vi "rsidr_core_global.vi"() -> ()   [LabVIEW 2015, in "Rohde&Schwarz CMP LR WPAN Measurement.lvlib"]
doc: "This Global variable contains driver's:\n- Attributes\n- Range Tables\n- Repeated Capabilities"
uses:
  <instrlib>/Rohde&Schwarz CMP LR WPAN Measurement/Rohde&Schwarz CMP LR WPAN Measurement.lvlib
  <instrlib>/Rohde&Schwarz CMP LR WPAN Measurement/Private/rsidr_core.llb/type_Input_Format_Attribute.ctl
  <instrlib>/Rohde&Schwarz CMP LR WPAN Measurement/Private/rsidr_core.llb/type_Input_Format_RangeTable.ctl
  <instrlib>/Rohde&Schwarz CMP LR WPAN Measurement/Private/rsidr_core.llb/type_Input_Format_RepCap.ctl
  <instrlib>/Rohde&Schwarz CMP LR WPAN Measurement/Private/rsidr_core.llb/rsidr_core.lvlib
panel:
  in  "Repeated Capabilities":T1[](array[typedef])=[{"repCapName"="instance", "indetifiers"=["i0", "i1", "i2", "i3", "i4", "i5", "i6", "i7", "i8", "i9", "i10", "i11", "i12", "i13", "i14", "i15", "i16", "i17", "i18", "i19", "i20", "i21", "i22", "i23", "i24", "i25", "i26", "i27", "i28", "i29", "i30", "i31", "i32"], "cmdValues"=["", "1", "2", "3", "4", "5", "6", "7", "8", "9", "10", "11", "12", "13", "14", "15", "16", "17", "18", "19", "20", "21", "22", "23", "24", "25", "26", "27", "28", "29", "30", "31", "32"]}]
  in  "Range Tables":T2[](array[typedef])=[{"Type"=0, "Name"="rscmplrwm_rngExternalAttenuation", "Entries"=[{"Name"="", "Value 1"=-50.0, "Value 2"=90.0, "Command"=""}]}, {"Type"=0, "Name"="rscmplrwm_rngFrequency", "Entries"=[{"Name"="", "Value 1"=4000000000.0, "Value 2"=20000000000.0, "Command"=""}]}, {"Type"=2, "Name"="rscmplrwm_rngRepetitionMode", "Entries"=[{"Name"="Single shot measurement", "Value 1"=0.0, "Value 2"=0.0, "Command"="SING"}, {"Name"="Continuous measurement", "Value 1"=1.0, "Value 2"=0.0, "Command"="CONT"}]}, {"Type"=2, "Name"="rscmplrwm_rngMultiEvalStopCondition", "Entries"=[{"Name"="None", "Value 1"=0.0, "Value 2"=0.0, "Command"="NONE"}, {"Name"="LimitFailure", "Value 1"=1.0, "Value 2"=0.0, "Command"="SLF"}]}, {"Type"=0, "Name"="rscmplrwm_rngMultiEvalModulationStatisticCount", "Entries"=[{"Name"="", "Value 1"=1.0, "Value 2"=1000.0, "Command"=""}]}, {"Type"=0, "Name"="rscmplrwm_rngMultiEvalPowerStatisticCount", "Entries"=[{"Name"="", "Value 1"=1.0, "Value 2"=1000.0, "Command"=""}]}, {"Type"=0, "Name"="rscmplrwm_rngMultiEvalSpectrumStatisticCount", "Entries"=[{"Name"="", "Value 1"=1.0, "Value 2"=1000.0, "Command"=""}]}, {"Type"=0, "Name"="rscmplrwm_rngMultiEvalMinimumTriggerGap", "Entries"=[{"Name"="", "Value 1"=0.0, "Value 2"=0.01, "Command"=""}]}, {"Type"=0, "Name"="rscmplrwm_rngMultiEvalTriggerTimeout", "Entries"=[{"Name"="", "Value 1"=0.01, "Value 2"=167772.1, "Command"=""}]}, {"Type"=0, "Name"="rscmplrwm_rngMultiEvalTriggerThreshold", "Entries"=[{"Name"="", "Value 1"=-50.0, "Value 2"=0.0, "Command"=""}]}, {"Type"=2, "Name"="rscmplrwm_rngModulationType", "Entries"=[{"Name"="2450 MHz, OQPSK", "Value 1"=0.0, "Value 2"=0.0, "Command"="OQ24"}]}, {"Type"=2, "Name"="rscmplrwm_rngSignalPath", "Entries"=[{"Name"="Port1.IFIn", "Value 1"=1.0, "Value 2"=0.0, "Command"="\"Port1.IFIn\""}, {"Name"="Port2.IFIn", "Value 1"=2.0, "Value 2"=0.0, "Command"="\"Port2.IFIn\""}, {"Name"="Port3.IFIn", "Value 1"=3.0, "Value 2"=0.0, "Command"="\"Port3.IFIn\""}]}, {"Type"=2, "Name"="rscmplrwm_rngResultType", "Entries"=[{"Name"="Current", "Value 1"=0.0, "Value 2"=0.0, "Command"="CURR"}, {"Name"="Average", "Value 1"=1.0, "Value 2"=0.0, "Command"="AVER"}, {"Name"="Extreme", "Value 1"=2.0, "Value 2"=0.0, "Command"="EXT"}, {"Name"="Standard Deviation", "Value 1"=3.0, "Value 2"=0.0, "Command"="SDEV"}, {"Name"="Maximum", "Value 1"=4.0, "Value 2"=0.0, "Command"="MAX"}, {"Name"="Minimum", "Value 1"=5.0, "Value 2"=0.0, "Command"="MIN"}]}, {"Type"=2, "Name"="rscmplrwm_rngLimitCheckResults", "Entries"=[{"Name"="Pass", "Value 1"=0.0, "Value 2"=0.0, "Command"="OK"}, {"Name"="Failed Upper", "Value 1"=1.0, "Value 2"=0.0, "Command"="ULEU"}, {"Name"="Failed Lower", "Value 1"=2.0, "Value 2"=0.0, "Command"="ULEL"}, {"Name"="Overflow", "Value 1"=3.0, "Value 2"=0.0, "Command"="OFL"}, {"Name"="Underflow", "Value 1"=4.0, "Value 2"=0.0, "Command"="UFL"}, {"Name"="Invalid", "Value 1"=5.0, "Value 2"=0.0, "Command"="INV"}, {"Name"="Not A Value", "Value 1"=6.0, "Value 2"=0.0, "Command"="NAV"}, {"Name"="Off", "Value 1"=7.0, "Value 2"=0.0, "Command"="OFF"}, {"Name"="Not Capable", "Value 1"=8.0, "Value 2"=0.0, "Command"="NCAP"}]}, {"Type"=2, "Name"="rscmplrwm_rngSyncState", "Entries"=[{"Name"="Pending", "Value 1"=0.0, "Value 2"=0.0, "Command"="PEND"}, {"Name"="Adjusted", "Value 1"=1.0, "Value 2"=0.0, "Command"="ADJ"}, {"Name"="Invalid", "Value 1"=2.0, "Value 2"=0.0, "Command"="INV"}]}, {"Type"=2, "Name"="rscmplrwm_rngResourceState", "Entries"=[{"Name"="No Resources", "Value 1"=0.0, "Value 2"=0.0, "Command"="QUE"}, {"Name"="Active", "Value 1"=1.0, "Value 2"=0.0, "Command"="ACT"}, {"Name"="Invalid", "Value 1"=2.0, "Value 2"=0.0, "Command"="INV"}]}, {"Type"=2, "Name"="rscmplrwm_rngMainState", "Entries"=[{"Name"="Off", "Value 1"=0.0, "Value 2"=0.0, "Command"="OFF"}, {"Name"="Run", "Value 1"=1.0, "Value 2"=0.0, "Command"="RUN"}, {"Name"="Ready", "Value 1"=2.0, "Value 2"=0.0, "Command"="RDY"}]}] {"Type" items=["Range", "Coerced", "Discrete"]}
  in  "Attributes":T3[](array[typedef])=[{"Level"=1, "Class Only"=TRUE, "Identifier"="", "Descriptive Name"="Configuration", "Data Type"=0, "Command"="", "Access"=0, "Range Table"="", "Read Callback"="", "Write Callback"="", "Supported Models"="", "Instrument Options"="", "Flags"=0, "Help"="Contains attributes for configuring LR-WPAN Measurement."}, {"Level"=2, "Class Only"=FALSE, "Identifier"="RSCMPLRWM_ATTR_SIGNAL_PATH", "Descriptive Name"="Signal Path", "Data Type"=0, "Command"="ROUT:WPAN:MEAS{instance}:SPAT", "Access"=2, "Range Table"="rscmplrwm_rngSignalPath", "Read Callback"="", "Write Callback"="", "Supported Models"="", "Instrument Options"="", "Flags"=0, "Help"="Selects the signal path for the measured RF signal.\nValid Values: Port1.IFln, Port2.IFln, Port3.IFln\n\nAvailable Repeated Capabilities:\ninstance: i0, i1, i2, i3, i4, i5, i6, i7, i8, i9, i10, i11, i12, i13, i14, i15, i16, i17, i18, i19, i20, i21, i22, i23, i24, i25, i26, i27, i28, i29, i30, i31, i32\r\n\nRemote-control command(s):\nROUTe:WPAN:MEAS<i>:SPATh"}, {"Level"=2, "Class Only"=FALSE, "Identifier"="RSCMPLRWM_ATTR_SIGNAL_PATH_CATALOG", "Descriptive Name"="Signal Path Catalog", "Data Type"=2, "Command"="CAT:WPAN:MEAS{instance}:SPAT?", "Access"=0, "Range Table"="", "Read Callback"="", "Write Callback"="", "Supported Models"="", "Instrument Options"="", "Flags"=0, "Help"="Returns the names of the available signal paths.\n\nReturned values: Comma-separated list of strings, one string per signal path\n\nAvailable Repeated Capabilities:\ninstance: i0, i1, i2, i3, i4, i5, i6, i7, i8, i9, i10, i11, i12, i13, i14, i15, i16, i17, i18, i19, i20, i21, i22, i23, i24, i25, i26, i27, i28, i29, i30, i31, i32\r\n\nRemote-control command(s):\nCATalog:WPAN:MEAS<i>:SPATh<stream>?"}, {"Level"=2, "Class Only"=FALSE, "Identifier"="RSCMPLRWM_ATTR_FREQUENCY", "Descriptive Name"="Frequency", "Data Type"=1, "Command"="CONF:WPAN:MEAS{instance}:RFS:FREQ", "Access"=2, "Range Table"="rscmplrwm_rngFrequency", "Read Callback"="", "Write Callback"="", "Supported Models"="", "Instrument Options"="", "Flags"=0, "Help"="Selects the center frequency of the RF analyzer.\n\nAvailable Repeated Capabilities:\ninstance: i0, i1, i2, i3, i4, i5, i6, i7, i8, i9, i10, i11, i12, i13, i14, i15, i16, i17, i18, i19, i20, i21, i22, i23, i24, i25, i26, i27, i28, i29, i30, i31, i32\r\n\nRemote-control command(s):\nCONFigure:WPAN:MEAS<i>:RFSettings:FREQuency"}, {"Level"=2, "Class Only"=FALSE, "Identifier"="RSCMPLRWM_ATTR_EXPECTED_NOMINAL_POWER", "Descriptive Name"="Expected Nominal Power", "Data Type"=1, "Command"="CONF:WPAN:MEAS{instance}:RFS:ENP", "Access"=2, "Range Table"="", "Read Callback"="", "Write Callback"="", "Supported Models"="", "Instrument Options"="", "Flags"=0, "Help"="Sets the expected nominal power of the measured RF signal.\n\nAvailable Repeated Capabilities:\ninstance: i0, i1, i2, i3, i4, i5, i6, i7, i8, i9, i10, i11, i12, i13, i14, i15, i16, i17, i18, i19, i20, i21, i22, i23, i24, i25, i26, i27, i28, i29, i30, i31, i32\r\n\nRemote-control command(s):\nCONFigure:WPAN:MEAS<i>:RFSettings:ENPower"}, {"Level"=2, "Class Only"=FALSE, "Identifier"="RSCMPLRWM_ATTR_EXTERNAL_ATTENUATION", "Descriptive Name"="External Attenuation", "Data Type"=1, "Command"="CONF:WPAN:MEAS{instance}:RFS:EATT", "Access"=2, "Range Table"="rscmplrwm_rngExternalAttenuation", "Read Callback"="", "Write Callback"="", "Supported Models"="", "Instrument Options"="", "Flags"=0, "Help"="Defines an external attenuation (or gain, if the value is negative)  to be applied to the input connector.\n\nAvailable Repeated Capabilities:\ninstance: i0, i1, i2, i3, i4, i5, i6, i7, i8, i9, i10, i11, i12, i13, i14, i15, i16, i17, i18, i19, i20, i21, i22, i23, i24, i25, i26, i27, i28, i29, i30, i31, i32\r\n\nRemote-control command(s):\nCONFigure:WPAN:MEAS<i>:RFSettings:EATTenuation"}, {"Level"=2, "Class Only"=FALSE, "Identifier"="RSCMPLRWM_ATTR_USER_MARGIN", "Descriptive Name"="User Margin", "Data Type"=1, "Command"="CONF:WPAN:MEAS{instance}:RFS:UMAR", "Access"=2, "Range Table"="", "Read Callback"="", "Write Callback"="", "Supported Models"="", "Instrument Options"="", "Flags"=0, "Help"="Sets the margin that the measurement adds to the expected nominal power to determine the reference level. The reference level minus the external input attenuation must be within the power range of the selected input connector; refer to the data sheet.\n\nAvailable Repeated Capabilities:\ninstance: i0, i1, i2, i3, i4, i5, i6, i7, i8, i9, i10, i11, i12, i13, i14, i15, i16, i17, i18, i19, i20, i21, i22, i23, i24, i25, i26, i27, i28, i29, i30, i31, i32\r\n\nRemote-control command(s):\nCONFigure:WPAN:MEAS<i>:RFSettings:UMARgin"}, {"Level"=2, "Class Only"=FALSE, "Identifier"="RSCMPLRWM_ATTR_MODULATION_TYPE", "Descriptive Name"="Modulation Type", "Data Type"=0, "Command"="CONF:WPAN:MEAS{instance}:ISIG:MTYP", "Access"=2, "Range Table"="rscmplrwm_rngModulationType", "Read Callback"="", "Write Callback"="", "Supported Models"="", "Instrument Options"="", "Flags"=0, "Help"="Specifies the modulation of the measured packets.\n\nAvailable Repeated Capabilities:\ninstance: i0, i1, i2, i3, i4, i5, i6, i7, i8, i9, i10, i11, i12, i13, i14, i15, i16, i17, i18, i19, i20, i21, i22, i23, i24, i25, i26, i27, i28, i29, i30, i31, i32\r\n\nRemote-control command(s):\nCONFigure:WPAN:MEAS<i>:ISIGnal:MTYPe"}, {"Level"=1, "Class Only"=TRUE, "Identifier"="", "Descriptive Name"="Multi Eval Meas", "Data Type"=0, "Command"="", "Access"=0, "Range Table"="", "Read Callback"="", "Write Callback"="", "Supported Models"="", "Instrument Options"="", "Flags"=0, "Help"="The attributes for the LR-WPAN multi-evaluation measurement are divided into the groups listed below. The general measurement settings also affect the measurement."}, {"Level"=2, "Class Only"=TRUE, "Identifier"="", "Descriptive Name"="Control and States", "Data Type"=0, "Command"="", "Access"=0, "Range Table"="", "Read Callback"="", "Write Callback"="", "Supported Models"="", "Instrument Options"="", "Flags"=0, "Help"="Measurement control and states."}, {"Level"=3, "Class Only"=FALSE, "Identifier"="RSCMPLRWM_ATTR_MULTIEVAL_INIT", "Descriptive Name"="MultiEval Init", "Data Type"=4, "Command"="INIT:WPAN:MEAS{instance}:MEV", "Access"=1, "Range Table"="", "Read Callback"="", "Write Callback"="", "Supported Models"="", "Instrument Options"="", "Flags"=1, "Help"="Starts or restarts the measurement, the measurement enters the 'RUN' state.\n\nAvailable Repeated Capabilities:\ninstance: i0, i1, i2, i3, i4, i5, i6, i7, i8, i9, i10, i11, i12, i13, i14, i15, i16, i17, i18, i19, i20, i21, i22, i23, i24, i25, i26, i27, i28, i29, i30, i31, i32\r\n\nRemote-control command(s):\nINITiate:WPAN:MEAS<i>:MEValuation"}, {"Level"=3, "Class Only"=FALSE, "Identifier"="RSCMPLRWM_ATTR_MULTIEVAL_ABORT", "Descriptive Name"="MultiEval Abort", "Data Type"=4, "Command"="ABOR:WPAN:MEAS{instance}:MEV", "Access"=1, "Range Table"="", "Read Callback"="", "Write Callback"="", "Supported Models"="", "Instrument Options"="", "Flags"=0, "Help"="Causes a running measurement to stop immediately, the measurement enters the 'OFF' state. All measurement values are set to NAV. Allocated resources are released.\n\nAvailable Repeated Capabilities:\ninstance: i0, i1, i2, i3, i4, i5, i6, i7, i8, i9, i10, i11, i12, i13, i14, i15, i16, i17, i18, i19, i20, i21, i22, i23, i24, i25, i26, i27, i28, i29, i30, i31, i32\r\n\nRemote-control command(s):\nABORt:WPAN:MEAS<i>:MEValuation"}, {"Level"=3, "Class Only"=FALSE, "Identifier"="RSCMPLRWM_ATTR_MULTIEVAL_STOP", "Descriptive Name"="MultiEval Stop", "Data Type"=4, "Command"="STOP:WPAN:MEAS{instance}:MEV", "Access"=1, "Range Table"="", "Read Callback"="", "Write Callback"="", "Supported Models"="", "Instrument Options"="", "Flags"=0, "Help"="Causes a running measurement to stop immediately: the measurement enters the 'RDY' state. Measurement results are kept. The resources remain allocated to the measurement.\n\nAvailable Repeated Capabilities:\ninstance: i0, i1, i2, i3, i4, i5, i6, i7, i8, i9, i10, i11, i12, i13, i14, i15, i16, i17, i18, i19, i20, i21, i22, i23, i24, i25, i26, i27, i28, i29, i30, i31, i32\r\n\nRemote-control command(s):\nSTOP:WPAN:MEAS<i>:MEValuation"}, {"Level"=3, "Class Only"=FALSE, "Identifier"="RSCMPLRWM_ATTR_HIDDEN_MULTIEVAL_STATE", "Descriptive Name"="MultiEval State", "Data Type"=6, "Command"="FETC:WPAN:MEAS{instance}:MEV:STAT:ALL?", "Access"=0, "Range Table"="", "Read Callback"="", "Write Callback"="", "Supported Models"="", "Instrument Options"="", "Flags"=8, "Help"="Queries the main measurement state and the measurement substates. Both measurement substates are relevant for running measurements only. Use FETCh:...:STATe? to query the main measurement state only. Use INITiate..., STOP..., ABORt... to change the measurement state.\n\nAvailable Repeated Capabilities:\ninstance: i0, i1, i2, i3, i4, i5, i6, i7, i8, i9, i10, i11, i12, i13, i14, i15, i16, i17, i18, i19, i20, i21, i22, i23, i24, i25, i26, i27, i28, i29, i30, i31, i32\r\n\nRemote-control command(s):\nFETCh:WPAN:MEAS<i>:MEValuation:STATe:ALL?"}, {"Level"=2, "Class Only"=TRUE, "Identifier"="", "Descriptive Name"="Configuration", "Data Type"=0, "Command"="", "Access"=0, "Range Table"="", "Read Callback"="", "Write Callback"="", "Supported Models"="", "Instrument Options"="", "Flags"=0, "Help"="Multi Evaluation measurement configuration attributes."}, {"Level"=3, "Class Only"=FALSE, "Identifier"="RSCMPLRWM_ATTR_HIDDEN_MULTIEVAL_ALL_RESULTS_ENABLED", "Descriptive Name"="MultiEval All Results Enabled", "Data Type"=6, "Command"="CONF:WPAN:MEAS{instance}:MEV:RES", "Access"=2, "Range Table"="", "Read Callback"="", "Write Callback"="", "Supported Models"="", "Instrument Options"="", "Flags"=8, "Help"="Enables or disables the evaluation of results in the multi-evaluation measurement. Combines all other CONFigure:WPAN:MEAS<i>:MEValuation:RESult... commands.\n\nSyntax:\nCONFigure:WPAN:MEAS<i>:MEValuation:RESult[:ALL] <PvT>, <PowerScalars>, <EVMChip>, <ModScalars>, <PowSpecDensity>[, <IQConstellation>]\n\nParameters:\n<PvT>   - Power vs time\nON: evaluate results\nOFF: do not evaluate results\nDefault value: ON\n\n<PowerScalars>   - Statistical power results\nOFF | ON\nDefault value: ON\n\n<EVMChip>   - Error vector magnitude vs chip\nOFF | ON\nDefault value: ON\n\n<ModScalars>   - Statistical modulation results\nOFF | ON\nDefault value: ON\n\n<PowSpecDensity>   - Power spectral density results\nOFF | ON\nDefault value: ON\n\n<IQConstellation>   - IQ constellation results\nOFF | ON\nDefault value: ON\n\nAvailable Repeated Capabilities:\ninstance: i0, i1, i2, i3, i4, i5, i6, i7, i8, i9, i10, i11, i12, i13, i14, i15, i16, i17, i18, i19, i20, i21, i22, i23, i24, i25, i26, i27, i28, i29, i30, i31, i32\r\n\nRemote-control command(s):\nCONFigure:WPAN:MEAS<i>:MEValuation:RESult[:ALL]"}, {"Level"=3, "Class Only"=TRUE, "Identifier"="", "Descriptive Name"="Control", "Data Type"=0, "Command"="", "Access"=0, "Range Table"="", "Read Callback"="", "Write Callback"="", "Supported Models"="", "Instrument Options"="", "Flags"=0, "Help"="General measurement control settings."}, {"Level"=4, "Class Only"=FALSE, "Identifier"="RSCMPLRWM_ATTR_MULTIEVAL_REPETITION", "Descriptive Name"="MultiEval Repetition", "Data Type"=0, "Command"="CONF:WPAN:MEAS{instance}:MEV:REP", "Access"=2, "Range Table"="rscmplrwm_rngRepetitionMode", "Read Callback"="", "Write Callback"="", "Supported Models"="", "Instrument Options"="", "Flags"=0, "Help"="Specifies the repetition mode of the measurement. The repetition mode specifies whether the measurement is stopped after a single shot or repeated continuously. Use CONFigure:..:MEAS<i>:...:SCOunt to determine the number of measurement intervals per single shot.\n\nAvailable Repeated Capabilities:\ninstance: i0, i1, i2, i3, i4, i5, i6, i7, i8, i9, i10, i11, i12, i13, i14, i15, i16, i17, i18, i19, i20, i21, i22, i23, i24, i25, i26, i27, i28, i29, i30, i31, i32\r\n\nRemote-control command(s):\nCONFigure:WPAN:MEAS<i>:MEValuation:REPetition"}, {"Level"=4, "Class Only"=FALSE, "Identifier"="RSCMPLRWM_ATTR_MULTIEVAL_STOP_CONDITION", "Descriptive Name"="MultiEval Stop Condition", "Data Type"=0, "Command"="CONF:WPAN:MEAS{instance}:MEV:SCON", "Access"=2, "Range Table"="rscmplrwm_rngMultiEvalStopCondition", "Read Callback"="", "Write Callback"="", "Supported Models"="", "Instrument Options"="", "Flags"=0, "Help"="Qualifies whether the measurement is stopped after a failed limit check or continued. SLFail means that the measurement is stopped and reaches the RDY state when one of the results exceeds the limits.\n\nAvailable Repeated Capabilities:\ninstance: i0, i1, i2, i3, i4, i5, i6, i7, i8, i9, i10, i11, i12, i13, i14, i15, i16, i17, i18, i19, i20, i21, i22, i23, i24, i25, i26, i27, i28, i29, i30, i31, i32\r\n\nRemote-control command(s):\nCONFigure:WPAN:MEAS<i>:MEValuation:SCONdition"}, {"Level"=4, "Class Only"=FALSE, "Identifier"="RSCMPLRWM_ATTR_MULTIEVAL_MEASURE_ON_EXCEPTION_ENABLED", "Descriptive Name"="MultiEval Measure On Exception Enabled", "Data Type"=3, "Command"="CONF:WPAN:MEAS{instance}:MEV:MOEX", "Access"=2, "Range Table"="", "Read Callback"="", "Write Callback"="", "Supported Models"="", "Instrument Options"="", "Flags"=0, "Help"="Specifies whether measurement results that are identified as faulty or inaccurate are rejected\n\nAvailable Repeated Capabilities:\ninstance: i0, i1, i2, i3, i4, i5, i6, i7, i8, i9, i10, i11, i12, i13, i14, i15, i16, i17, i18, i19, i20, i21, i22, i23, i24, i25, i26, i27, i28, i29, i30, i31, i32\r\n\nRemote-control command(s):\nCONFigure:WPAN:MEAS<i>:MEValuation:MOEXception"}, {"Level"=4, "Class Only"=FALSE, "Identifier"="RSCMPLRWM_ATTR_MULTIEVAL_TIMEOUT", "Descriptive Name"="MultiEval Timeout", "Data Type"=1, "Command"="CONF:WPAN:MEAS{instance}:MEV:TOUT", "Access"=2, "Range Table"="", "Read Callback"="", "Write Callback"="", "Supported Models"="", "Instrument Options"="", "Flags"=0, "Help"="Defines a timeout for the measurement. The timer is started when the measurement is initiated via a READ or INIT command. It is not started if the measurement is initiated manually. When the measurement has completed the first measurement cycle (first single shot), the statistical depth is reached and the timer is reset. If the first measurement cycle has not been completed when the timer expires, the measurement is stopped. The measurement state changes to RDY. The reliability indicator is set to 1, indicating that a measurement timeout occurred. Still running READ, FETCh or CALCulate commands are completed, returning the available results. At least for some results, there are no values at all or the statistical depth has not been reached.\nA timeout of 0 s corresponds to an infinite measurement timeout.\n\nAvailable Repeated Capabilities:\ninstance: i0, i1, i2, i3, i4, i5, i6, i7, i8, i9, i10, i11, i12, i13, i14, i15, i16, i17, i18, i19, i20, i21, i22, i23, i24, i25, i26, i27, i28, i29, i30, i31, i32\r\n\nRemote-control command(s):\nCONFigure:WPAN:MEAS<i>:MEValuation:TOUT"}, {"Level"=3, "Class Only"=TRUE, "Identifier"="", "Descriptive Name"="TX Measurement", "Data Type"=0, "Command"="", "Access"=0, "Range Table"="", "Read Callback"="", "Write Callback"="", "Supported Models"="", "Instrument Options"="", "Flags"=0, "Help"="Enables or disables the evaluation of the individual measurement results."}, {"Level"=4, "Class Only"=FALSE, "Identifier"="RSCMPLRWM_ATTR_MULTIEVAL_MODULATION_SCALAR_ENABLED", "Descriptive Name"="MultiEval Modulation Scalar Enabled", "Data Type"=3, "Command"="CONF:WPAN:MEAS{instance}:MEV:RES:MSC", "Access"=2, "Range Table"="", "Read Callback"="", "Write Callback"="", "Supported Models"="", "Instrument Options"="", "Flags"=0, "Help"="Enables or disables the evaluation of Modulation Scalar results in the multi-evaluation measurement.\n\nAvailable Repeated Capabilities:\ninstance: i0, i1, i2, i3, i4, i5, i6, i7, i8, i9, i10, i11, i12, i13, i14, i15, i16, i17, i18, i19, i20, i21, i22, i23, i24, i25, i26, i27, i28, i29, i30, i31, i32\r\n\nRemote-control command(s):\nCONFigure:WPAN:MEAS<i>:MEValuation:RESult:MSCalar"}, {"Level"=4, "Class Only"=FALSE, "Identifier"="RSCMPLRWM_ATTR_MULTIEVAL_POWER_SCALAR_ENABLED", "Descriptive Name"="MultiEval Power Scalar Enabled", "Data Type"=3, "Command"="CONF:WPAN:MEAS{instance}:MEV:RES:PSC", "Access"=2, "Range Table"="", "Read Callback"="", "Write Callback"="", "Supported Models"="", "Instrument Options"="", "Flags"=0, "Help"="Enables or disables the evaluation of Power Scalar results in the multi-evaluation measurement.\n\nAvailable Repeated Capabilities:\ninstance: i0, i1, i2, i3, i4, i5, i6, i7, i8, i9, i10, i11, i12, i13, i14, i15, i16, i17, i18, i19, i20, i21, i22, i23, i24, i25, i26, i27, i28, i29, i30, i31, i32\r\n\nRemote-control command(s):\nCONFigure:WPAN:MEAS<i>:MEValuation:RESult:PSCalar"}, {"Level"=3, "Class Only"=TRUE, "Identifier"="", "Descriptive Name"="Modulation", "Data Type"=0, "Command"="", "Access"=0, "Range Table"="", "Read Callback"="", "Write Callback"="", "Supported Models"="", "Instrument Options"="", "Flags"=0, "Help"="Modulation control settings."}, {"Level"=4, "Class Only"=FALSE, "Identifier"="RSCMPLRWM_ATTR_MULTIEVAL_MODULATION_STATIC_COUNT", "Descriptive Name"="MultiEval Modulation Statistic Count", "Data Type"=0, "Command"="CONF:WPAN:MEAS{instance}:MEV:SCO:MOD", "Access"=2, "Range Table"="rscmplrwm_rngMultiEvalModulationStatisticCount", "Read Callback"="", "Write Callback"="", "Supported Models"="", "Instrument Options"="", "Flags"=0, "Help"="Specifies the statistic count of the measurement. The statistic count is equal to the number of measurement intervals per single shot.\n\nAvailable Repeated Capabilities:\ninstance: i0, i1, i2, i3, i4, i5, i6, i7, i8, i9, i10, i11, i12, i13, i14, i15, i16, i17, i18, i19, i20, i21, i22, i23, i24, i25, i26, i27, i28, i29, i30, i31, i32\r\n\nRemote-control command(s):\nCONFigure:WPAN:MEAS<i>:MEValuation:SCOunt:MODulation"}, {"Level"=4, "Class Only"=FALSE, "Identifier"="RSCMPLRWM_ATTR_MULTIEVAL_MODULATION_EVM_VS_CHIP_ENABLED", "Descriptive Name"="MultiEval Modulation EVM vs Chip Enabled", "Data Type"=3, "Command"="CONF:WPAN:MEAS{instance}:MEV:RES:EVMC", "Access"=2, "Range Table"="", "Read Callback"="", "Write Callback"="", "Supported Models"="", "Instrument Options"="", "Flags"=0, "Help"="Enables or disables the evaluation of EVM vs Chip results in the multi-evaluation measurement.\n\nAvailable Repeated Capabilities:\ninstance: i0, i1, i2, i3, i4, i5, i6, i7, i8, i9, i10, i11, i12, i13, i14, i15, i16, i17, i18, i19, i20, i21, i22, i23, i24, i25, i26, i27, i28, i29, i30, i31, i32\r\n\nRemote-control command(s):\nCONFigure:WPAN:MEAS<i>:MEValuation:RESult:EVMChip"}, {"Level"=4, "Class Only"=FALSE, "Identifier"="RSCMPLRWM_ATTR_MULTIEVAL_MODULATION_IQ_ENABLED", "Descriptive Name"="MultiEval Modulation IQ Enabled", "Data Type"=3, "Command"="CONF:WPAN:MEAS{instance}:MEV:RES:IQ", "Access"=2, "Range Table"="", "Read Callback"="", "Write Callback"="", "Supported Models"="", "Instrument Options"="", "Flags"=0, "Help"="Enables or disables the evaluation of IQ results in the multi-evaluation measurement.\n\nAvailable Repeated Capabilities:\ninstance: i0, i1, i2, i3, i4, i5, i6, i7, i8, i9, i10, i11, i12, i13, i14, i15, i16, i17, i18, i19, i20, i21, i22, i23, i24, i25, i26, i27, i28, i29, i30, i31, i32\r\n\nRemote-control command(s):\nCONFigure:WPAN:MEAS<i>:MEValuation:RESult:IQ"}, {"Level"=4, "Class Only"=FALSE, "Identifier"="RSCMPLRWM_ATTR_MULTIEVAL_MODULATION_PHASE_TRACKING", "Descriptive Name"="MultiEval Modulation Phase Tracking", "Data Type"=3, "Command"="CONF:WPAN:MEAS{instance}:MEV:MOD:PTR", "Access"=2, "Range Table"="", "Read Callback"="", "Write Callback"="", "Supported Models"="", "Instrument Options"="", "Flags"=0, "Help"="Enables or disables phase tracking for modulation results.\n\nAvailable Repeated Capabilities:\ninstance: i0, i1, i2, i3, i4, i5, i6, i7, i8, i9, i10, i11, i12, i13, i14, i15, i16, i17, i18, i19, i20, i21, i22, i23, i24, i25, i26, i27, i28, i29, i30, i31, i32\r\n\nRemote-control command(s):\nCONFigure:WPAN:MEAS<i>:MEValuation:MODulation:PTRacking"}, {"Level"=3, "Class Only"=TRUE, "Identifier"="", "Descriptive Name"="Spectrum", "Data Type"=0, "Command"="", "Access"=0, "Range Table"="", "Read Callback"="", "Write Callback"="", "Supported Models"="", "Instrument Options"="", "Flags"=0, "Help"="Spectrum Measurement Settings."}, {"Level"=4, "Class Only"=FALSE, "Identifier"="RSCMPLRWM_ATTR_MULTIEVAL_SPECTRUM_STATIC_COUNT", "Descriptive Name"="MultiEval Spectrum Statistic Count", "Data Type"=0, "Command"="CONF:WPAN:MEAS{instance}:MEV:SCO:SPEC", "Access"=2, "Range Table"="rscmplrwm_rngMultiEvalSpectrumStatisticCount", "Read Callback"="", "Write Callback"="", "Supported Models"="", "Instrument Options"="", "Flags"=0, "Help"="Specifies the statistic count of the measurement. The statistic count is equal to the number of measurement intervals per single shot.\n\nAvailable Repeated Capabilities:\ninstance: i0, i1, i2, i3, i4, i5, i6, i7, i8, i9, i10, i11, i12, i13, i14, i15, i16, i17, i18, i19, i20, i21, i22, i23, i24, i25, i26, i27, i28, i29, i30, i31, i32\r\n\nRemote-control command(s):\nCONFigure:WPAN:MEAS<i>:MEValuation:SCOunt:SPECtrum"}, {"Level"=4, "Class Only"=FALSE, "Identifier"="RSCMPLRWM_ATTR_MULTIEVAL_SPECTRUM_POWER_SPECTRAL_DENSITY_ENABLED", "Descriptive Name"="MultiEval Spectrum Power Spectral Density Enabled", "Data Type"=3, "Command"="CONF:WPAN:MEAS{instance}:MEV:RES:SPEC", "Access"=2, "Range Table"="", "Read Callback"="", "Write Callback"="", "Supported Models"="", "Instrument Options"="", "Flags"=0, "Help"="Enables or disables the evaluation of Power Spectral Density results in the multi-evaluation measurement.\n\nAvailable Repeated Capabilities:\ninstance: i0, i1, i2, i3, i4, i5, i6, i7, i8, i9, i10, i11, i12, i13, i14, i15, i16, i17, i18, i19, i20, i21, i22, i23, i24, i25, i26, i27, i28, i29, i30, i31, i32\r\n\nRemote-control command(s):\nCONFigure:WPAN:MEAS<i>:MEValuation:RESult:SPECtrum"}, {"Level"=3, "Class Only"=TRUE, "Identifier"="", "Descriptive Name"="Power", "Data Type"=0, "Command"="", "Access"=0, "Range Table"="", "Read Callback"="", "Write Callback"="", "Supported Models"="", "Instrument Options"="", "Flags"=0, "Help"="Power vs Time Measurement Setting"}, {"Level"=4, "Class Only"=FALSE, "Identifier"="RSCMPLRWM_ATTR_MULTIEVAL_PVT_STATISTIC_COUNT", "Descriptive Name"="MultiEval PVT Statistic Count", "Data Type"=0, "Command"="CONF:WPAN:MEAS{instance}:MEV:SCO:PVT", "Access"=2, "Range Table"="rscmplrwm_rngMultiEvalPowerStatisticCount", "Read Callback"="", "Write Callback"="", "Supported Models"="", "Instrument Options"="", "Flags"=0, "Help"="Specifies the statistic count of the measurement. The statistic count is equal to the number of measurement intervals per single shot.\n\nAvailable Repeated Capabilities:\ninstance: i0, i1, i2, i3, i4, i5, i6, i7, i8, i9, i10, i11, i12, i13, i14, i15, i16, i17, i18, i19, i20, i21, i22, i23, i24, i25, i26, i27, i28, i29, i30, i31, i32\r\n\nRemote-control command(s):\nCONFigure:WPAN:MEAS<i>:MEValuation:SCOunt:PVTime"}, {"Level"=4, "Class Only"=FALSE, "Identifier"="RSCMPLRWM_ATTR_MULTIEVAL_PVT_ENABLED", "Descriptive Name"="MultiEval PVT Enabled", "Data Type"=3, "Command"="CONF:WPAN:MEAS{instance}:MEV:RES:PVT", "Access"=2, "Range Table"="", "Read Callback"="", "Write Callback"="", "Supported Models"="", "Instrument Options"="", "Flags"=0, "Help"="Enables or disables the evaluation of Power vs Time results in the multi-evaluation measurement.\n\nAvailable Repeated Capabilities:\ninstance: i0, i1, i2, i3, i4, i5, i6, i7, i8, i9, i10, i11, i12, i13, i14, i15, i16, i17, i18, i19, i20, i21, i22, i23, i24, i25, i26, i27, i28, i29, i30, i31, i32\r\n\nRemote-control command(s):\nCONFigure:WPAN:MEAS<i>:MEValuation:RESult:PVTime"}, {"Level"=2, "Class Only"=TRUE, "Identifier"="", "Descriptive Name"="Trigger", "Data Type"=0, "Command"="", "Access"=0, "Range Table"="", "Read Callback"="", "Write Callback"="", "Supported Models"="", "Instrument Options"="", "Flags"=0, "Help"="Trigger settings"}, {"Level"=3, "Class Only"=FALSE, "Identifier"="RSCMPLRWM_ATTR_MULTIEVAL_TRIGGER_SOURCE", "Descriptive Name"="MultiEval Trigger Source", "Data Type"=2, "Command"="TRIG:WPAN:MEAS{instance}:MEV:SOUR", "Access"=2, "Range Table"="", "Read Callback"="", "Write Callback"="", "Supported Models"="", "Instrument Options"="", "Flags"=0, "Help"="Selects the source of the trigger events. Some values are always available. They are listed below. Depending on the installed options, additional values are available. You can query a list of all supported values via TRIGger:...:CATalog:SOURce?.\n\nAvailable Repeated Capabilities:\ninstance: i0, i1, i2, i3, i4, i5, i6, i7, i8, i9, i10, i11, i12, i13, i14, i15, i16, i17, i18, i19, i20, i21, i22, i23, i24, i25, i26, i27, i28, i29, i30, i31, i32\r\n\nRemote-control command(s):\nTRIGger:WPAN:MEAS<i>:MEValuation:SOURce"}, {"Level"=3, "Class Only"=FALSE, "Identifier"="RSCMPLRWM_ATTR_HIDDEN_MULTIEVAL_TRIGGER_SOURCE_CATALOG", "Descriptive Name"="MultiEval Trigger Source Catalog", "Data Type"=6, "Command"="TRIG:WPAN:MEAS{instance}:MEV:CAT:SOUR?", "Access"=0, "Range Table"="", "Read Callback"="", "Write Callback"="", "Supported Models"="", "Instrument Options"="", "Flags"=8, "Help"="Lists all trigger source values that can be set using TRIGger:WPAN:MEAS<i>:MEValuation:SOURce. Comma-separated list of all supported values. Each value is represented as a string.\n\nAvailable Repeated Capabilities:\ninstance: i0, i1, i2, i3, i4, i5, i6, i7, i8, i9, i10, i11, i12, i13, i14, i15, i16, i17, i18, i19, i20, i21, i22, i23, i24, i25, i26, i27, i28, i29, i30, i31, i32\r\n\nRemote-control command(s):\nTRIGger:WPAN:MEAS<i>:MEValuation:CATalog:SOURce?"}, {"Level"=3, "Class Only"=FALSE, "Identifier"="RSCMPLRWM_ATTR_MULTIEVAL_TRIGGER_THRESHOLD", "Descriptive Name"="MultiEval Trigger Threshold", "Data Type"=1, "Command"="TRIG:WPAN:MEAS{instance}:MEV:THReshold", "Access"=2, "Range Table"="rscmplrwm_rngMultiEvalTriggerThreshold", "Read Callback"="", "Write Callback"="", "Supported Models"="", "Instrument Options"="", "Flags"=0, "Help"="Defines the trigger threshold for the power trigger.\n\nAvailable Repeated Capabilities:\ninstance: i0, i1, i2, i3, i4, i5, i6, i7, i8, i9, i10, i11, i12, i13, i14, i15, i16, i17, i18, i19, i20, i21, i22, i23, i24, i25, i26, i27, i28, i29, i30, i31, i32\r\n\nRemote-control command(s):\nTRIGger:WPAN:MEAS<i>:MEValuation:THReshold"}, {"Level"=3, "Class Only"=FALSE, "Identifier"="RSCMPLRWM_ATTR_MULTIEVAL_TRIGGER_TIMEOUT_ENABLED", "Descriptive Name"="MultiEval Trigger Timeout Enabled", "Data Type"=3, "Command"="CONF:WPAN:MEAS{instance}:MEV:TRIG:TOUT", "Access"=2, "Range Table"="", "Read Callback"="", "Write Callback"="", "Supported Models"="", "Instrument Options"="", "Flags"=0, "Help"="Disables or enables timeout using the previous/default values\n\nAvailable Repeated Capabilities:\ninstance: i0, i1, i2, i3, i4, i5, i6, i7, i8, i9, i10, i11, i12, i13, i14, i15, i16, i17, i18, i19, i20, i21, i22, i23, i24, i25, i26, i27, i28, i29, i30, i31, i32\r\n\nRemote-control command(s):\nCONFigure:WPAN:MEAS<i>:MEValuation:TRIGger:TOUT"}, {"Level"=3, "Class Only"=FALSE, "Identifier"="RSCMPLRWM_ATTR_MULTIEVAL_TRIGGER_TIMEOUT", "Descriptive Name"="MultiEval Trigger Timeout", "Data Type"=1, "Command"="CONF:WPAN:MEAS{instance}:MEV:TRIG:TOUT", "Access"=2, "Range Table"="rscmplrwm_rngMultiEvalTriggerTimeout", "Read Callback"="", "Write Callback"="", "Supported Models"="", "Instrument Options"="", "Flags"=0, "Help"="Selects the maximum time that the measurement waits for a trigger event before it stops in remote control mode or indicates a trigger timeout in manual operation mode.\n\nAvailable Repeated Capabilities:\ninstance: i0, i1, i2, i3, i4, i5, i6, i7, i8, i9, i10, i11, i12, i13, i14, i15, i16, i17, i18, i19, i20, i21, i22, i23, i24, i25, i26, i27, i28, i29, i30, i31, i32\r\n\nRemote-control command(s):\nCONFigure:WPAN:MEAS<i>:MEValuation:TRIGger:TOUT"}, {"Level"=3, "Class Only"=FALSE, "Identifier"="RSCMPLRWM_ATTR_MULTIEVAL_MINIMUM_TRIGGER_GAP", "Descriptive Name"="MultiEval Minimum Trigger Gap", "Data Type"=1, "Command"="CONF:WPAN:MEAS{instance}:MEV:TRIG:MGAP", "Access"=2, "Range Table"="rscmplrwm_rngMultiEvalMinimumTriggerGap", "Read Callback"="", "Write Callback"="", "Supported Models"="", "Instrument Options"="", "Flags"=0, "Help"="Sets a minimum time during which the IF signal must be below the trigger threshold before the trigger is armed so that an IF power trigger event can be generated.\n\nAvailable Repeated Capabilities:\ninstance: i0, i1, i2, i3, i4, i5, i6, i7, i8, i9, i10, i11, i12, i13, i14, i15, i16, i17, i18, i19, i20, i21, i22, i23, i24, i25, i26, i27, i28, i29, i30, i31, i32\r\n\nRemote-control command(s):\nCONFigure:WPAN:MEAS<i>:MEValuation:TRIGger:MGAP"}, {"Level"=2, "Class Only"=TRUE, "Identifier"="", "Descriptive Name"="Limits", "Data Type"=0, "Command"="", "Access"=0, "Range Table"="", "Read Callback"="", "Write Callback"="", "Supported Models"="", "Instrument Options"="", "Flags"=0, "Help"="Multi Evaluation measurement limits attributes."}, {"Level"=3, "Class Only"=FALSE, "Identifier"="RSCMPLRWM_ATTR_HIDDEN_MULTIEVAL_EVM_ABSOLUTE_LIMIT", "Descriptive Name"="MultiEval EVM Absolute Limit", "Data Type"=6, "Command"="CONF:WPAN:MEAS{instance}:MEV:LIM:EVM:ABS", "Access"=2, "Range Table"="", "Read Callback"="", "Write Callback"="", "Supported Models"="", "Instrument Options"="", "Flags"=8, "Help"="Defines upper limits for the RMS and peak values of the absolute error vector magnitude (EVM).\n\nSyntax:\nCONFigure:WPAN:MEAS<i>:MEValuation:LIMit:EVM:ABSolute <RMS_EVM>, <PeakEVM>, <RMS_EVMEnabled>, <PeakEVM_Enabled>[, <RMS_SHRPHR>, <Peak_SHRPHR>, <RMS_Overall>, <Peak_Overall>, <RMS_SHRPHR_Enb>, <Pk_SHRPHR_Enb>, <RMSOverall_Enb>, <PkOverall_Enb>]\n\nParameters\n<1_RMS_EVM_PS>   - RMS EVM for PSDU portion\nRange: 0 - 100 %\nDefault value: 35 %\n\n<2_Peak_EVM_PS>   - Peak EVM for PSDU portion\nRange: 0 - 100 %\nDefault value: 35 %\n\n<3_RMS_PS_Enb>   - Disables | enables the RMS limit check for EVM within PSDU portion.\nOFF | ON\nDeafult value: ON\n\n<4_Peak_PS_Enb>   - Disables | enables the peak limit check for EVM within PSDU portion.\nOFF | ON\nDefault value: OFF\n\n<5_RMS_EVM_SP>   - RMS EVM for SHR + PHR portion\nRange: 0 % to 100 %\nDeaful value: 35 %\n\n<6_Peak_EVM_SP>   - Peak EVM for SHR + PHR portion\nRange: 0 % to 100 %\nDeaful value: 35 %\n\n<7_RMS_EVM_All>   - Overall RMS EVM for complete PPDU\nRange: 0 % to 100 %\nDeaful value: 35 %\n\n <8_Peak_EVM_All>   - Overall Peak EVM for complete PPDU\nRange: 0 % to 100 %\nDeaful value: 35 %\n\n<9_RMS_SP_Enb>   - Disables | enables the RMS limit check for EVM within SHR + PHR portion.\nOFF | ON\nDefault value: ON\n\n<10_Peak_SP_Enb>   - Disables | enables the peak limit check for EVM within SHR + PHR portion.\nOFF | ON\nDefault value: OFF\n\n<11_RMS_Sll_Enb>    - Disables | enables the RMS limit check for overall EVM for complete PPDU.\nOFF | ON\nDefault value: ON\n\n<12_Peak_All_Enb>   - Disables | enables the peak limit check for overall EVM for complete PPDU.\nOFF | ON\nDefault value: OFF\n\nAvailable Repeated Capabilities:\ninstance: i0, i1, i2, i3, i4, i5, i6, i7, i8, i9, i10, i11, i12, i13, i14, i15, i16, i17, i18, i19, i20, i21, i22, i23, i24, i25, i26, i27, i28, i29, i30, i31, i32\r\n\nRemote-control command(s):\nCONFigure:WPAN:MEAS<i>:MEValuation:LIMit:EVM:ABSolute"}, {"Level"=3, "Class Only"=FALSE, "Identifier"="RSCMPLRWM_ATTR_HIDDEN_MULTIEVAL_EVM_OFFSET_LIMIT", "Descriptive Name"="MultiEval EVM Offset Limit", "Data Type"=6, "Command"="CONF:WPAN:MEAS{instance}:MEV:LIM:EVM", "Access"=2, "Range Table"="", "Read Callback"="", "Write Callback"="", "Supported Models"="", "Instrument Options"="", "Flags"=8, "Help"="Defines upper limits for the RMS and peak values of the offset error vector magnitude (EVM).\n\nSyntax:\nCONFigure:WPAN:MEAS<i>:MEValuation:LIMit:EVM[:OFFSet] <RMS_EVM>, <PeakEVM>, <RMS_EVMEnabled>, <PeakEVM_Enabled>[, <RMS_SHRPHR>, <Peak_SHRPHR>, <RMS_Overall>, <Peak_Overall>, <RMS_SHRPHR_Enb>, <Pk_SHRPHR_Enb>, <RMSOverall_Enb>, <PkOverall_Enb>]\n\nParameters\n<1_RMS_EVM_PS>   - RMS offset EVM for PSDU portion\nRange: 0 - 100 %\nDefault value: 35 %\n\n<2_Peak_EVM_PS>   - Peak offset EVM for PSDU portion\nRange: 0 - 100 %\nDefault value: 35 %\n\n<3_RMS_PS_Enb>   - Disables | enables the limit check for RMS offset EVM within PSDU portion.\nOFF | ON\nDeafult value: ON\n\n<4_Peak_PS_Enb>   - Disables | enables the limit check for peak offset EVM within PSDU portion.\nOFF | ON\nDefault value: OFF\n\n<5_RMS_EVM_SP>   - RMS offset EVM for SHR + PHR portion\nRange: 0 % to 100 %\nDeaful value: 35 %\n\n<6_Peak_EVM_SP>   - Peak offset EVM for SHR + PHR portion\nRange: 0 % to 100 %\nDeaful value: 35 %\n\n<7_RMS_EVM_All>   - Overall RMS offset EVM for complete PPDU\nRange: 0 % to 100 %\nDeaful value: 35 %\n\n <8_Peak_EVM_All>   - Overall Peak offset EVM for complete PPDU\nRange: 0 % to 100 %\nDeaful value: 35 %\n\n<9_RMS_SP_Enb>   - Disables | enables the RMS limit check for offset EVM within SHR + PHR portion.\nOFF | ON\nDefault value: ON\n\n<10_Peak_SP_Enb>   - Disables | enables the peak limit check for offset EVM within SHR + PHR portion.\nOFF | ON\nDefault value: OFF\n\n<11_RMS_Sll_Enb>    - Disables | enables the RMS limit check for overall offset EVM for complete PPDU.\nOFF | ON\nDefault value: ON\n\n<12_Peak_All_Enb>   - Disables | enables the peak limit check for overall offset EVM for complete PPDU.\nOFF | ON\nDefault value: OFF\n\nAvailable Repeated Capabilities:\ninstance: i0, i1, i2, i3, i4, i5, i6, i7, i8, i9, i10, i11, i12, i13, i14, i15, i16, i17, i18, i19, i20, i21, i22, i23, i24, i25, i26, i27, i28, i29, i30, i31, i32\r\n\nRemote-control command(s):\nCONFigure:WPAN:MEAS<i>:MEValuation:LIMit:EVM[:OFFSet]"}, {"Level"=3, "Class Only"=FALSE, "Identifier"="RSCMPLRWM_ATTR_HIDDEN_MULTIEVAL_LO_LEAKAGE_LIMIT", "Descriptive Name"="MultiEval LO Leakage Limit", "Data Type"=6, "Command"="CONF:WPAN:MEAS{instance}:MEV:LIM:LLE", "Access"=2, "Range Table"="", "Read Callback"="", "Write Callback"="", "Supported Models"="", "Instrument Options"="", "Flags"=8, "Help"="Defines upper limit for the LO leakage value.\n\nSyntax:\nCONFigure:WPAN:MEAS<i>:MEValuation:LIMit:LLEakage <LO_Leakage>, <LO_Leakage_Enb>\n\nParameters:\n<LO_Leakage>\nRange: -90 - 0\nDefault value: -40\n\n<LO_Leakage_Enb>   - Disables | enables the limit check for LO leakage.\nOFF | ON\nDefault value: ON\n\nAvailable Repeated Capabilities:\ninstance: i0, i1, i2, i3, i4, i5, i6, i7, i8, i9, i10, i11, i12, i13, i14, i15, i16, i17, i18, i19, i20, i21, i22, i23, i24, i25, i26, i27, i28, i29, i30, i31, i32\r\n\nRemote-control command(s):\nCONFigure:WPAN:MEAS<i>:MEValuation:LIMit:LLEakage"}, {"Level"=3, "Class Only"=FALSE, "Identifier"="RSCMPLRWM_ATTR_HIDDEN_MULTIEVAL_FREQUENCY_ACCURACY_LIMIT", "Descriptive Name"="MultiEval Frequency Accuracy Limit", "Data Type"=6, "Command"="CONF:WPAN:MEAS{instance}:MEV:LIM:FACC", "Access"=2, "Range Table"="", "Read Callback"="", "Write Callback"="", "Supported Models"="", "Instrument Options"="", "Flags"=8, "Help"="Defines the upper limit for the frequency accuracy.\n\nSyntax:\nCONFigure:WPAN:MEAS<i>:MEValuation:LIMit:FACCuracy <FreqAccuracyppm>, <FreqAccuracykHz>, <FreqAccppmEnble>, <FreqAcckHzEnble>\n\nParameters:\n<FreqAccuracyppm>\nRange: 0 - 80\nDefault value: 40\n\n<FreqAccuracykHz>\nRange: 0 - 200\nDefault value: 98\n\n<FreqAccppmEnble>   - Disable or enable limit check for frequency accuracy defined in ppm.\nOFF | ON\nDefault value: ON\n\n<FreqAcckHzEnble>   - Disable or enable limit check for frequency accuracy defined in kHz.\nOFF | ON\nDefault value: ON\n\nAvailable Repeated Capabilities:\ninstance: i0, i1, i2, i3, i4, i5, i6, i7, i8, i9, i10, i11, i12, i13, i14, i15, i16, i17, i18, i19, i20, i21, i22, i23, i24, i25, i26, i27, i28, i29, i30, i31, i32\r\n\nRemote-control command(s):\nCONFigure:WPAN:MEAS<i>:MEValuation:LIMit:FACCuracy"}, {"Level"=3, "Class Only"=FALSE, "Identifier"="RSCMPLRWM_ATTR_HIDDEN_MULTIEVAL_POWER_VS_TIME_LIMIT", "Descriptive Name"="MultiEval Power Vs Time Limit", "Data Type"=6, "Command"="CONF:WPAN:MEAS{instance}:MEV:LIM:PVT", "Access"=2, "Range Table"="", "Read Callback"="", "Write Callback"="", "Supported Models"="", "Instrument Options"="", "Flags"=8, "Help"="Sets and enables or disables a lower limit for PVT measurements.\n\nSyntax:\nCONFigure:WPAN:MEAS<i>:MEValuation:LIMit:PVTime <AveragePower>, <AvgPowEnabled>\n\nParameters:\n<AveragePower>\nRange: -50 - 55\nDefault value: -3\n\n<AvgPowEnabled>\nOFF | ON\nDefault value:ON\n\nAvailable Repeated Capabilities:\ninstance: i0, i1, i2, i3, i4, i5, i6, i7, i8, i9, i10, i11, i12, i13, i14, i15, i16, i17, i18, i19, i20, i21, i22, i23, i24, i25, i26, i27, i28, i29, i30, i31, i32\r\n\nRemote-control command(s):\nCONFigure:WPAN:MEAS<i>:MEValuation:LIMit:PVTime"}, {"Level"=3, "Class Only"=FALSE, "Identifier"="RSCMPLRWM_ATTR_HIDDEN_MULTIEVAL_POWER_SPECTRUM_DENSITY_LIMIT", "Descriptive Name"="MultiEval Power Spectrum Density Limit", "Data Type"=6, "Command"="CONF:WPAN:MEAS{instance}:MEV:LIM:SPEC", "Access"=2, "Range Table"="", "Read Callback"="", "Write Callback"="", "Supported Models"="", "Instrument Options"="", "Flags"=8, "Help"="Defines upper limits of power spectrum density for the absolute power and for the power relative to the reference power.\n\nSyntax:\nCONFigure:WPAN:MEAS<i>:MEValuation:LIMit:SPECtrum <PSDAbsolute>, <PSDRelative>, <PSDEnabled>\n\nParameters:\n<PSDAbsolute>\nRange: -80 -  5\nDefault value: -30\n\n<PSDRelative>\nRange: -80 - 0\nDefault value: -20\n\n<PSDEnabled>   - Disable or enable limit check.\nOFF | ON\nDefault value: ON\n\nAvailable Repeated Capabilities:\ninstance: i0, i1, i2, i3, i4, i5, i6, i7, i8, i9, i10, i11, i12, i13, i14, i15, i16, i17, i18, i19, i20, i21, i22, i23, i24, i25, i26, i27, i28, i29, i30, i31, i32\r\n\nRemote-control command(s):\nCONFigure:WPAN:MEAS<i>:MEValuation:LIMit:SPECtrum"}, {"Level"=3, "Class Only"=FALSE, "Identifier"="RSCMPLRWM_ATTR_HIDDEN_MULTIEVAL_SYMBOL_RATE_ERROR_LIMIT", "Descriptive Name"="MultiEval Symbol Rate Error Limit", "Data Type"=6, "Command"="CONF:WPAN:MEAS{instance}:MEV:LIM:SRAT", "Access"=2, "Range Table"="", "Read Callback"="", "Write Callback"="", "Supported Models"="", "Instrument Options"="", "Flags"=8, "Help"="Defines upper limit for symbol rate error.\n\nSyntax:\nCONFigure:WPAN:MEAS<i>:MEValuation:LIMit:SRATe <SymbolRate>, <SymbolRateEnble>\n\nParameters:\n<SymbolRate>\nRange: 0 - 80\nDefault: 40\n\n<SymbolRateEnble>   - Disables | enables the limit check for symbol rate error.\nOFF | ON\nDefault: ON\n\nAvailable Repeated Capabilities:\ninstance: i0, i1, i2, i3, i4, i5, i6, i7, i8, i9, i10, i11, i12, i13, i14, i15, i16, i17, i18, i19, i20, i21, i22, i23, i24, i25, i26, i27, i28, i29, i30, i31, i32\r\n\nRemote-control command(s):\nCONFigure:WPAN:MEAS<i>:MEValuation:LIMit:SRATe"}, {"Level"=2, "Class Only"=TRUE, "Identifier"="", "Descriptive Name"="Results", "Data Type"=0, "Command"="", "Access"=0, "Range Table"="", "Read Callback"="", "Write Callback"="", "Supported Models"="", "Instrument Options"="", "Flags"=0, "Help"="The attributes in this class retrieve results for multi-evaluation measurements."}, {"Level"=3, "Class Only"=TRUE, "Identifier"="", "Descriptive Name"="Modulation", "Data Type"=0, "Command"="", "Access"=0, "Range Table"="", "Read Callback"="", "Write Callback"="", "Supported Models"="", "Instrument Options"="", "Flags"=0, "Help"="The following attributes return the modulation results."}, {"Level"=4, "Class Only"=FALSE, "Identifier"="RSCMPLRWM_ATTR_HIDDEN_QUERY_MULTIEVAL_MODULATION_CURRENT_LIMIT_CHECK_RESULTS", "Descriptive Name"="Query MultiEval Modulation Current Limit Check Results", "Data Type"=6, "Command"="CALC:WPAN:MEAS{instance}:MEV:MOD:CURR?", "Access"=0, "Range Table"="", "Read Callback"="", "Write Callback"="", "Supported Models"="", "Instrument Options"="", "Flags"=8, "Help"="Returns the current limit check single value results.\n\nReturn values:\n<1_Reliability>   - Reliability indicator\nfloat\n\n<2_OutOfTol>   -  Out of tolerance result\nfloat\nRange: 0 - 100\n\n<3_AveragePower>   - Average burst power\nfloat\nRange: -99.99 - 99.99\n\n<4_SymbolRateErr>   - Symbol rate error\nfloat\nRange: -1000 - 1000\n\n<5_FreqTolerance>   -  Frequency accuracy\nfloat\nRange: -1000 - 1000\n\n<6_FreqAccuracy>   -  Frequency accuracy\nfloat\nRange: -0.99999E+6 - 0.99999E+6\n\n<7_RMS_EVM_PS>   -  Offset error vector magnitude within PSDU portion, RMS value\nfloat\nRange: 0 -100\n\n<8_Peak_EVM_PS>   -  Offset error vector magnitude within PSDU portion,  peak value\nfloat\nRange: 0 - 100\n\n<9_RMS_EVM_SP>   -  Offset error vector magnitude within SHR + PHR portion, RMS value\nfloat\nRange: 0 - 999.99\n\n<10_Peak_EVM_SP>   -  Offset error vector magnitude within SHR + PHR portion, peak value\nfloat\nRange: 0 - 999.99\n\n<11_RMS_EVM_All>   -  Overall offset error vector magnitude for complete PPDU, RMS value\nfloat\nRange: 0 - 999.99\n\n<12_Peak_EVM_All>   -  Overall offset error vector magnitude for complete PPDU, peak value\nfloat\nRange: 0 - 999.99\n\n<13_LoLeakage>   -  Local oscillator leakage\nfloat\nRange: -99.99 - 99.99\n\nAvailable Repeated Capabilities:\ninstance: i0, i1, i2, i3, i4, i5, i6, i7, i8, i9, i10, i11, i12, i13, i14, i15, i16, i17, i18, i19, i20, i21, i22, i23, i24, i25, i26, i27, i28, i29, i30, i31, i32\r\n\nRemote-control command(s):\nCALCulate:WPAN:MEAS<i>:MEValuation:MODulation[:OFFSet]:CURRent?"}, {"Level"=4, "Class Only"=FALSE, "Identifier"="RSCMPLRWM_ATTR_HIDDEN_QUERY_MULTIEVAL_MODULATION_AVERAGE_LIMIT_CHECK_RESULTS", "Descriptive Name"="Query MultiEval Modulation Average Limit Check Results", "Data Type"=6, "Command"="CALC:WPAN:MEAS{instance}:MEV:MOD:AVER?", "Access"=0, "Range Table"="", "Read Callback"="", "Write Callback"="", "Supported Models"="", "Instrument Options"="", "Flags"=8, "Help"="Returns the average limit check single value results.\n\nReturn values:\n<1_Reliability>   - Reliability indicator\nfloat\n\n<2_OutOfTol>   -  Out of tolerance result\nfloat\nRange: 0 - 100\n\n<3_AveragePower>   - Average burst power\nfloat\nRange: -99.99 - 99.99\n\n<4_SymbolRateErr>   - Symbol rate error\nfloat\nRange: -1000 - 1000\n\n<5_FreqTolerance>   -  Frequency accuracy\nfloat\nRange: -1000 - 1000\n\n<6_FreqAccuracy>   -  Frequency accuracy\nfloat\nRange: -0.99999E+6 - 0.99999E+6\n\n<7_RMS_EVM_PS>   -  Offset error vector magnitude within PSDU portion, RMS value\nfloat\nRange: 0 -100\n\n<8_Peak_EVM_PS>   -  Offset error vector magnitude within PSDU portion,  peak value\nfloat\nRange: 0 - 100\n\n<9_RMS_EVM_SP>   -  Offset error vector magnitude within SHR + PHR portion, RMS value\nfloat\nRange: 0 - 999.99\n\n<10_Peak_EVM_SP>   -  Offset error vector magnitude within SHR + PHR portion, peak value\nfloat\nRange: 0 - 999.99\n\n<11_RMS_EVM_All>   -  Overall offset error vector magnitude for complete PPDU, RMS value\nfloat\nRange: 0 - 999.99\n\n<12_Peak_EVM_All>   -  Overall offset error vector magnitude for complete PPDU, peak value\nfloat\nRange: 0 - 999.99\n\n<13_LoLeakage>   -  Local oscillator leakage\nfloat\nRange: -99.99 - 99.99\n\nAvailable Repeated Capabilities:\ninstance: i0, i1, i2, i3, i4, i5, i6, i7, i8, i9, i10, i11, i12, i13, i14, i15, i16, i17, i18, i19, i20, i21, i22, i23, i24, i25, i26, i27, i28, i29, i30, i31, i32\r\n\nRemote-control command(s):\nCALCulate:WPAN:MEAS<i>:MEValuation:MODulation[:OFFSet]:AVERage?"}, {"Level"=4, "Class Only"=FALSE, "Identifier"="RSCMPLRWM_ATTR_HIDDEN_QUERY_MULTIEVAL_MODULATION_MAXIMUM_LIMIT_CHECK_RESULTS", "Descriptive Name"="Query MultiEval Modulation Maximum Limit Check Results", "Data Type"=6, "Command"="CALC:WPAN:MEAS{instance}:MEV:MOD:MAX?", "Access"=0, "Range Table"="", "Read Callback"="", "Write Callback"="", "Supported Models"="", "Instrument Options"="", "Flags"=8, "Help"="Returns the maximum limit check single value results.\n\nReturn values:\n<1_Reliability>   - Reliability indicator\nfloat\n\n<2_OutOfTol>   -  Out of tolerance result\nfloat\nRange: 0 - 100\n\n<3_AveragePower>   - Average burst power\nfloat\nRange: -99.99 - 99.99\n\n<4_SymbolRateErr>   - Symbol rate error\nfloat\nRange: -1000 - 1000\n\n<5_FreqTolerance>   -  Frequency accuracy\nfloat\nRange: -1000 - 1000\n\n<6_FreqAccuracy>   -  Frequency accuracy\nfloat\nRange: -0.99999E+6 - 0.99999E+6\n\n<7_RMS_EVM_PS>   -  Offset error vector magnitude within PSDU portion, RMS value\nfloat\nRange: 0 -100\n\n<8_Peak_EVM_PS>   -  Offset error vector magnitude within PSDU portion,  peak value\nfloat\nRange: 0 - 100\n\n<9_RMS_EVM_SP>   -  Offset error vector magnitude within SHR + PHR portion, RMS value\nfloat\nRange: 0 - 999.99\n\n<10_Peak_EVM_SP>   -  Offset error vector magnitude within SHR + PHR portion, peak value\nfloat\nRange: 0 - 999.99\n\n<11_RMS_EVM_All>   -  Overall offset error vector magnitude for complete PPDU, RMS value\nfloat\nRange: 0 - 999.99\n\n<12_Peak_EVM_All>   -  Overall offset error vector magnitude for complete PPDU, peak value\nfloat\nRange: 0 - 999.99\n\n<13_LoLeakage>   -  Local oscillator leakage\nfloat\nRange: -99.99 - 99.99\n\nAvailable Repeated Capabilities:\ninstance: i0, i1, i2, i3, i4, i5, i6, i7, i8, i9, i10, i11, i12, i13, i14, i15, i16, i17, i18, i19, i20, i21, i22, i23, i24, i25, i26, i27, i28, i29, i30, i31, i32\r\n\nRemote-control command(s):\nCALCulate:WPAN:MEAS<i>:MEValuation:MODulation[:OFFSet]:MAXimum?"}, {"Level"=4, "Class Only"=FALSE, "Identifier"="RSCMPLRWM_ATTR_HIDDEN_QUERY_MULTIEVAL_MODULATION_STANDARD_DEVIATION_LIMIT_CHECK_RESULTS", "Descriptive Name"="Query MultiEval Modulation Standard Deviation Limit Check Results", "Data Type"=6, "Command"="CALC:WPAN:MEAS{instance}:MEV:MOD:SDEV?", "Access"=0, "Range Table"="", "Read Callback"="", "Write Callback"="", "Supported Models"="", "Instrument Options"="", "Flags"=8, "Help"="Returns the standard deviation limit check single value results.\n\nReturn values:\n<1_Reliability>   - Reliability indicator\nfloat\n\n<2_OutOfTol>   -  Out of tolerance result\nfloat\nRange: 0 - 100\n\n<3_AveragePower>   - Average burst power\nfloat\nRange: -99.99 - 99.99\n\n<4_SymbolRateErr>   - Symbol rate error\nfloat\nRange: -1000 - 1000\n\n<5_FreqTolerance>   -  Frequency accuracy\nfloat\nRange: -1000 - 1000\n\n<6_FreqAccuracy>   -  Frequency accuracy\nfloat\nRange: -0.99999E+6 - 0.99999E+6\n\n<7_RMS_EVM_PS>   -  Offset error vector magnitude within PSDU portion, RMS value\nfloat\nRange: 0 -100\n\n<8_Peak_EVM_PS>   -  Offset error vector magnitude within PSDU portion,  peak value\nfloat\nRange: 0 - 100\n\n<9_RMS_EVM_SP>   -  Offset error vector magnitude within SHR + PHR portion, RMS value\nfloat\nRange: 0 - 999.99\n\n<10_Peak_EVM_SP>   -  Offset error vector magnitude within SHR + PHR portion, peak value\nfloat\nRange: 0 - 999.99\n\n<11_RMS_EVM_All>   -  Overall offset error vector magnitude for complete PPDU, RMS value\nfloat\nRange: 0 - 999.99\n\n<12_Peak_EVM_All>   -  Overall offset error vector magnitude for complete PPDU, peak value\nfloat\nRange: 0 - 999.99\n\n<13_LoLeakage>   -  Local oscillator leakage\nfloat\nRange: -99.99 - 99.99\n\nAvailable Repeated Capabilities:\ninstance: i0, i1, i2, i3, i4, i5, i6, i7, i8, i9, i10, i11, i12, i13, i14, i15, i16, i17, i18, i19, i20, i21, i22, i23, i24, i25, i26, i27, i28, i29, i30, i31, i32\r\n\nRemote-control command(s):\nCALCulate:WPAN:MEAS<i>:MEValuation:MODulation[:OFFSet]:SDEViation?"}, {"Level"=4, "Class Only"=FALSE, "Identifier"="RSCMPLRWM_ATTR_HIDDEN_FETCH_MULTIEVAL_MODULATION_CURRENT_RESULTS", "Descriptive Name"="Fetch MultiEval Modulation Current Results", "Data Type"=6, "Command"="FETC:WPAN:MEAS{instance}:MEV:MOD:CURR?", "Access"=0, "Range Table"="", "Read Callback"="", "Write Callback"="", "Supported Models"="", "Instrument Options"="", "Flags"=8, "Help"="Returns the current single value results.\n\nReturn values:\n<1_Reliability>   - Reliability indicator\nfloat\n\n<2_OutOfTol>   -  Out of tolerance result\nfloat\nRange: 0 - 100\n\n<3_AveragePower>   - Average burst power\nfloat\nRange: -99.99 - 99.99\n\n<4_SymbolRateErr>   - Symbol rate error\nfloat\nRange: -1000 - 1000\n\n<5_FreqTolerance>   -  Frequency accuracy\nfloat\nRange: -1000 - 1000\n\n<6_FreqAccuracy>   -  Frequency accuracy\nfloat\nRange: -0.99999E+6 - 0.99999E+6\n\n<7_RMS_EVM_PS>   -  Offset error vector magnitude within PSDU portion, RMS value\nfloat\nRange: 0 -100\n\n<8_Peak_EVM_PS>   -  Offset error vector magnitude within PSDU portion,  peak value\nfloat\nRange: 0 - 100\n\n<9_RMS_EVM_SP>   -  Offset error vector magnitude within SHR + PHR portion, RMS value\nfloat\nRange: 0 - 999.99\n\n<10_Peak_EVM_SP>   -  Offset error vector magnitude within SHR + PHR portion, peak value\nfloat\nRange: 0 - 999.99\n\n<11_RMS_EVM_All>   -  Overall offset error vector magnitude for complete PPDU, RMS value\nfloat\nRange: 0 - 999.99\n\n<12_Peak_EVM_All>   -  Overall offset error vector magnitude for complete PPDU, peak value\nfloat\nRange: 0 - 999.99\n\n<13_LoLeakage>   -  Local oscillator leakage\nfloat\nRange: -99.99 - 99.99\n\nAvailable Repeated Capabilities:\ninstance: i0, i1, i2, i3, i4, i5, i6, i7, i8, i9, i10, i11, i12, i13, i14, i15, i16, i17, i18, i19, i20, i21, i22, i23, i24, i25, i26, i27, i28, i29, i30, i31, i32\r\n\nRemote-control command(s):\nFETCh:WPAN:MEAS<i>:MEValuation:MODulation[:OFFSet]:CURRent?"}, {"Level"=4, "Class Only"=FALSE, "Identifier"="RSCMPLRWM_ATTR_HIDDEN_FETCH_MULTIEVAL_MODULATION_AVERAGE_RESULTS", "Descriptive Name"="Fetch MultiEval Modulation Average Results", "Data Type"=6, "Command"="FETC:WPAN:MEAS{instance}:MEV:MOD:AVER?", "Access"=0, "Range Table"="", "Read Callback"="", "Write Callback"="", "Supported Models"="", "Instrument Options"="", "Flags"=8, "Help"="Returns the average single value results.\n\nReturn values:\n<1_Reliability>   - Reliability indicator\nfloat\n\n<2_OutOfTol>   -  Out of tolerance result\nfloat\nRange: 0 - 100\n\n<3_AveragePower>   - Average burst power\nfloat\nRange: -99.99 - 99.99\n\n<4_SymbolRateErr>   - Symbol rate error\nfloat\nRange: -1000 - 1000\n\n<5_FreqTolerance>   -  Frequency accuracy\nfloat\nRange: -1000 - 1000\n\n<6_FreqAccuracy>   -  Frequency accuracy\nfloat\nRange: -0.99999E+6 - 0.99999E+6\n\n<7_RMS_EVM_PS>   -  Offset error vector magnitude within PSDU portion, RMS value\nfloat\nRange: 0 -100\n\n<8_Peak_EVM_PS>   -  Offset error vector magnitude within PSDU portion,  peak value\nfloat\nRange: 0 - 100\n\n<9_RMS_EVM_SP>   -  Offset error vector magnitude within SHR + PHR portion, RMS value\nfloat\nRange: 0 - 999.99\n\n<10_Peak_EVM_SP>   -  Offset error vector magnitude within SHR + PHR portion, peak value\nfloat\nRange: 0 - 999.99\n\n<11_RMS_EVM_All>   -  Overall offset error vector magnitude for complete PPDU, RMS value\nfloat\nRange: 0 - 999.99\n\n<12_Peak_EVM_All>   -  Overall offset error vector magnitude for complete PPDU, peak value\nfloat\nRange: 0 - 999.99\n\n<13_LoLeakage>   -  Local oscillator leakage\nfloat\nRange: -99.99 - 99.99\n\nAvailable Repeated Capabilities:\ninstance: i0, i1, i2, i3, i4, i5, i6, i7, i8, i9, i10, i11, i12, i13, i14, i15, i16, i17, i18, i19, i20, i21, i22, i23, i24, i25, i26, i27, i28, i29, i30, i31, i32\r\n\nRemote-control command(s):\nFETCh:WPAN:MEAS<i>:MEValuation:MODulation[:OFFSet]:AVERage?"}, {"Level"=4, "Class Only"=FALSE, "Identifier"="RSCMPLRWM_ATTR_HIDDEN_FETCH_MULTIEVAL_MODULATION_MAXIMUM_RESULTS", "Descriptive Name"="Fetch MultiEval Modulation Maximum Results", "Data Type"=6, "Command"="FETC:WPAN:MEAS{instance}:MEV:MOD:MAX?", "Access"=0, "Range Table"="", "Read Callback"="", "Write Callback"="", "Supported Models"="", "Instrument Options"="", "Flags"=8, "Help"="Returns the maximum single value results.\n\nReturn values:\n<1_Reliability>   - Reliability indicator\nfloat\n\n<2_OutOfTol>   -  Out of tolerance result\nfloat\nRange: 0 - 100\n\n<3_AveragePower>   - Average burst power\nfloat\nRange: -99.99 - 99.99\n\n<4_SymbolRateErr>   - Symbol rate error\nfloat\nRange: -1000 - 1000\n\n<5_FreqTolerance>   -  Frequency accuracy\nfloat\nRange: -1000 - 1000\n\n<6_FreqAccuracy>   -  Frequency accuracy\nfloat\nRange: -0.99999E+6 - 0.99999E+6\n\n<7_RMS_EVM_PS>   -  Offset error vector magnitude within PSDU portion, RMS value\nfloat\nRange: 0 -100\n\n<8_Peak_EVM_PS>   -  Offset error vector magnitude within PSDU portion,  peak value\nfloat\nRange: 0 - 100\n\n<9_RMS_EVM_SP>   -  Offset error vector magnitude within SHR + PHR portion, RMS value\nfloat\nRange: 0 - 999.99\n\n<10_Peak_EVM_SP>   -  Offset error vector magnitude within SHR + PHR portion, peak value\nfloat\nRange: 0 - 999.99\n\n<11_RMS_EVM_All>   -  Overall offset error vector magnitude for complete PPDU, RMS value\nfloat\nRange: 0 - 999.99\n\n<12_Peak_EVM_All>   -  Overall offset error vector magnitude for complete PPDU, peak value\nfloat\nRange: 0 - 999.99\n\n<13_LoLeakage>   -  Local oscillator leakage\nfloat\nRange: -99.99 - 99.99\n\nAvailable Repeated Capabilities:\ninstance: i0, i1, i2, i3, i4, i5, i6, i7, i8, i9, i10, i11, i12, i13, i14, i15, i16, i17, i18, i19, i20, i21, i22, i23, i24, i25, i26, i27, i28, i29, i30, i31, i32\r\n\nRemote-control command(s):\nFETCh:WPAN:MEAS<i>:MEValuation:MODulation[:OFFSet]:MAXimum?"}, {"Level"=4, "Class Only"=FALSE, "Identifier"="RSCMPLRWM_ATTR_HIDDEN_FETCH_MULTIEVAL_MODULATION_STANDARD_DEVIATION_RESULTS", "Descriptive Name"="Fetch MultiEval Modulation Standard Deviation Results", "Data Type"=6, "Command"="FETC:WPAN:MEAS{instance}:MEV:MOD:SDEV?", "Access"=0, "Range Table"="", "Read Callback"="", "Write Callback"="", "Supported Models"="", "Instrument Options"="", "Flags"=8, "Help"="Returns the standard deviation single value results.\n\nReturn values:\n<1_Reliability>   - Reliability indicator\nfloat\n\n<2_OutOfTol>   -  Out of tolerance result\nfloat\nRange: 0 - 100\n\n<3_AveragePower>   - Average burst power\nfloat\nRange: -99.99 - 99.99\n\n<4_SymbolRateErr>   - Symbol rate error\nfloat\nRange: -1000 - 1000\n\n<5_FreqTolerance>   -  Frequency accuracy\nfloat\nRange: -1000 - 1000\n\n<6_FreqAccuracy>   -  Frequency accuracy\nfloat\nRange: -0.99999E+6 - 0.99999E+6\n\n<7_RMS_EVM_PS>   -  Offset error vector magnitude within PSDU portion, RMS value\nfloat\nRange: 0 -100\n\n<8_Peak_EVM_PS>   -  Offset error vector magnitude within PSDU portion,  peak value\nfloat\nRange: 0 - 100\n\n<9_RMS_EVM_SP>   -  Offset error vector magnitude within SHR + PHR portion, RMS value\nfloat\nRange: 0 - 999.99\n\n<10_Peak_EVM_SP>   -  Offset error vector magnitude within SHR + PHR portion, peak value\nfloat\nRange: 0 - 999.99\n\n<11_RMS_EVM_All>   -  Overall offset error vector magnitude for complete PPDU, RMS value\nfloat\nRange: 0 - 999.99\n\n<12_Peak_EVM_All>   -  Overall offset error vector magnitude for complete PPDU, peak value\nfloat\nRange: 0 - 999.99\n\n<13_LoLeakage>   -  Local oscillator leakage\nfloat\nRange: -99.99 - 99.99\n\nAvailable Repeated Capabilities:\ninstance: i0, i1, i2, i3, i4, i5, i6, i7, i8, i9, i10, i11, i12, i13, i14, i15, i16, i17, i18, i19, i20, i21, i22, i23, i24, i25, i26, i27, i28, i29, i30, i31, i32\r\n\nRemote-control command(s):\nFETCh:WPAN:MEAS<i>:MEValuation:MODulation[:OFFSet]:SDEViation?"}, {"Level"=4, "Class Only"=FALSE, "Identifier"="RSCMPLRWM_ATTR_HIDDEN_READ_MULTIEVAL_MODULATION_CURRENT_RESULTS", "Descriptive Name"="Read MultiEval Modulation Current Results", "Data Type"=6, "Command"="READ:WPAN:MEAS{instance}:MEV:MOD:CURR?", "Access"=0, "Range Table"="", "Read Callback"="", "Write Callback"="", "Supported Models"="", "Instrument Options"="", "Flags"=8, "Help"="Starts a new single shot measurement and returns the current single value results.\n\nReturn values:\n<1_Reliability>   - Reliability indicator\nfloat\n\n<2_OutOfTol>   -  Out of tolerance result\nfloat\nRange: 0 - 100\n\n<3_AveragePower>   - Average burst power\nfloat\nRange: -99.99 - 99.99\n\n<4_SymbolRateErr>   - Symbol rate error\nfloat\nRange: -1000 - 1000\n\n<5_FreqTolerance>   -  Frequency accuracy\nfloat\nRange: -1000 - 1000\n\n<6_FreqAccuracy>   -  Frequency accuracy\nfloat\nRange: -0.99999E+6 - 0.99999E+6\n\n<7_RMS_EVM_PS>   -  Offset error vector magnitude within PSDU portion, RMS value\nfloat\nRange: 0 -100\n\n<8_Peak_EVM_PS>   -  Offset error vector magnitude within PSDU portion,  peak value\nfloat\nRange: 0 - 100\n\n<9_RMS_EVM_SP>   -  Offset error vector magnitude within SHR + PHR portion, RMS value\nfloat\nRange: 0 - 999.99\n\n<10_Peak_EVM_SP>   -  Offset error vector magnitude within SHR + PHR portion, peak value\nfloat\nRange: 0 - 999.99\n\n<11_RMS_EVM_All>   -  Overall offset error vector magnitude for complete PPDU, RMS value\nfloat\nRange: 0 - 999.99\n\n<12_Peak_EVM_All>   -  Overall offset error vector magnitude for complete PPDU, peak value\nfloat\nRange: 0 - 999.99\n\n<13_LoLeakage>   -  Local oscillator leakage\nfloat\nRange: -99.99 - 99.99\n\nAvailable Repeated Capabilities:\ninstance: i0, i1, i2, i3, i4, i5, i6, i7, i8, i9, i10, i11, i12, i13, i14, i15, i16, i17, i18, i19, i20, i21, i22, i23, i24, i25, i26, i27, i28, i29, i30, i31, i32\r\n\nRemote-control command(s):\nREAD:WPAN:MEAS<i>:MEValuation:MODulation[:OFFSet]:CURRent?"}, {"Level"=4, "Class Only"=FALSE, "Identifier"="RSCMPLRWM_ATTR_HIDDEN_READ_MULTIEVAL_MODULATION_AVERAGE_RESULTS", "Descriptive Name"="Read MultiEval Modulation Average Results", "Data Type"=6, "Command"="READ:WPAN:MEAS{instance}:MEV:MOD:AVER?", "Access"=0, "Range Table"="", "Read Callback"="", "Write Callback"="", "Supported Models"="", "Instrument Options"="", "Flags"=8, "Help"="Starts a new single shot measurement and returns the average single value results.\n\nReturn values:\n<1_Reliability>   - Reliability indicator\nfloat\n\n<2_OutOfTol>   -  Out of tolerance result\nfloat\nRange: 0 - 100\n\n<3_AveragePower>   - Average burst power\nfloat\nRange: -99.99 - 99.99\n\n<4_SymbolRateErr>   - Symbol rate error\nfloat\nRange: -1000 - 1000\n\n<5_FreqTolerance>   - Frequency accuracy\nfloat\nRange: -1000 - 1000\n\n<6_FreqAccuracy>   -  Frequency accuracy\nfloat\nRange: -0.99999E+6 - 0.99999E+6\n\n<7_RMS_EVM_PS>   -  Offset error vector magnitude within PSDU portion, RMS value\nfloat\nRange: 0 -100\n\n<8_Peak_EVM_PS>   -  Offset error vector magnitude within PSDU portion,  peak value\nfloat\nRange: 0 - 100\n\n<9_RMS_EVM_SP>   -  Offset error vector magnitude within SHR + PHR portion, RMS value\nfloat\nRange: 0 - 999.99\n\n<10_Peak_EVM_SP>   -  Offset error vector magnitude within SHR + PHR portion, peak value\nfloat\nRange: 0 - 999.99\n\n<11_RMS_EVM_All>   -  Overall offset error vector magnitude for complete PPDU, RMS value\nfloat\nRange: 0 - 999.99\n\n<12_Peak_EVM_All>   -  Overall offset error vector magnitude for complete PPDU, peak value\nfloat\nRange: 0 - 999.99\n\n<13_LoLeakage>   -  Local oscillator leakage\nfloat\nRange: -99.99 - 99.99\n\nAvailable Repeated Capabilities:\ninstance: i0, i1, i2, i3, i4, i5, i6, i7, i8, i9, i10, i11, i12, i13, i14, i15, i16, i17, i18, i19, i20, i21, i22, i23, i24, i25, i26, i27, i28, i29, i30, i31, i32\r\n\nRemote-control command(s):\nREAD:WPAN:MEAS<i>:MEValuation:MODulation[:OFFSet]:AVERage?"}, {"Level"=4, "Class Only"=FALSE, "Identifier"="RSCMPLRWM_ATTR_HIDDEN_READ_MULTIEVAL_MODULATION_MAXIMUM_RESULTS", "Descriptive Name"="Read MultiEval Modulation Maximum Results", "Data Type"=6, "Command"="READ:WPAN:MEAS{instance}:MEV:MOD:MAX?", "Access"=0, "Range Table"="", "Read Callback"="", "Write Callback"="", "Supported Models"="", "Instrument Options"="", "Flags"=8, "Help"="Starts a new single shot measurement and returns the maximum single value results.\n\nReturn values:\n<1_Reliability>   - Reliability indicator\nfloat\n\n<2_OutOfTol>   -  Out of tolerance result\nfloat\nRange: 0 - 100\n\n<3_AveragePower>   - Average burst power\nfloat\nRange: -99.99 - 99.99\n\n<4_SymbolRateErr>   - Symbol rate error\nfloat\nRange: -1000 - 1000\n\n<5_FreqTolerance>   -  Frequency accuracy\nfloat\nRange: -1000 - 1000\n\n<6_FreqAccuracy>   -  Frequency accuracy\nfloat\nRange: -0.99999E+6 - 0.99999E+6\n\n<7_RMS_EVM_PS>   -  Offset error vector magnitude within PSDU portion, RMS value\nfloat\nRange: 0 -100\n\n<8_Peak_EVM_PS>   -  Offset error vector magnitude within PSDU portion,  peak value\nfloat\nRange: 0 - 100\n\n<9_RMS_EVM_SP>   -  Offset error vector magnitude within SHR + PHR portion, RMS value\nfloat\nRange: 0 - 999.99\n\n<10_Peak_EVM_SP>   -  Offset error vector magnitude within SHR + PHR portion, peak value\nfloat\nRange: 0 - 999.99\n\n<11_RMS_EVM_All>   -  Overall offset error vector magnitude for complete PPDU, RMS value\nfloat\nRange: 0 - 999.99\n\n<12_Peak_EVM_All>   -  Overall offset error vector magnitude for complete PPDU, peak value\nfloat\nRange: 0 - 999.99\n\n<13_LoLeakage>   -  Local oscillator leakage\nfloat\nRange: -99.99 - 99.99\n\nAvailable Repeated Capabilities:\ninstance: i0, i1, i2, i3, i4, i5, i6, i7, i8, i9, i10, i11, i12, i13, i14, i15, i16, i17, i18, i19, i20, i21, i22, i23, i24, i25, i26, i27, i28, i29, i30, i31, i32\r\n\nRemote-control command(s):\nREAD:WPAN:MEAS<i>:MEValuation:MODulation[:OFFSet]:MAXimum?"}, {"Level"=4, "Class Only"=FALSE, "Identifier"="RSCMPLRWM_ATTR_HIDDEN_READ_MULTIEVAL_MODULATION_STANDARD_DEVIATION_RESULTS", "Descriptive Name"="Read MultiEval Modulation Standard Deviation Results", "Data Type"=6, "Command"="READ:WPAN:MEAS{instance}:MEV:MOD:SDEV?", "Access"=0, "Range Table"="", "Read Callback"="", "Write Callback"="", "Supported Models"="", "Instrument Options"="", "Flags"=8, "Help"="Starts a new single shot measurement and returns the standard deviation single value results.\n\nReturn values:\n<1_Reliability>   - Reliability indicator\nfloat\n\n<2_OutOfTol>   -  Out of tolerance result\nfloat\nRange: 0 - 100\n\n<3_AveragePower>   - Average burst power\nfloat\nRange: -99.99 - 99.99\n\n<4_SymbolRateErr>   - Symbol rate error\nfloat\nRange: -1000 - 1000\n\n<5_FreqTolerance>   -  Frequency accuracy\nfloat\nRange: -1000 - 1000\n\n<6_FreqAccuracy>   -  Frequency accuracy\nfloat\nRange: -0.99999E+6 - 0.99999E+6\n\n<7_RMS_EVM_PS>   -  Offset error vector magnitude within PSDU portion, RMS value\nfloat\nRange: 0 -100\n\n<8_Peak_EVM_PS>   -  Offset error vector magnitude within PSDU portion,  peak value\nfloat\nRange: 0 - 100\n\n<9_RMS_EVM_SP>   -  Offset error vector magnitude within SHR + PHR portion, RMS value\nfloat\nRange: 0 - 999.99\n\n<10_Peak_EVM_SP>   -  Offset error vector magnitude within SHR + PHR portion, peak value\nfloat\nRange: 0 - 999.99\n\n<11_RMS_EVM_All>   -  Overall offset error vector magnitude for complete PPDU, RMS value\nfloat\nRange: 0 - 999.99\n\n<12_Peak_EVM_All>   -  Overall offset error vector magnitude for complete PPDU, peak value\nfloat\nRange: 0 - 999.99\n\n<13_LoLeakage>   -  Local oscillator leakage\nfloat\nRange: -99.99 - 99.99\n\nAvailable Repeated Capabilities:\ninstance: i0, i1, i2, i3, i4, i5, i6, i7, i8, i9, i10, i11, i12, i13, i14, i15, i16, i17, i18, i19, i20, i21, i22, i23, i24, i25, i26, i27, i28, i29, i30, i31, i32\r\n\nRemote-control command(s):\nREAD:WPAN:MEAS<i>:MEValuation:MODulation[:OFFSet]:SDEViation?"}, {"Level"=4, "Class Only"=FALSE, "Identifier"="RSCMPLRWM_ATTR_HIDDEN_QUERY_MULTIEVAL_MODULATION_ABSOLUTE_CURRENT_LIMIT_CHECK_RESULTS", "Descriptive Name"="Query MultiEval Modulation Absolute Current Limit Check Results", "Data Type"=6, "Command"="CALC:WPAN:MEAS{instance}:MEV:MOD:ABS:CURR?", "Access"=0, "Range Table"="", "Read Callback"="", "Write Callback"="", "Supported Models"="", "Instrument Options"="", "Flags"=8, "Help"="Returns the absolute current limit check single value results.\n\nReturn values:\n<1_Reliability>   - Reliability indicator\nfloat\n\n<2_OutOfTol>   -  Out of tolerance result\nfloat\nRange: 0 - 100\n\n<3_AveragePower>   - Average burst power\nfloat\nRange: -99.99 - 99.99\n\n<4_SymbolRateErr>   - Symbol rate error\nfloat\nRange: -1000 - 1000\n\n<5_FreqTolerance>   -  Frequency accuracy\nfloat\nRange: -1000 - 1000\n\n<6_FreqAccuracy>   -  Frequency accuracy\nfloat\nRange: -0.99999E+6 - 0.99999E+6\n\n<7_RMS_EVM_PS>   -  Offset error vector magnitude within PSDU portion, RMS value\nfloat\nRange: 0 -100\n\n<8_Peak_EVM_PS>   -  Offset error vector magnitude within PSDU portion,  peak value\nfloat\nRange: 0 - 100\n\n<9_RMS_EVM_SP>   -  Offset error vector magnitude within SHR + PHR portion, RMS value\nfloat\nRange: 0 - 999.99\n\n<10_Peak_EVM_SP>   -  Offset error vector magnitude within SHR + PHR portion, peak value\nfloat\nRange: 0 - 999.99\n\n<11_RMS_EVM_All>   -  Overall offset error vector magnitude for complete PPDU, RMS value\nfloat\nRange: 0 - 999.99\n\n<12_Peak_EVM_All>   -  Overall offset error vector magnitude for complete PPDU, peak value\nfloat\nRange: 0 - 999.99\n\n<13_LoLeakage>   -  Local oscillator leakage\nfloat\nRange: -99.99 - 99.99\n\nAvailable Repeated Capabilities:\ninstance: i0, i1, i2, i3, i4, i5, i6, i7, i8, i9, i10, i11, i12, i13, i14, i15, i16, i17, i18, i19, i20, i21, i22, i23, i24, i25, i26, i27, i28, i29, i30, i31, i32\r\n\nRemote-control command(s):\nCALCulate:WPAN:MEAS<i>:MEValuation:MODulation:ABSolute:CURRent?"}, {"Level"=4, "Class Only"=FALSE, "Identifier"="RSCMPLRWM_ATTR_HIDDEN_QUERY_MULTIEVAL_MODULATION_ABSOLUTE_AVERAGE_LIMIT_CHECK_RESULTS", "Descriptive Name"="Query MultiEval Modulation Absolute Average Limit Check Results", "Data Type"=6, "Command"="CALC:WPAN:MEAS{instance}:MEV:MOD:ABS:AVER?", "Access"=0, "Range Table"="", "Read Callback"="", "Write Callback"="", "Supported Models"="", "Instrument Options"="", "Flags"=8, "Help"="Returns the absolute average limit check single value results.\n\nReturn values:\n<1_Reliability>   - Reliability indicator\nfloat\n\n<2_OutOfTol>   -  Out of tolerance result\nfloat\nRange: 0 - 100\n\n<3_AveragePower>   - Average burst power\nfloat\nRange: -99.99 - 99.99\n\n<4_SymbolRateErr>   - Symbol rate error\nfloat\nRange: -1000 - 1000\n\n<5_FreqTolerance>   -  Frequency accuracy\nfloat\nRange: -1000 - 1000\n\n<6_FreqAccuracy>   -  Frequency accuracy\nfloat\nRange: -0.99999E+6 - 0.99999E+6\n\n<7_RMS_EVM_PS>   -  Offset error vector magnitude within PSDU portion, RMS value\nfloat\nRange: 0 -100\n\n<8_Peak_EVM_PS>   -  Offset error vector magnitude within PSDU portion,  peak value\nfloat\nRange: 0 - 100\n\n<9_RMS_EVM_SP>   -  Offset error vector magnitude within SHR + PHR portion, RMS value\nfloat\nRange: 0 - 999.99\n\n<10_Peak_EVM_SP>   -  Offset error vector magnitude within SHR + PHR portion, peak value\nfloat\nRange: 0 - 999.99\n\n<11_RMS_EVM_All>   -  Overall offset error vector magnitude for complete PPDU, RMS value\nfloat\nRange: 0 - 999.99\n\n<12_Peak_EVM_All>   -  Overall offset error vector magnitude for complete PPDU, peak value\nfloat\nRange: 0 - 999.99\n\n<13_LoLeakage>   -  Local oscillator leakage\nfloat\nRange: -99.99 - 99.99\n\nAvailable Repeated Capabilities:\ninstance: i0, i1, i2, i3, i4, i5, i6, i7, i8, i9, i10, i11, i12, i13, i14, i15, i16, i17, i18, i19, i20, i21, i22, i23, i24, i25, i26, i27, i28, i29, i30, i31, i32\r\n\nRemote-control command(s):\nCALCulate:WPAN:MEAS<i>:MEValuation:MODulation:ABSolute:AVERage?"}, {"Level"=4, "Class Only"=FALSE, "Identifier"="RSCMPLRWM_ATTR_HIDDEN_QUERY_MULTIEVAL_MODULATION_ABSOLUTE_MAXIMUM_LIMIT_CHECK_RESULTS", "Descriptive Name"="Query MultiEval Modulation Absolute Maximum Limit Check Results", "Data Type"=6, "Command"="CALC:WPAN:MEAS{instance}:MEV:MOD:ABS:MAX?", "Access"=0, "Range Table"="", "Read Callback"="", "Write Callback"="", "Supported Models"="", "Instrument Options"="", "Flags"=8, "Help"="Returns the absolute maximum limit check single value results.\n\nReturn values:\n<1_Reliability>   - Reliability indicator\nfloat\n\n<2_OutOfTol>   -  Out of tolerance result\nfloat\nRange: 0 - 100\n\n<3_AveragePower>   - Average burst power\nfloat\nRange: -99.99 - 99.99\n\n<4_SymbolRateErr>   - Symbol rate error\nfloat\nRange: -1000 - 1000\n\n<5_FreqTolerance>   -  Frequency accuracy\nfloat\nRange: -1000 - 1000\n\n<6_FreqAccuracy>   -  Frequency accuracy\nfloat\nRange: -0.99999E+6 - 0.99999E+6\n\n<7_RMS_EVM_PS>   -  Offset error vector magnitude within PSDU portion, RMS value\nfloat\nRange: 0 -100\n\n<8_Peak_EVM_PS>   -  Offset error vector magnitude within PSDU portion,  peak value\nfloat\nRange: 0 - 100\n\n<9_RMS_EVM_SP>   -  Offset error vector magnitude within SHR + PHR portion, RMS value\nfloat\nRange: 0 - 999.99\n\n<10_Peak_EVM_SP>   -  Offset error vector magnitude within SHR + PHR portion, peak value\nfloat\nRange: 0 - 999.99\n\n<11_RMS_EVM_All>   -  Overall offset error vector magnitude for complete PPDU, RMS value\nfloat\nRange: 0 - 999.99\n\n<12_Peak_EVM_All>   -  Overall offset error vector magnitude for complete PPDU, peak value\nfloat\nRange: 0 - 999.99\n\n<13_LoLeakage>   -  Local oscillator leakage\nfloat\nRange: -99.99 - 99.99\n\nAvailable Repeated Capabilities:\ninstance: i0, i1, i2, i3, i4, i5, i6, i7, i8, i9, i10, i11, i12, i13, i14, i15, i16, i17, i18, i19, i20, i21, i22, i23, i24, i25, i26, i27, i28, i29, i30, i31, i32\r\n\nRemote-control command(s):\nCALCulate:WPAN:MEAS<i>:MEValuation:MODulation:ABSolute:MAXimum?"}, {"Level"=4, "Class Only"=FALSE, "Identifier"="RSCMPLRWM_ATTR_HIDDEN_QUERY_MULTIEVAL_MODULATION_ABSOLUTE_STANDARD_DEVIATION_LIMIT_CHECK_RESULTS", "Descriptive Name"="Query MultiEval Modulation Absolute Standard Deviation Limit Check Results", "Data Type"=6, "Command"="CALC:WPAN:MEAS{instance}:MEV:MOD:ABS:SDEV?", "Access"=0, "Range Table"="", "Read Callback"="", "Write Callback"="", "Supported Models"="", "Instrument Options"="", "Flags"=8, "Help"="Returns the absolute standard deviation limit check single value results.\n\nReturn values:\n<1_Reliability>   - Reliability indicator\nfloat\n\n<2_OutOfTol>   -  Out of tolerance results\nfloat\nRange: 0 - 100\n\n<3_AveragePower>   - Average burst power\nfloat\nRange: -99.99 - 99.99\n\n<4_SymbolRateErr>   - Symbol rate error\nfloat\nRange: -1000 - 1000\n\n<5_FreqTolerance>   -  Frequency accuracy\nfloat\nRange: -1000 - 1000\n\n<6_FreqAccuracy>   -  Frequency accuracy\nfloat\nRange: -0.99999E+6 - 0.99999E+6\n\n<7_RMS_EVM_PS>   -  Offset error vector magnitude within PSDU portion, RMS value\nfloat\nRange: 0 -100\n\n<8_Peak_EVM_PS>   -  Offset error vector magnitude within PSDU portion,  peak value\nfloat\nRange: 0 - 100\n\n<9_RMS_EVM_SP>   -  Offset error vector magnitude within SHR + PHR portion, RMS value\nfloat\nRange: 0 - 999.99\n\n<10_Peak_EVM_SP>   -  Offset error vector magnitude within SHR + PHR portion, peak value\nfloat\nRange: 0 - 999.99\n\n<11_RMS_EVM_All>   -  Overall offset error vector magnitude for complete PPDU, RMS value\nfloat\nRange: 0 - 999.99\n\n<12_Peak_EVM_All>   -  Overall offset error vector magnitude for complete PPDU, peak value\nfloat\nRange: 0 - 999.99\n\n<13_LoLeakage>   -  Local oscillator leakage\nfloat\nRange: -99.99 - 99.99\n\nAvailable Repeated Capabilities:\ninstance: i0, i1, i2, i3, i4, i5, i6, i7, i8, i9, i10, i11, i12, i13, i14, i15, i16, i17, i18, i19, i20, i21, i22, i23, i24, i25, i26, i27, i28, i29, i30, i31, i32\r\n\nRemote-control command(s):\nCALCulate:WPAN:MEAS<i>:MEValuation:MODulation:ABSolute:SDEViation?"}, {"Level"=4, "Class Only"=FALSE, "Identifier"="RSCMPLRWM_ATTR_HIDDEN_FETCH_MULTIEVAL_MODULATION_ABSOLUTE_CURRENT_RESULTS", "Descriptive Name"="Fetch MultiEval Modulation Absolute Current Results", "Data Type"=6, "Command"="FETC:WPAN:MEAS{instance}:MEV:MOD:ABS:CURR?", "Access"=0, "Range Table"="", "Read Callback"="", "Write Callback"="", "Supported Models"="", "Instrument Options"="", "Flags"=8, "Help"="Returns the absolute current single value results.\n\nReturn values:\n<1_Reliability>   - Reliability indicator\nfloat\n\n<2_OutOfTol>   -  Out of tolerance result\nfloat\nRange: 0 - 100\n\n<3_AveragePower>   - Average burst power\nfloat\nRange: -99.99 - 99.99\n\n<4_SymbolRateErr>   - Symbol rate error\nfloat\nRange: -1000 - 1000\n\n<5_FreqTolerance>   -  Frequency accuracy\nfloat\nRange: -1000 - 1000\n\n<6_FreqAccuracy>   -  Frequency accuracy\nfloat\nRange: -0.99999E+6 - 0.99999E+6\n\n<7_RMS_EVM_PS>   -  Offset error vector magnitude within PSDU portion, RMS value\nfloat\nRange: 0 -100\n\n<8_Peak_EVM_PS>   -  Offset error vector magnitude within PSDU portion,  peak value\nfloat\nRange: 0 - 100\n\n<9_RMS_EVM_SP>   -  Offset error vector magnitude within SHR + PHR portion, RMS value\nfloat\nRange: 0 - 999.99\n\n<10_Peak_EVM_SP>   -  Offset error vector magnitude within SHR + PHR portion, peak value\nfloat\nRange: 0 - 999.99\n\n<11_RMS_EVM_All>   -  Overall offset error vector magnitude for complete PPDU, RMS value\nfloat\nRange: 0 - 999.99\n\n<12_Peak_EVM_All>   -  Overall offset error vector magnitude for complete PPDU, peak value\nfloat\nRange: 0 - 999.99\n\n<13_LoLeakage>   -  Local oscillator leakage\nfloat\nRange: -99.99 - 99.99\n\nAvailable Repeated Capabilities:\ninstance: i0, i1, i2, i3, i4, i5, i6, i7, i8, i9, i10, i11, i12, i13, i14, i15, i16, i17, i18, i19, i20, i21, i22, i23, i24, i25, i26, i27, i28, i29, i30, i31, i32\r\n\nRemote-control command(s):\nFETCh:WPAN:MEAS<i>:MEValuation:MODulation:ABSolute:CURRent?"}, {"Level"=4, "Class Only"=FALSE, "Identifier"="RSCMPLRWM_ATTR_HIDDEN_FETCH_MULTIEVAL_MODULATION_ABSOLUTE_AVERAGE_RESULTS", "Descriptive Name"="Fetch MultiEval Modulation Absolute Average Results", "Data Type"=6, "Command"="FETC:WPAN:MEAS{instance}:MEV:MOD:ABS:AVER?", "Access"=0, "Range Table"="", "Read Callback"="", "Write Callback"="", "Supported Models"="", "Instrument Options"="", "Flags"=8, "Help"="Returns the absolute average single value results.\n\nReturn values:\n<1_Reliability>   - Reliability indicator\nfloat\n\n<2_OutOfTol>   -  Out of tolerance result\nfloat\nRange: 0 - 100\n\n<3_AveragePower>   - Average burst power\nfloat\nRange: -99.99 - 99.99\n\n<4_SymbolRateErr>   - Symbol rate error\nfloat\nRange: -1000 - 1000\n\n<5_FreqTolerance>   -  Frequency accuracy\nfloat\nRange: -1000 - 1000\n\n<6_FreqAccuracy>   -  Frequency accuracy\nfloat\nRange: -0.99999E+6 - 0.99999E+6\n\n<7_RMS_EVM_PS>   -  Offset error vector magnitude within PSDU portion, RMS value\nfloat\nRange: 0 -100\n\n<8_Peak_EVM_PS>   -  Offset error vector magnitude within PSDU portion,  peak value\nfloat\nRange: 0 - 100\n\n<9_RMS_EVM_SP>   -  Offset error vector magnitude within SHR + PHR portion, RMS value\nfloat\nRange: 0 - 999.99\n\n<10_Peak_EVM_SP>   -  Offset error vector magnitude within SHR + PHR portion, peak value\nfloat\nRange: 0 - 999.99\n\n<11_RMS_EVM_All>   -  Overall offset error vector magnitude for complete PPDU, RMS value\nfloat\nRange: 0 - 999.99\n\n<12_Peak_EVM_All>   -  Overall offset error vector magnitude for complete PPDU, peak value\nfloat\nRange: 0 - 999.99\n\n<13_LoLeakage>   -  Local oscillator leakage\nfloat\nRange: -99.99 - 99.99\n\nAvailable Repeated Capabilities:\ninstance: i0, i1, i2, i3, i4, i5, i6, i7, i8, i9, i10, i11, i12, i13, i14, i15, i16, i17, i18, i19, i20, i21, i22, i23, i24, i25, i26, i27, i28, i29, i30, i31, i32\r\n\nRemote-control command(s):\nFETCh:WPAN:MEAS<i>:MEValuation:MODulation:ABSolute:AVERage?"}, {"Level"=4, "Class Only"=FALSE, "Identifier"="RSCMPLRWM_ATTR_HIDDEN_FETCH_MULTIEVAL_MODULATION_ABSOLUTE_MAXIMUM_RESULTS", "Descriptive Name"="Fetch MultiEval Modulation Absolute Maximum Results", "Data Type"=6, "Command"="FETC:WPAN:MEAS{instance}:MEV:MOD:ABS:MAX?", "Access"=0, "Range Table"="", "Read Callback"="", "Write Callback"="", "Supported Models"="", "Instrument Options"="", "Flags"=8, "Help"="Returns the absolute maximum single value results.\n\nReturn values:\n<1_Reliability>   - Reliability indicator\nfloat\n\n<2_OutOfTol>   -  Out of tolerance result\nfloat\nRange: 0 - 100\n\n<3_AveragePower>   - Average burst power\nfloat\nRange: -99.99 - 99.99\n\n<4_SymbolRateErr>   - Symbol rate error\nfloat\nRange: -1000 - 1000\n\n<5_FreqTolerance>   -  Frequency accuracy\nfloat\nRange: -1000 - 1000\n\n<6_FreqAccuracy>   -  Frequency accuracy\nfloat\nRange: -0.99999E+6 - 0.99999E+6\n\n<7_RMS_EVM_PS>   -  Offset error vector magnitude within PSDU portion, RMS value\nfloat\nRange: 0 -100\n\n<8_Peak_EVM_PS>   -  Offset error vector magnitude within PSDU portion,  peak value\nfloat\nRange: 0 - 100\n\n<9_RMS_EVM_SP>   -  Offset error vector magnitude within SHR + PHR portion, RMS value\nfloat\nRange: 0 - 999.99\n\n<10_Peak_EVM_SP>   -  Offset error vector magnitude within SHR + PHR portion, peak value\nfloat\nRange: 0 - 999.99\n\n<11_RMS_EVM_All>   -  Overall offset error vector magnitude for complete PPDU, RMS value\nfloat\nRange: 0 - 999.99\n\n<12_Peak_EVM_All>   -  Overall offset error vector magnitude for complete PPDU, peak value\nfloat\nRange: 0 - 999.99\n\n<13_LoLeakage>   -  Local oscillator leakage\nfloat\nRange: -99.99 - 99.99\n\nAvailable Repeated Capabilities:\ninstance: i0, i1, i2, i3, i4, i5, i6, i7, i8, i9, i10, i11, i12, i13, i14, i15, i16, i17, i18, i19, i20, i21, i22, i23, i24, i25, i26, i27, i28, i29, i30, i31, i32\r\n\nRemote-control command(s):\nFETCh:WPAN:MEAS<i>:MEValuation:MODulation:ABSolute:MAXimum?"}, {"Level"=4, "Class Only"=FALSE, "Identifier"="RSCMPLRWM_ATTR_HIDDEN_FETCH_MULTIEVAL_MODULATION_ABSOLUTE_STANDARD_DEVIATION_RESULTS", "Descriptive Name"="Fetch MultiEval Modulation Absolute Standard Deviation Results", "Data Type"=6, "Command"="FETC:WPAN:MEAS{instance}:MEV:MOD:ABS:SDEV?", "Access"=0, "Range Table"="", "Read Callback"="", "Write Callback"="", "Supported Models"="", "Instrument Options"="", "Flags"=8, "Help"="Returns the absolute standard deviation single value results.\n\nReturn values:\n<1_Reliability>   - Reliability indicator\nfloat\n\n<2_OutOfTol>   -  Out of tolerance result\nfloat\nRange: 0 - 100\n\n<3_AveragePower>   - Average burst power\nfloat\nRange: -99.99 - 99.99\n\n<4_SymbolRateErr>   - Symbol rate error\nfloat\nRange: -1000 - 1000\n\n<5_FreqTolerance>   -  Frequency accuracy\nfloat\nRange: -1000 - 1000\n\n<6_FreqAccuracy>   -  Frequency accuracy\nfloat\nRange: -0.99999E+6 - 0.99999E+6\n\n<7_RMS_EVM_PS>   -  Offset error vector magnitude within PSDU portion, RMS value\nfloat\nRange: 0 -100\n\n<8_Peak_EVM_PS>   -  Offset error vector magnitude within PSDU portion,  peak value\nfloat\nRange: 0 - 100\n\n<9_RMS_EVM_SP>   -  Offset error vector magnitude within SHR + PHR portion, RMS value\nfloat\nRange: 0 - 999.99\n\n<10_Peak_EVM_SP>   -  Offset error vector magnitude within SHR + PHR portion, peak value\nfloat\nRange: 0 - 999.99\n\n<11_RMS_EVM_All>   -  Overall offset error vector magnitude for complete PPDU, RMS value\nfloat\nRange: 0 - 999.99\n\n<12_Peak_EVM_All>   -  Overall offset error vector magnitude for complete PPDU, peak value\nfloat\nRange: 0 - 999.99\n\n<13_LoLeakage>   -  Local oscillator leakage\nfloat\nRange: -99.99 - 99.99\n\nAvailable Repeated Capabilities:\ninstance: i0, i1, i2, i3, i4, i5, i6, i7, i8, i9, i10, i11, i12, i13, i14, i15, i16, i17, i18, i19, i20, i21, i22, i23, i24, i25, i26, i27, i28, i29, i30, i31, i32\r\n\nRemote-control command(s):\nFETCh:WPAN:MEAS<i>:MEValuation:MODulation:ABSolute:SDEViation?"}, {"Level"=4, "Class Only"=FALSE, "Identifier"="RSCMPLRWM_ATTR_HIDDEN_READ_MULTIEVAL_MODULATION_ABSOLUTE_CURRENT_RESULTS", "Descriptive Name"="Read MultiEval Modulation Absolute Current Results", "Data Type"=6, "Command"="READ:WPAN:MEAS{instance}:MEV:MOD:ABS:CURR?", "Access"=0, "Range Table"="", "Read Callback"="", "Write Callback"="", "Supported Models"="", "Instrument Options"="", "Flags"=8, "Help"="Starts a new single shot measurement and returns the absolute current single value results.\n\nReturn values:\n<1_Reliability>   - Reliability indicator\nfloat\n\n<2_OutOfTol>   -  Out of tolerance result\nfloat\nRange: 0 - 100\n\n<3_AveragePower>   - Average burst power\nfloat\nRange: -99.99 - 99.99\n\n<4_SymbolRateErr>   - Symbol rate error\nfloat\nRange: -1000 - 1000\n\n<5_FreqTolerance>   -  Frequency accuracy\nfloat\nRange: -1000 - 1000\n\n<6_FreqAccuracy>   -  Frequency accuracy\nfloat\nRange: -0.99999E+6 - 0.99999E+6\n\n<7_RMS_EVM_PS>   -  Offset error vector magnitude within PSDU portion, RMS value\nfloat\nRange: 0 -100\n\n<8_Peak_EVM_PS>   -  Offset error vector magnitude within PSDU portion,  peak value\nfloat\nRange: 0 - 100\n\n<9_RMS_EVM_SP>   -  Offset error vector magnitude within SHR + PHR portion, RMS value\nfloat\nRange: 0 - 999.99\n\n<10_Peak_EVM_SP>   -  Offset error vector magnitude within SHR + PHR portion, peak value\nfloat\nRange: 0 - 999.99\n\n<11_RMS_EVM_All>   -  Overall offset error vector magnitude for complete PPDU, RMS value\nfloat\nRange: 0 - 999.99\n\n<12_Peak_EVM_All>   -  Overall offset error vector magnitude for complete PPDU, peak value\nfloat\nRange: 0 - 999.99\n\n<13_LoLeakage>   -  Local oscillator leakage\nfloat\nRange: -99.99 - 99.99\n\nAvailable Repeated Capabilities:\ninstance: i0, i1, i2, i3, i4, i5, i6, i7, i8, i9, i10, i11, i12, i13, i14, i15, i16, i17, i18, i19, i20, i21, i22, i23, i24, i25, i26, i27, i28, i29, i30, i31, i32\r\n\nRemote-control command(s):\nREAD:WPAN:MEAS<i>:MEValuation:MODulation:ABSolute:CURRent?"}, {"Level"=4, "Class Only"=FALSE, "Identifier"="RSCMPLRWM_ATTR_HIDDEN_READ_MULTIEVAL_MODULATION_ABSOLUTE_AVERAGE_RESULTS", "Descriptive Name"="Read MultiEval Modulation Absolute Average Results", "Data Type"=6, "Command"="READ:WPAN:MEAS{instance}:MEV:MOD:ABS:AVER?", "Access"=0, "Range Table"="", "Read Callback"="", "Write Callback"="", "Supported Models"="", "Instrument Options"="", "Flags"=8, "Help"="Starts a new single shot measurement and returns the absolute average single value results.\n\nReturn values:\n<1_Reliability>   - Reliability indicator\nfloat\n\n<2_OutOfTol>   -  Out of tolerance result\nfloat\nRange: 0 - 100\n\n<3_AveragePower>   - Average burst power\nfloat\nRange: -99.99 - 99.99\n\n<4_SymbolRateErr>   - Symbol rate error\nfloat\nRange: -1000 - 1000\n\n<5_FreqTolerance>   -  Frequency accuracy\nfloat\nRange: -1000 - 1000\n\n<6_FreqAccuracy>   -  Frequency accuracy\nfloat\nRange: -0.99999E+6 - 0.99999E+6\n\n<7_RMS_EVM_PS>   -  Offset error vector magnitude within PSDU portion, RMS value\nfloat\nRange: 0 -100\n\n<8_Peak_EVM_PS>   -  Offset error vector magnitude within PSDU portion,  peak value\nfloat\nRange: 0 - 100\n\n<9_RMS_EVM_SP>   -  Offset error vector magnitude within SHR + PHR portion, RMS value\nfloat\nRange: 0 - 999.99\n\n<10_Peak_EVM_SP>   -  Offset error vector magnitude within SHR + PHR portion, peak value\nfloat\nRange: 0 - 999.99\n\n<11_RMS_EVM_All>   -  Overall offset error vector magnitude for complete PPDU, RMS value\nfloat\nRange: 0 - 999.99\n\n<12_Peak_EVM_All>   -  Overall offset error vector magnitude for complete PPDU, peak value\nfloat\nRange: 0 - 999.99\n\n<13_LoLeakage>   -  Local oscillator leakage\nfloat\nRange: -99.99 - 99.99\n\nAvailable Repeated Capabilities:\ninstance: i0, i1, i2, i3, i4, i5, i6, i7, i8, i9, i10, i11, i12, i13, i14, i15, i16, i17, i18, i19, i20, i21, i22, i23, i24, i25, i26, i27, i28, i29, i30, i31, i32\r\n\nRemote-control command(s):\nREAD:WPAN:MEAS<i>:MEValuation:MODulation:ABSolute:AVERage?"}, {"Level"=4, "Class Only"=FALSE, "Identifier"="RSCMPLRWM_ATTR_HIDDEN_READ_MULTIEVAL_MODULATION_ABSOLUTE_MAXIMUM_RESULTS", "Descriptive Name"="Read MultiEval Modulation Absolute Maximum Results", "Data Type"=6, "Command"="READ:WPAN:MEAS{instance}:MEV:MOD:ABS:MAX?", "Access"=0, "Range Table"="", "Read Callback"="", "Write Callback"="", "Supported Models"="", "Instrument Options"="", "Flags"=8, "Help"="Starts a new single shot measurement and returns the absolute maximum single value results.\n\nReturn values:\n<1_Reliability>   - Reliability indicator\nfloat\n\n<2_OutOfTol>   -  Out of tolerance result\nfloat\nRange: 0 - 100\n\n<3_AveragePower>   - Average burst power\nfloat\nRange: -99.99 - 99.99\n\n<4_SymbolRateErr>   - Symbol rate error\nfloat\nRange: -1000 - 1000\n\n<5_FreqTolerance>   -  Frequency accuracy\nfloat\nRange: -1000 - 1000\n\n<6_FreqAccuracy>   -  Frequency accuracy\nfloat\nRange: -0.99999E+6 - 0.99999E+6\n\n<7_RMS_EVM_PS>   -  Offset error vector magnitude within PSDU portion, RMS value\nfloat\nRange: 0 -100\n\n<8_Peak_EVM_PS>   -  Offset error vector magnitude within PSDU portion,  peak value\nfloat\nRange: 0 - 100\n\n<9_RMS_EVM_SP>   -  Offset error vector magnitude within SHR + PHR portion, RMS value\nfloat\nRange: 0 - 999.99\n\n<10_Peak_EVM_SP>   -  Offset error vector magnitude within SHR + PHR portion, peak value\nfloat\nRange: 0 - 999.99\n\n<11_RMS_EVM_All>   -  Overall offset error vector magnitude for complete PPDU, RMS value\nfloat\nRange: 0 - 999.99\n\n<12_Peak_EVM_All>   -  Overall offset error vector magnitude for complete PPDU, peak value\nfloat\nRange: 0 - 999.99\n\n<13_LoLeakage>   -  Local oscillator leakage\nfloat\nRange: -99.99 - 99.99\n\nAvailable Repeated Capabilities:\ninstance: i0, i1, i2, i3, i4, i5, i6, i7, i8, i9, i10, i11, i12, i13, i14, i15, i16, i17, i18, i19, i20, i21, i22, i23, i24, i25, i26, i27, i28, i29, i30, i31, i32\r\n\nRemote-control command(s):\nREAD:WPAN:MEAS<i>:MEValuation:MODulation:ABSolute:MAXimum?"}, {"Level"=4, "Class Only"=FALSE, "Identifier"="RSCMPLRWM_ATTR_HIDDEN_READ_MULTIEVAL_MODULATION_ABSOLUTE_STANDARD_DEVIATION_RESULTS", "Descriptive Name"="Read MultiEval Modulation Absolute Standard Deviation Results", "Data Type"=6, "Command"="READ:WPAN:MEAS{instance}:MEV:MOD:ABS:SDEV?", "Access"=0, "Range Table"="", "Read Callback"="", "Write Callback"="", "Supported Models"="", "Instrument Options"="", "Flags"=8, "Help"="Starts a new single shot measurement and returns the absolute standard deviation single value results.\n\nReturn values:\n<1_Reliability>   - Reliability indicator\nfloat\n\n<2_OutOfTol>   -  Out of tolerance result\nfloat\nRange: 0 - 100s\n\n<3_AveragePower>   - Average burst power\nfloat\nRange: -99.99 - 99.99\n\n<4_SymbolRateErr>   - Symbol rate error\nfloat\nRange: -1000 - 1000\n\n<5_FreqTolerance>   -  Frequency accuracy\nfloat\nRange: -1000 - 1000\n\n<6_FreqAccuracy>   -  Frequency accuracy\nfloat\nRange: -0.99999E+6 - 0.99999E+6\n\n<7_RMS_EVM_PS>   -  Offset error vector magnitude within PSDU portion, RMS value\nfloat\nRange: 0 -100\n\n<8_Peak_EVM_PS>   -  Offset error vector magnitude within PSDU portion,  peak value\nfloat\nRange: 0 - 100\n\n<9_RMS_EVM_SP>   -  Offset error vector magnitude within SHR + PHR portion, RMS value\nfloat\nRange: 0 - 999.99\n\n<10_Peak_EVM_SP>   -  Offset error vector magnitude within SHR + PHR portion, peak value\nfloat\nRange: 0 - 999.99\n\n<11_RMS_EVM_All>   -  Overall offset error vector magnitude for complete PPDU, RMS value\nfloat\nRange: 0 - 999.99\n\n<12_Peak_EVM_All>   -  Overall offset error vector magnitude for complete PPDU, peak value\nfloat\nRange: 0 - 999.99\n\n<13_LoLeakage>   -  Local oscillator leakage\nfloat\nRange: -99.99 - 99.99\n\nAvailable Repeated Capabilities:\ninstance: i0, i1, i2, i3, i4, i5, i6, i7, i8, i9, i10, i11, i12, i13, i14, i15, i16, i17, i18, i19, i20, i21, i22, i23, i24, i25, i26, i27, i28, i29, i30, i31, i32\r\n\nRemote-control command(s):\nREAD:WPAN:MEAS<i>:MEValuation:MODulation:ABSolute:SDEViation?"}, {"Level"=3, "Class Only"=TRUE, "Identifier"="", "Descriptive Name"="Power", "Data Type"=0, "Command"="", "Access"=0, "Range Table"="", "Read Callback"="", "Write Callback"="", "Supported Models"="", "Instrument Options"="", "Flags"=0, "Help"="The following attributes return the power vs time results."}, {"Level"=4, "Class Only"=FALSE, "Identifier"="RSCMPLRWM_ATTR_HIDDEN_QUERY_MULTIEVAL_PVT_CURRENT_LIMIT_CHECK_RESULTS", "Descriptive Name"="Query MultiEval PVT Current Limit Check Results", "Data Type"=6, "Command"="CALC:WPAN:MEAS{instance}:MEV:PVT:CURR?", "Access"=0, "Range Table"="", "Read Callback"="", "Write Callback"="", "Supported Models"="", "Instrument Options"="", "Flags"=8, "Help"="Returns the limit check for current power vs time results.\n\nReturned values:\n<Reliability>   - Reliability indicator\ndecimal\n\n<BurstOutOfTol>   - Out of tolerance result,\nfloat | ON | OFF\nRange: 0 - 100\n\n<AveragePower>   - Average transmit power of the DUT\nfloat\nRange: -128 - 30\n\n<TrigToPpduStart>   - Trigger to packet start timing\nfloat\nRange: -5 - 5\n\nAvailable Repeated Capabilities:\ninstance: i0, i1, i2, i3, i4, i5, i6, i7, i8, i9, i10, i11, i12, i13, i14, i15, i16, i17, i18, i19, i20, i21, i22, i23, i24, i25, i26, i27, i28, i29, i30, i31, i32\r\n\nRemote-control command(s):\nCALCulate:WPAN:MEAS<i>:MEValuation:PVTime:CURRent?"}, {"Level"=4, "Class Only"=FALSE, "Identifier"="RSCMPLRWM_ATTR_HIDDEN_QUERY_MULTIEVAL_PVT_AVERAGE_LIMIT_CHECK_RESULTS", "Descriptive Name"="Query MultiEval PVT Average Limit Check Results", "Data Type"=6, "Command"="CALC:WPAN:MEAS{instance}:MEV:PVT:AVER?", "Access"=0, "Range Table"="", "Read Callback"="", "Write Callback"="", "Supported Models"="", "Instrument Options"="", "Flags"=8, "Help"="Returns the limit check for average power vs time results.\n\nReturned values:\n<Reliability>   - Reliability indicator\ndecimal\n\n<BurstOutOfTol>   - Out of tolerance result,\nfloat | ON | OFF\nRange: 0 - 100\n\n<AveragePower>   - Average transmit power of the DUT\nfloat\nRange: -128 - 30\n\n<TrigToPpduStart>   - Trigger to packet start timing\nfloat\nRange: -5 - 5\n\nAvailable Repeated Capabilities:\ninstance: i0, i1, i2, i3, i4, i5, i6, i7, i8, i9, i10, i11, i12, i13, i14, i15, i16, i17, i18, i19, i20, i21, i22, i23, i24, i25, i26, i27, i28, i29, i30, i31, i32\r\n\nRemote-control command(s):\nCALCulate:WPAN:MEAS<i>:MEValuation:PVTime:AVERage?"}, {"Level"=4, "Class Only"=FALSE, "Identifier"="RSCMPLRWM_ATTR_HIDDEN_QUERY_MULTIEVAL_PVT_MAXIMUM_LIMIT_CHECK_RESULTS", "Descriptive Name"="Query MultiEval PVT Maximum Limit Check Results", "Data Type"=6, "Command"="CALC:WPAN:MEAS{instance}:MEV:PVT:MAX?", "Access"=0, "Range Table"="", "Read Callback"="", "Write Callback"="", "Supported Models"="", "Instrument Options"="", "Flags"=8, "Help"="Returns the limit check for maximum power vs time results.\n\nReturned values:\n<Reliability>   - Reliability indicator\ndecimal\n\n<BurstOutOfTol>   - Out of tolerance result,\nfloat | ON | OFF\nRange: 0 - 100\n\n<AveragePower>   - Average transmit power of the DUT\nfloat\nRange: -128 - 30\n\n<TrigToPpduStart>   - Trigger to packet start timing\nfloat\nRange: -5 - 5\n\nAvailable Repeated Capabilities:\ninstance: i0, i1, i2, i3, i4, i5, i6, i7, i8, i9, i10, i11, i12, i13, i14, i15, i16, i17, i18, i19, i20, i21, i22, i23, i24, i25, i26, i27, i28, i29, i30, i31, i32\r\n\nRemote-control command(s):\nCALCulate:WPAN:MEAS<i>:MEValuation:PVTime:MAXimum?"}, {"Level"=4, "Class Only"=FALSE, "Identifier"="RSCMPLRWM_ATTR_HIDDEN_QUERY_MULTIEVAL_PVT_MINIMUM_LIMIT_CHECK_RESULTS", "Descriptive Name"="Query MultiEval PVT Minimum Limit Check Results", "Data Type"=6, "Command"="CALC:WPAN:MEAS{instance}:MEV:PVT:MIN?", "Access"=0, "Range Table"="", "Read Callback"="", "Write Callback"="", "Supported Models"="", "Instrument Options"="", "Flags"=8, "Help"="Returns the limit check for minimum power vs time results.\n\nReturned values:\n<Reliability>   - Reliability indicator\ndecimal\n\n<BurstOutOfTol>   - Out of tolerance result,\nfloat | ON | OFF\nRange: 0 - 100\n\n<AveragePower>   - Average transmit power of the DUT\nfloat\nRange: -128 - 30\n\n<TrigToPpduStart>   - Trigger to packet start timing\nfloat\nRange: -5 - 5\n\nAvailable Repeated Capabilities:\ninstance: i0, i1, i2, i3, i4, i5, i6, i7, i8, i9, i10, i11, i12, i13, i14, i15, i16, i17, i18, i19, i20, i21, i22, i23, i24, i25, i26, i27, i28, i29, i30, i31, i32\r\n\nRemote-control command(s):\nCALCulate:WPAN:MEAS<i>:MEValuation:PVTime:MINimum?"}, {"Level"=4, "Class Only"=FALSE, "Identifier"="RSCMPLRWM_ATTR_HIDDEN_FETCH_MULTIEVAL_PVT_CURRENT_RESULTS", "Descriptive Name"="Fetch MultiEval PVT Current Results", "Data Type"=6, "Command"="FETC:WPAN:MEAS{instance}:MEV:PVT:CURR?", "Access"=0, "Range Table"="", "Read Callback"="", "Write Callback"="", "Supported Models"="", "Instrument Options"="", "Flags"=8, "Help"="Returns the current power vs time results.\n\nReturned values:\n<Reliability>   - Reliability indicator\ndecimal\n\n<BurstOutOfTol>   - Out of tolerance result,\nfloat | ON | OFF\nRange: 0 - 100\n\n<AveragePower>   - Average transmit power of the DUT\nfloat\nRange: -128 - 30\n\n<TrigToPpduStart>   - Trigger to packet start timing\nfloat\nRange: -5 - 5\n\nAvailable Repeated Capabilities:\ninstance: i0, i1, i2, i3, i4, i5, i6, i7, i8, i9, i10, i11, i12, i13, i14, i15, i16, i17, i18, i19, i20, i21, i22, i23, i24, i25, i26, i27, i28, i29, i30, i31, i32\r\n\nRemote-control command(s):\nFETCh:WPAN:MEAS<i>:MEValuation:PVTime:CURRent?"}, {"Level"=4, "Class Only"=FALSE, "Identifier"="RSCMPLRWM_ATTR_HIDDEN_FETCH_MULTIEVAL_PVT_AVERAGE_RESULTS", "Descriptive Name"="Fetch MultiEval PVT Average Results", "Data Type"=6, "Command"="FETC:WPAN:MEAS{instance}:MEV:PVT:AVER?", "Access"=0, "Range Table"="", "Read Callback"="", "Write Callback"="", "Supported Models"="", "Instrument Options"="", "Flags"=8, "Help"="Returns the average power vs time results.\n\nReturned values:\n<Reliability>   - Reliability indicator\ndecimal\n\n<BurstOutOfTol>   - Out of tolerance result,\nfloat | ON | OFF\nRange: 0 - 100\n\n<AveragePower>   - Average transmit power of the DUT\nfloat\nRange: -128 - 30\n\n<TrigToPpduStart>   - Trigger to packet start timing\nfloat\nRange: -5 - 5\n\nAvailable Repeated Capabilities:\ninstance: i0, i1, i2, i3, i4, i5, i6, i7, i8, i9, i10, i11, i12, i13, i14, i15, i16, i17, i18, i19, i20, i21, i22, i23, i24, i25, i26, i27, i28, i29, i30, i31, i32\r\n\nRemote-control command(s):\nFETCh:WPAN:MEAS<i>:MEValuation:PVTime:AVERage?"}, {"Level"=4, "Class Only"=FALSE, "Identifier"="RSCMPLRWM_ATTR_HIDDEN_FETCH_MULTIEVAL_PVT_MAXIMUM_RESULTS", "Descriptive Name"="Fetch MultiEval PVT Maximum Results", "Data Type"=6, "Command"="FETC:WPAN:MEAS{instance}:MEV:PVT:MAX?", "Access"=0, "Range Table"="", "Read Callback"="", "Write Callback"="", "Supported Models"="", "Instrument Options"="", "Flags"=8, "Help"="Returns the maximum power vs time results.\n\nReturned values:\n<Reliability>   - Reliability indicator\ndecimal\n\n<BurstOutOfTol>   - Out of tolerance result,\nfloat | ON | OFF\nRange: 0 - 100\n\n<AveragePower>   - Average transmit power of the DUT\nfloat\nRange: -128 - 30\n\n<TrigToPpduStart>   - Trigger to packet start timing\nfloat\nRange: -5 - 5\n\nAvailable Repeated Capabilities:\ninstance: i0, i1, i2, i3, i4, i5, i6, i7, i8, i9, i10, i11, i12, i13, i14, i15, i16, i17, i18, i19, i20, i21, i22, i23, i24, i25, i26, i27, i28, i29, i30, i31, i32\r\n\nRemote-control command(s):\nFETCh:WPAN:MEAS<i>:MEValuation:PVTime:MAXimum?"}, {"Level"=4, "Class Only"=FALSE, "Identifier"="RSCMPLRWM_ATTR_HIDDEN_FETCH_MULTIEVAL_PVT_MINIMUM_RESULTS", "Descriptive Name"="Fetch MultiEval PVT Minimum Results", "Data Type"=6, "Command"="FETC:WPAN:MEAS{instance}:MEV:PVT:MIN?", "Access"=0, "Range Table"="", "Read Callback"="", "Write Callback"="", "Supported Models"="", "Instrument Options"="", "Flags"=8, "Help"="Returns the minimum power vs time results.\n\nReturned values:\n<Reliability>   - Reliability indicator\ndecimal\n\n<BurstOutOfTol>   - Out of tolerance result,\nfloat | ON | OFF\nRange: 0 - 100\n\n<AveragePower>   - Average transmit power of the DUT\nfloat\nRange: -128 - 30\n\n<TrigToPpduStart>   - Trigger to packet start timing\nfloat\nRange: -5 - 5\n\nAvailable Repeated Capabilities:\ninstance: i0, i1, i2, i3, i4, i5, i6, i7, i8, i9, i10, i11, i12, i13, i14, i15, i16, i17, i18, i19, i20, i21, i22, i23, i24, i25, i26, i27, i28, i29, i30, i31, i32\r\n\nRemote-control command(s):\nFETCh:WPAN:MEAS<i>:MEValuation:PVTime:MINimum?"}, {"Level"=4, "Class Only"=FALSE, "Identifier"="RSCMPLRWM_ATTR_HIDDEN_READ_MULTIEVAL_PVT_CURRENT_RESULTS", "Descriptive Name"="Read MultiEval PVT Current Results", "Data Type"=6, "Command"="READ:WPAN:MEAS{instance}:MEV:PVT:CURR?", "Access"=0, "Range Table"="", "Read Callback"="", "Write Callback"="", "Supported Models"="", "Instrument Options"="", "Flags"=8, "Help"="Starts a new single shot measurement and returns the current power vs time results.\n\nReturned values:\n<Reliability>   - Reliability indicator\ndecimal\n\n<BurstOutOfTol>   - Out of tolerance result,\nfloat | ON | OFF\nRange: 0 - 100\n\n<AveragePower>   - Average transmit power of the DUT\nfloat\nRange: -128 - 30\n\n<TrigToPpduStart>   - Trigger to packet start timing\nfloat\nRange: -5 - 5\n\nAvailable Repeated Capabilities:\ninstance: i0, i1, i2, i3, i4, i5, i6, i7, i8, i9, i10, i11, i12, i13, i14, i15, i16, i17, i18, i19, i20, i21, i22, i23, i24, i25, i26, i27, i28, i29, i30, i31, i32\r\n\nRemote-control command(s):\nREAD:WPAN:MEAS<i>:MEValuation:PVTime:CURRent?"}, {"Level"=4, "Class Only"=FALSE, "Identifier"="RSCMPLRWM_ATTR_HIDDEN_READ_MULTIEVAL_PVT_AVERAGE_RESULTS", "Descriptive Name"="Read MultiEval PVT Average Results", "Data Type"=6, "Command"="READ:WPAN:MEAS{instance}:MEV:PVT:AVER?", "Access"=0, "Range Table"="", "Read Callback"="", "Write Callback"="", "Supported Models"="", "Instrument Options"="", "Flags"=8, "Help"="Starts a new single shot measurement and returns the average power vs time results.\n\nReturned values:\n<Reliability>   - Reliability indicator\ndecimal\n\n<BurstOutOfTol>   - Out of tolerance result,\nfloat | ON | OFF\nRange: 0 - 100\n\n<AveragePower>   - Average transmit power of the DUT\nfloat\nRange: -128 - 30\n\n<TrigToPpduStart>   - Trigger to packet start timing\nfloat\nRange: -5 - 5\n\nAvailable Repeated Capabilities:\ninstance: i0, i1, i2, i3, i4, i5, i6, i7, i8, i9, i10, i11, i12, i13, i14, i15, i16, i17, i18, i19, i20, i21, i22, i23, i24, i25, i26, i27, i28, i29, i30, i31, i32\r\n\nRemote-control command(s):\nREAD:WPAN:MEAS<i>:MEValuation:PVTime:AVERage?"}, {"Level"=4, "Class Only"=FALSE, "Identifier"="RSCMPLRWM_ATTR_HIDDEN_READ_MULTIEVAL_PVT_MAXIMUM_RESULTS", "Descriptive Name"="Read MultiEval PVT Maximum Results", "Data Type"=6, "Command"="READ:WPAN:MEAS{instance}:MEV:PVT:MAX?", "Access"=0, "Range Table"="", "Read Callback"="", "Write Callback"="", "Supported Models"="", "Instrument Options"="", "Flags"=8, "Help"="Starts a new single shot measurement and returns the maximum power vs time results.\n\nReturned values:\n<Reliability>   - Reliability indicator\ndecimal\n\n<BurstOutOfTol>   - Out of tolerance result,\nfloat | ON | OFF\nRange: 0 - 100\n\n<AveragePower>   - Average transmit power of the DUT\nfloat\nRange: -128 - 30\n\n<TrigToPpduStart>   - Trigger to packet start timing\nfloat\nRange: -5 - 5\n\nAvailable Repeated Capabilities:\ninstance: i0, i1, i2, i3, i4, i5, i6, i7, i8, i9, i10, i11, i12, i13, i14, i15, i16, i17, i18, i19, i20, i21, i22, i23, i24, i25, i26, i27, i28, i29, i30, i31, i32\r\n\nRemote-control command(s):\nREAD:WPAN:MEAS<i>:MEValuation:PVTime:MAXimum?"}, {"Level"=4, "Class Only"=FALSE, "Identifier"="RSCMPLRWM_ATTR_HIDDEN_READ_MULTIEVAL_PVT_MINIMUM_RESULTS", "Descriptive Name"="Read MultiEval PVT Minimum Results", "Data Type"=6, "Command"="READ:WPAN:MEAS{instance}:MEV:PVT:MIN?", "Access"=0, "Range Table"="", "Read Callback"="", "Write Callback"="", "Supported Models"="", "Instrument Options"="", "Flags"=8, "Help"="Starts a new single shot measurement and returns the minimum power vs time results.\n\nReturned values:\n<Reliability>   - Reliability indicator\ndecimal\n\n<BurstOutOfTol>   - Out of tolerance result,\nfloat | ON | OFF\nRange: 0 - 100\n\n<AveragePower>   - Average transmit power of the DUT\nfloat\nRange: -128 - 30\n\n<TrigToPpduStart>   - Trigger to packet start timing\nfloat\nRange: -5 - 5\n\nAvailable Repeated Capabilities:\ninstance: i0, i1, i2, i3, i4, i5, i6, i7, i8, i9, i10, i11, i12, i13, i14, i15, i16, i17, i18, i19, i20, i21, i22, i23, i24, i25, i26, i27, i28, i29, i30, i31, i32\r\n\nRemote-control command(s):\nREAD:WPAN:MEAS<i>:MEValuation:PVTime:MINimum?"}, {"Level"=4, "Class Only"=FALSE, "Identifier"="RSCMPLRWM_ATTR_HIDDEN_FETCH_MULTIEVAL_PVT_CURRENT_TRACE_RESULTS", "Descriptive Name"="Fetch MultiEval PVT Current Trace Results", "Data Type"=6, "Command"="FETC:WPAN:MEAS{instance}:MEV:TRAC:PVT:CURR?", "Access"=0, "Range Table"="", "Read Callback"="", "Write Callback"="", "Supported Models"="", "Instrument Options"="", "Flags"=8, "Help"="Returns the power vs time traces. Eight values per chip are returned, starting from 500 st chip before the first chip to 500 st chip after the last chip in the burst.\n\nReturn values:\n<Reliability>   - Reliability indicator\ndecimal\n\n<PvT>   - Transmit power of the DUT\nfloat\nRange: -128 - 30\n\nAvailable Repeated Capabilities:\ninstance: i0, i1, i2, i3, i4, i5, i6, i7, i8, i9, i10, i11, i12, i13, i14, i15, i16, i17, i18, i19, i20, i21, i22, i23, i24, i25, i26, i27, i28, i29, i30, i31, i32\r\n\nRemote-control command(s):\nFETCh:WPAN:MEAS<i>:MEValuation:TRACe:PVTime:CURRent?"}, {"Level"=4, "Class Only"=FALSE, "Identifier"="RSCMPLRWM_ATTR_HIDDEN_FETCH_MULTIEVAL_PVT_AVERAGE_TRACE_RESULTS", "Descriptive Name"="Fetch MultiEval PVT Average Trace Results", "Data Type"=6, "Command"="FETC:WPAN:MEAS{instance}:MEV:TRAC:PVT:AVER?", "Access"=0, "Range Table"="", "Read Callback"="", "Write Callback"="", "Supported Models"="", "Instrument Options"="", "Flags"=8, "Help"="Returns the average power vs time traces. Eight values per chip are returned, starting from 500 st chip before the first chip to 500 st chip after the last chip in the burst.\n\nReturn values:\n<Reliability>   - Reliability indicator\ndecimal\n\n<PvT>   - Transmit power of the DUT\nfloat\nRange: -128 - 30\n\nAvailable Repeated Capabilities:\ninstance: i0, i1, i2, i3, i4, i5, i6, i7, i8, i9, i10, i11, i12, i13, i14, i15, i16, i17, i18, i19, i20, i21, i22, i23, i24, i25, i26, i27, i28, i29, i30, i31, i32\r\n\nRemote-control command(s):\nFETCh:WPAN:MEAS<i>:MEValuation:TRACe:PVTime:AVERage?"}, {"Level"=4, "Class Only"=FALSE, "Identifier"="RSCMPLRWM_ATTR_HIDDEN_FETCH_MULTIEVAL_PVT_MAXIMUM_TRACE_RESULTS", "Descriptive Name"="Fetch MultiEval PVT Maximum Trace Results", "Data Type"=6, "Command"="FETC:WPAN:MEAS{instance}:MEV:TRAC:PVT:MAX?", "Access"=0, "Range Table"="", "Read Callback"="", "Write Callback"="", "Supported Models"="", "Instrument Options"="", "Flags"=8, "Help"="Returns the maximum power vs time traces. Eight values per chip are returned, starting from 500 st chip before the first chip to 500 st chip after the last chip in the burst.\n\nReturn values:\n<Reliability>   - Reliability indicator\ndecimal\n\n<PvT>   - Transmit power of the DUT\nfloat\nRange: -128 - 30\n\nAvailable Repeated Capabilities:\ninstance: i0, i1, i2, i3, i4, i5, i6, i7, i8, i9, i10, i11, i12, i13, i14, i15, i16, i17, i18, i19, i20, i21, i22, i23, i24, i25, i26, i27, i28, i29, i30, i31, i32\r\n\nRemote-control command(s):\nFETCh:WPAN:MEAS<i>:MEValuation:TRACe:PVTime:MAXimum?"}, {"Level"=4, "Class Only"=FALSE, "Identifier"="RSCMPLRWM_ATTR_HIDDEN_FETCH_MULTIEVAL_PVT_MINIMUM_TRACE_RESULTS", "Descriptive Name"="Fetch MultiEval PVT Minimum Trace Results", "Data Type"=6, "Command"="FETC:WPAN:MEAS{instance}:MEV:TRAC:PVT:MIN?", "Access"=0, "Range Table"="", "Read Callback"="", "Write Callback"="", "Supported Models"="", "Instrument Options"="", "Flags"=8, "Help"="Returns the minimum power vs time traces. Eight values per chip are returned, starting from 500 st chip before the first chip to 500 st chip after the last chip in the burst.\n\nReturn values:\n<Reliability>   - Reliability indicator\ndecimal\n\n<PvT>   - Transmit power of the DUT\nfloat\nRange: -128 - 30\n\nAvailable Repeated Capabilities:\ninstance: i0, i1, i2, i3, i4, i5, i6, i7, i8, i9, i10, i11, i12, i13, i14, i15, i16, i17, i18, i19, i20, i21, i22, i23, i24, i25, i26, i27, i28, i29, i30, i31, i32\r\n\nRemote-control command(s):\nFETCh:WPAN:MEAS<i>:MEValuation:TRACe:PVTime:MINimum?"}, {"Level"=4, "Class Only"=FALSE, "Identifier"="RSCMPLRWM_ATTR_HIDDEN_READ_MULTIEVAL_PVT_CURRENT_TRACE_RESULTS", "Descriptive Name"="Read MultiEval PVT Current Trace Results", "Data Type"=6, "Command"="READ:WPAN:MEAS{instance}:MEV:TRAC:PVT:CURR?", "Access"=0, "Range Table"="", "Read Callback"="", "Write Callback"="", "Supported Models"="", "Instrument Options"="", "Flags"=8, "Help"="Starts a new single shot measurement and returns  the current power vs time traces. Eight values per chip are returned, starting from 500 st chip before the first chip to 500 st chip after the last chip in the burst.\n\nReturn values:\n<Reliability>   - Reliability indicator\ndecimal\n\n<PvT>   - Transmit power of the DUT\nfloat\nRange: -128 - 30\n\nAvailable Repeated Capabilities:\ninstance: i0, i1, i2, i3, i4, i5, i6, i7, i8, i9, i10, i11, i12, i13, i14, i15, i16, i17, i18, i19, i20, i21, i22, i23, i24, i25, i26, i27, i28, i29, i30, i31, i32\r\n\nRemote-control command(s):\nREAD:WPAN:MEAS<i>:MEValuation:TRACe:PVTime:CURRent?"}, {"Level"=4, "Class Only"=FALSE, "Identifier"="RSCMPLRWM_ATTR_HIDDEN_READ_MULTIEVAL_PVT_AVERAGE_TRACE_RESULTS", "Descriptive Name"="Read MultiEval PVT Average Trace Results", "Data Type"=6, "Command"="READ:WPAN:MEAS{instance}:MEV:TRAC:PVT:AVER?", "Access"=0, "Range Table"="", "Read Callback"="", "Write Callback"="", "Supported Models"="", "Instrument Options"="", "Flags"=8, "Help"="Starts a new single shot measurement and returns  the average power vs time traces. Eight values per chip are returned, starting from 500 st chip before the first chip to 500 st chip after the last chip in the burst.\n\nReturn values:\n<Reliability>   - Reliability indicator\ndecimal\n\n<PvT>   - Transmit power of the DUT\nfloat\nRange: -128 - 30\n\nAvailable Repeated Capabilities:\ninstance: i0, i1, i2, i3, i4, i5, i6, i7, i8, i9, i10, i11, i12, i13, i14, i15, i16, i17, i18, i19, i20, i21, i22, i23, i24, i25, i26, i27, i28, i29, i30, i31, i32\r\n\nRemote-control command(s):\nREAD:WPAN:MEAS<i>:MEValuation:TRACe:PVTime:AVERage?"}, {"Level"=4, "Class Only"=FALSE, "Identifier"="RSCMPLRWM_ATTR_HIDDEN_READ_MULTIEVAL_PVT_MAXIMUM_TRACE_RESULTS", "Descriptive Name"="Read MultiEval PVT Maximum Trace Results", "Data Type"=6, "Command"="READ:WPAN:MEAS{instance}:MEV:TRAC:PVT:MAX?", "Access"=0, "Range Table"="", "Read Callback"="", "Write Callback"="", "Supported Models"="", "Instrument Options"="", "Flags"=8, "Help"="Starts a new single shot measurement and returns  the maximum power vs time traces. Eight values per chip are returned, starting from 500 st chip before the first chip to 500 st chip after the last chip in the burst.\n\nReturn values:\n<Reliability>   - Reliability indicator\ndecimal\n\n<PvT>   - Transmit power of the DUT\nfloat\nRange: -128 - 30\n\nAvailable Repeated Capabilities:\ninstance: i0, i1, i2, i3, i4, i5, i6, i7, i8, i9, i10, i11, i12, i13, i14, i15, i16, i17, i18, i19, i20, i21, i22, i23, i24, i25, i26, i27, i28, i29, i30, i31, i32\r\n\nRemote-control command(s):\nREAD:WPAN:MEAS<i>:MEValuation:TRACe:PVTime:MAXimum?"}, {"Level"=4, "Class Only"=FALSE, "Identifier"="RSCMPLRWM_ATTR_HIDDEN_READ_MULTIEVAL_PVT_MINIMUM_TRACE_RESULTS", "Descriptive Name"="Read MultiEval PVT Minimum Trace Results", "Data Type"=6, "Command"="READ:WPAN:MEAS{instance}:MEV:TRAC:PVT:MIN?", "Access"=0, "Range Table"="", "Read Callback"="", "Write Callback"="", "Supported Models"="", "Instrument Options"="", "Flags"=8, "Help"="Starts a new single shot measurement and returns  the minimum power vs time traces. Eight values per chip are returned, starting from 500 st chip before the first chip to 500 st chip after the last chip in the burst.\n\nReturn values:\n<Reliability>   - Reliability indicator\ndecimal\n\n<PvT>   - Transmit power of the DUT\nfloats\nRange: -128 - 30\n\nAvailable Repeated Capabilities:\ninstance: i0, i1, i2, i3, i4, i5, i6, i7, i8, i9, i10, i11, i12, i13, i14, i15, i16, i17, i18, i19, i20, i21, i22, i23, i24, i25, i26, i27, i28, i29, i30, i31, i32\r\n\nRemote-control command(s):\nREAD:WPAN:MEAS<i>:MEValuation:TRACe:PVTime:MINimum?"}, {"Level"=3, "Class Only"=TRUE, "Identifier"="", "Descriptive Name"="Spectrum", "Data Type"=0, "Command"="", "Access"=0, "Range Table"="", "Read Callback"="", "Write Callback"="", "Supported Models"="", "Instrument Options"="", "Flags"=0, "Help"="The following attributes return spectrum results."}, {"Level"=4, "Class Only"=FALSE, "Identifier"="RSCMPLRWM_ATTR_HIDDEN_QUERY_MULTIEVAL_SPECTRUM_AVERAGE_LIMIT_CHECK_RESULTS", "Descriptive Name"="Query MultiEval Spectrum Average Limit Check Results", "Data Type"=6, "Command"="CALC:WPAN:MEAS{instance}:MEV:SPEC:AVER?", "Access"=0, "Range Table"="", "Read Callback"="", "Write Callback"="", "Supported Models"="", "Instrument Options"="", "Flags"=8, "Help"="Returns the average limit check results. Returns string of 22 single values.\n\nReturned values:\n<1_Reliability>   - Reliability indicator\ndecimal\n\n<2_BurstOutOfTol>   - Out of tolerance result\nfloat | ON | OFF\nRange: 0 - 100\n\n<3_AveragePower>  - Average burst power\nfloat\nRange: -99.99 - 99.99\n\n<5_Margin1> ... <7_Margin3>\nfloat\nRange: -99.99 - 99.99\nThree margins (three worst values) between power spectral density trace and spectrum limit line for relative frequencies f < 0 (lesser than the frequency of central channel). A negative result indicates that the trace is located above the limit line, i.e. the limit is exceeded.\n\n\n<8_Margin4> ... <10_Margin6>\nfloat\nRange: -99.99 - 99.99\nThree margins (three worst values) between power spectral density trace and spectrum limit line for relative frequencies f > 0 (greater than the frequency of central channel). A negative result indicates that the trace is located above the limit line, i.e. the limit is exceeded.\n\n<11_Signal_Level1> ... <16_Signal_Level6>\nfloat\nRange: -99.99 - 99.99\nLevel of received signal measured in margin points 1 to 6.\n\n<17_Frequency1> ... <22_Frequency6>\nfloat\nRange: -9999 - 9999\nFrequency offsets between the margin points 1 to 6 and the channel center frequency.\n\nAvailable Repeated Capabilities:\ninstance: i0, i1, i2, i3, i4, i5, i6, i7, i8, i9, i10, i11, i12, i13, i14, i15, i16, i17, i18, i19, i20, i21, i22, i23, i24, i25, i26, i27, i28, i29, i30, i31, i32\r\n\nRemote-control command(s):\nCALCulate:WPAN:MEAS<i>:MEValuation:SPECtrum:AVERage?"}, {"Level"=4, "Class Only"=FALSE, "Identifier"="RSCMPLRWM_ATTR_HIDDEN_FETCH_MULTIEVAL_SPECTRUM_AVERAGE_RESULTS", "Descriptive Name"="Fetch MultiEval Spectrum Average Results", "Data Type"=6, "Command"="FETC:WPAN:MEAS{instance}:MEV:SPEC:AVER?", "Access"=0, "Range Table"="", "Read Callback"="", "Write Callback"="", "Supported Models"="", "Instrument Options"="", "Flags"=8, "Help"="Returns the average spectrum results. Returns string of 22 single values.\n\nReturned values:\n<1_Reliability>   - Reliability indicator\ndecimal\n\n<2_BurstOutOfTol>   - Out of tolerance result\nfloat | ON | OFF\nRange: 0 - 100\n\n<3_AveragePower>  - Average burst power\nfloat\nRange: -99.99 - 99.99\n\n<5_Margin1> ... <7_Margin3>\nfloat\nRange: -99.99 - 99.99\nThree margins (three worst values) between power spectral density trace and spectrum limit line for relative frequencies f < 0 (lesser than the frequency of central channel). A negative result indicates that the trace is located above the limit line, i.e. the limit is exceeded.\n\n\n<8_Margin4> ... <10_Margin6>\nfloat\nRange: -99.99 - 99.99\nThree margins (three worst values) between power spectral density trace and spectrum limit line for relative frequencies f > 0 (greater than the frequency of central channel). A negative result indicates that the trace is located above the limit line, i.e. the limit is exceeded.\n\n<11_Signal_Level1> ... <16_Signal_Level6>\nfloat\nRange: -99.99 - 99.99\nLevel of received signal measured in margin points 1 to 6.\n\n<17_Frequency1> ... <22_Frequency6>\nfloat\nRange: -9999 - 9999\nFrequency offsets between the margin points 1 to 6 and the channel center frequency.\n\nAvailable Repeated Capabilities:\ninstance: i0, i1, i2, i3, i4, i5, i6, i7, i8, i9, i10, i11, i12, i13, i14, i15, i16, i17, i18, i19, i20, i21, i22, i23, i24, i25, i26, i27, i28, i29, i30, i31, i32\r\n\nRemote-control command(s):\nFETCh:WPAN:MEAS<i>:MEValuation:SPECtrum:AVERage?"}, {"Level"=4, "Class Only"=FALSE, "Identifier"="RSCMPLRWM_ATTR_HIDDEN_READ_MULTIEVAL_SPECTRUM_AVERAGE_RESULTS", "Descriptive Name"="Read MultiEval Spectrum Average Results", "Data Type"=6, "Command"="READ:WPAN:MEAS{instance}:MEV:SPEC:AVER?", "Access"=0, "Range Table"="", "Read Callback"="", "Write Callback"="", "Supported Models"="", "Instrument Options"="", "Flags"=8, "Help"="Starts a new single shot measurement and returns the average spectrum results. Returns string of 22 single values.\n\nReturned values:\n<1_Reliability>   - Reliability indicator\ndecimal\n\n<2_BurstOutOfTol>   - Out of tolerance result\nfloat | ON | OFF\nRange: 0 - 100\n\n<3_AveragePower>  - Average burst power\nfloat\nRange: -99.99 - 99.99\n\n<5_Margin1> ... <7_Margin3>\nfloat\nRange: -99.99 - 99.99\nThree margins (three worst values) between power spectral density trace and spectrum limit line for relative frequencies f < 0 (lesser than the frequency of central channel). A negative result indicates that the trace is located above the limit line, i.e. the limit is exceeded.\n\n\n<8_Margin4> ... <10_Margin6>\nfloat\nRange: -99.99 - 99.99\nThree margins (three worst values) between power spectral density trace and spectrum limit line for relative frequencies f > 0 (greater than the frequency of central channel). A negative result indicates that the trace is located above the limit line, i.e. the limit is exceeded.\n\n<11_Signal_Level1> ... <16_Signal_Level6>\nfloat\nRange: -99.99 - 99.99\nLevel of received signal measured in margin points 1 to 6.\n\n<17_Frequency1> ... <22_Frequency6>\nfloat\nRange: -9999 - 9999\nFrequency offsets between the margin points 1 to 6 and the channel center frequency.\n\nAvailable Repeated Capabilities:\ninstance: i0, i1, i2, i3, i4, i5, i6, i7, i8, i9, i10, i11, i12, i13, i14, i15, i16, i17, i18, i19, i20, i21, i22, i23, i24, i25, i26, i27, i28, i29, i30, i31, i32\r\n\nRemote-control command(s):\nREAD:WPAN:MEAS<i>:MEValuation:SPECtrum:AVERage?"}, {"Level"=4, "Class Only"=FALSE, "Identifier"="RSCMPLRWM_ATTR_HIDDEN_QUERY_MULTIEVAL_SPECTRUM_CURRENT_LIMIT_CHECK_RESULTS", "Descriptive Name"="Query MultiEval Spectrum Current Limit Check Results", "Data Type"=6, "Command"="CALC:WPAN:MEAS{instance}:MEV:SPEC:CURR?", "Access"=0, "Range Table"="", "Read Callback"="", "Write Callback"="", "Supported Models"="", "Instrument Options"="", "Flags"=8, "Help"="Returns the current spectrum limit check single results.\n\nReturned values:\n<Reliability>   - Reliability indicator\ndecimal\n\n<BurstOutOfTol>   - Out of tolerance result\nfloat | ON | OFF\nRange : 0 - 100\n\n<AveragePower>   - Average burst power\nfloat\nRange: -99.99 - 99.99\n\nAvailable Repeated Capabilities:\ninstance: i0, i1, i2, i3, i4, i5, i6, i7, i8, i9, i10, i11, i12, i13, i14, i15, i16, i17, i18, i19, i20, i21, i22, i23, i24, i25, i26, i27, i28, i29, i30, i31, i32\r\n\nRemote-control command(s):\nCALCulate:WPAN:MEAS<i>:MEValuation:SPECtrum:CURRent?"}, {"Level"=4, "Class Only"=FALSE, "Identifier"="RSCMPLRWM_ATTR_HIDDEN_QUERY_MULTIEVAL_SPECTRUM_MAXIMUM_LIMIT_CHECK_RESULTS", "Descriptive Name"="Query MultiEval Spectrum Maximum Limit Check Results", "Data Type"=6, "Command"="CALC:WPAN:MEAS{instance}:MEV:SPEC:MAX?", "Access"=0, "Range Table"="", "Read Callback"="", "Write Callback"="", "Supported Models"="", "Instrument Options"="", "Flags"=8, "Help"="Returns the maximum spectrum limit check single results.\n\nReturned values:\n<Reliability>   - Reliability indicator\ndecimal\n\n<BurstOutOfTol>   - Out of tolerance result\nfloat | ON | OFF\nRange : 0 - 100\n\n<AveragePower>   - Average burst power\nfloat\nRange: -99.99 - 99.99\n\nAvailable Repeated Capabilities:\ninstance: i0, i1, i2, i3, i4, i5, i6, i7, i8, i9, i10, i11, i12, i13, i14, i15, i16, i17, i18, i19, i20, i21, i22, i23, i24, i25, i26, i27, i28, i29, i30, i31, i32\r\n\nRemote-control command(s):\nCALCulate:WPAN:MEAS<i>:MEValuation:SPECtrum:MAXimum?"}, {"Level"=4, "Class Only"=FALSE, "Identifier"="RSCMPLRWM_ATTR_HIDDEN_FETCH_MULTIEVAL_SPECTRUM_CURRENT_RESULTS", "Descriptive Name"="Fetch MultiEval Spectrum Current Results", "Data Type"=6, "Command"="FETC:WPAN:MEAS{instance}:MEV:SPEC:CURR?", "Access"=0, "Range Table"="", "Read Callback"="", "Write Callback"="", "Supported Models"="", "Instrument Options"="", "Flags"=8, "Help"="Returns the current spectrum single results.\n\nReturned values:\n<Reliability>   - Reliability indicator\ndecimal\n\n<BurstOutOfTol>   - Out of tolerance result\nfloat | ON | OFF\nRange : 0 - 100\n\n<AveragePower>   - Average burst power\nfloat\nRange: -99.99 - 99.99\n\nAvailable Repeated Capabilities:\ninstance: i0, i1, i2, i3, i4, i5, i6, i7, i8, i9, i10, i11, i12, i13, i14, i15, i16, i17, i18, i19, i20, i21, i22, i23, i24, i25, i26, i27, i28, i29, i30, i31, i32\r\n\nRemote-control command(s):\nFETCh:WPAN:MEAS<i>:MEValuation:SPECtrum:CURRent?"}, {"Level"=4, "Class Only"=FALSE, "Identifier"="RSCMPLRWM_ATTR_HIDDEN_FETCH_MULTIEVAL_SPECTRUM_MAXIMUM_RESULTS", "Descriptive Name"="Fetch MultiEval Spectrum Maximum Results", "Data Type"=6, "Command"="FETC:WPAN:MEAS{instance}:MEV:SPEC:MAX?", "Access"=0, "Range Table"="", "Read Callback"="", "Write Callback"="", "Supported Models"="", "Instrument Options"="", "Flags"=8, "Help"="Returns the maximum spectrum single results.\n\nReturned values:\n<Reliability>   - Reliability indicator\ndecimal\n\n<BurstOutOfTol>   - Out of tolerance result\nfloat | ON | OFF\nRange : 0 - 100\n\n<AveragePower>   - Average burst power\nfloat\nRange: -99.99 - 99.99\n\nAvailable Repeated Capabilities:\ninstance: i0, i1, i2, i3, i4, i5, i6, i7, i8, i9, i10, i11, i12, i13, i14, i15, i16, i17, i18, i19, i20, i21, i22, i23, i24, i25, i26, i27, i28, i29, i30, i31, i32\r\n\nRemote-control command(s):\nFETCh:WPAN:MEAS<i>:MEValuation:SPECtrum:MAXimum?"}, {"Level"=4, "Class Only"=FALSE, "Identifier"="RSCMPLRWM_ATTR_HIDDEN_READ_MULTIEVAL_SPECTRUM_CURRENT_RESULTS", "Descriptive Name"="Read MultiEval Spectrum Current Results", "Data Type"=6, "Command"="READ:WPAN:MEAS{instance}:MEV:SPEC:CURR?", "Access"=0, "Range Table"="", "Read Callback"="", "Write Callback"="", "Supported Models"="", "Instrument Options"="", "Flags"=8, "Help"="Starts a new single shot measurement and returns the current spectrum results.\n\nReturned values:\n<Reliability>   - Reliability indicator\ndecimal\n\n<BurstOutOfTol>   - Out of tolerance result\nfloat | ON | OFF\nRange : 0 - 100\n\n<AveragePower>   - Average burst power\nfloat\nRange: -99.99 - 99.99\n\nAvailable Repeated Capabilities:\ninstance: i0, i1, i2, i3, i4, i5, i6, i7, i8, i9, i10, i11, i12, i13, i14, i15, i16, i17, i18, i19, i20, i21, i22, i23, i24, i25, i26, i27, i28, i29, i30, i31, i32\r\n\nRemote-control command(s):\nREAD:WPAN:MEAS<i>:MEValuation:SPECtrum:CURRent?"}, {"Level"=4, "Class Only"=FALSE, "Identifier"="RSCMPLRWM_ATTR_HIDDEN_READ_MULTIEVAL_SPECTRUM_MAXIMUM_RESULTS", "Descriptive Name"="Read MultiEval Spectrum Maximum Results", "Data Type"=6, "Command"="READ:WPAN:MEAS{instance}:MEV:SPEC:MAX?", "Access"=0, "Range Table"="", "Read Callback"="", "Write Callback"="", "Supported Models"="", "Instrument Options"="", "Flags"=8, "Help"="Starts a new single shot measurement and returns the maximum spectrum results.\n\nReturned values:\n<Reliability>   - Reliability indicator\ndecimal\n\n<BurstOutOfTol>   - Out of tolerance result\nfloat | ON | OFF\nRange : 0 - 100\n\n<AveragePower>   - Average burst power\nfloat\nRange: -99.99 - 99.99\n\nAvailable Repeated Capabilities:\ninstance: i0, i1, i2, i3, i4, i5, i6, i7, i8, i9, i10, i11, i12, i13, i14, i15, i16, i17, i18, i19, i20, i21, i22, i23, i24, i25, i26, i27, i28, i29, i30, i31, i32\r\n\nRemote-control command(s):\nREAD:WPAN:MEAS<i>:MEValuation:SPECtrum:MAXimum?"}, {"Level"=3, "Class Only"=TRUE, "Identifier"="", "Descriptive Name"="EVM vs Chip Trace Results", "Data Type"=0, "Command"="", "Access"=0, "Range Table"="", "Read Callback"="", "Write Callback"="", "Supported Models"="", "Instrument Options"="", "Flags"=0, "Help"="The commands in this class return the contents of the EVM vs chip result diagrams."}, {"Level"=4, "Class Only"=FALSE, "Identifier"="RSCMPLRWM_ATTR_HIDDEN_FETCH_MULTIEVAL_EVM_VS_CHIP_CURRENT_TRACE_RESULTS", "Descriptive Name"="Fetch MultiEval EVM vs Chip Current Trace Results", "Data Type"=6, "Command"="FETC:WPAN:MEAS{instance}:MEV:TRAC:EVMC:CURR?", "Access"=0, "Range Table"="", "Read Callback"="", "Write Callback"="", "Supported Models"="", "Instrument Options"="", "Flags"=8, "Help"="Returns the current offset EVM vs chip traces. One value per two chips within the PSDU is returned.\n\nReturn values:\n<Reliability>   - Reliability indicator\ndecimal\n\n<EVM>   - Offset error vector magnitude\nfloat\n\nAvailable Repeated Capabilities:\ninstance: i0, i1, i2, i3, i4, i5, i6, i7, i8, i9, i10, i11, i12, i13, i14, i15, i16, i17, i18, i19, i20, i21, i22, i23, i24, i25, i26, i27, i28, i29, i30, i31, i32\r\n\nRemote-control command(s):\nFETCh:WPAN:MEAS<i>:MEValuation:TRACe:EVMChip[:OFFSet]:CURRent?"}, {"Level"=4, "Class Only"=FALSE, "Identifier"="RSCMPLRWM_ATTR_HIDDEN_FETCH_MULTIEVAL_EVM_VS_CHIP_AVERAGE_TRACE_RESULTS", "Descriptive Name"="Fetch MultiEval EVM vs Chip Average Trace Results", "Data Type"=6, "Command"="FETC:WPAN:MEAS{instance}:MEV:TRAC:EVMC:AVER?", "Access"=0, "Range Table"="", "Read Callback"="", "Write Callback"="", "Supported Models"="", "Instrument Options"="", "Flags"=8, "Help"="Returns theverage offset EVM vs chip traces. One value per two chips within the PSDU is returned.\n\nReturn values:\n<Reliability>   - Reliability indicator\ndecimal\n\n<EVM>   - Offset error vector magnitude\nfloat\n\nAvailable Repeated Capabilities:\ninstance: i0, i1, i2, i3, i4, i5, i6, i7, i8, i9, i10, i11, i12, i13, i14, i15, i16, i17, i18, i19, i20, i21, i22, i23, i24, i25, i26, i27, i28, i29, i30, i31, i32\r\n\nRemote-control command(s):\nFETCh:WPAN:MEAS<i>:MEValuation:TRACe:EVMChip[:OFFSet]:AVERage?"}, {"Level"=4, "Class Only"=FALSE, "Identifier"="RSCMPLRWM_ATTR_HIDDEN_FETCH_MULTIEVAL_EVM_VS_CHIP_MAXIMUM_TRACE_RESULTS", "Descriptive Name"="Fetch MultiEval EVM vs Chip Maximum Trace Results", "Data Type"=6, "Command"="FETC:WPAN:MEAS{instance}:MEV:TRAC:EVMC:MAX?", "Access"=0, "Range Table"="", "Read Callback"="", "Write Callback"="", "Supported Models"="", "Instrument Options"="", "Flags"=8, "Help"="Returns the maximum offset EVM vs chip traces. One value per two chips within the PSDU is returned.\n\nReturn values:\n<Reliability>   - Reliability indicator\ndecimal\n\n<EVM>   - Offset error vector magnitudes\nfloat\n\nAvailable Repeated Capabilities:\ninstance: i0, i1, i2, i3, i4, i5, i6, i7, i8, i9, i10, i11, i12, i13, i14, i15, i16, i17, i18, i19, i20, i21, i22, i23, i24, i25, i26, i27, i28, i29, i30, i31, i32\r\n\nRemote-control command(s):\nFETCh:WPAN:MEAS<i>:MEValuation:TRACe:EVMChip[:OFFSet]:MAXimum?"}, {"Level"=4, "Class Only"=FALSE, "Identifier"="RSCMPLRWM_ATTR_HIDDEN_READ_MULTIEVAL_EVM_VS_CHIP_CURRENT_TRACE_RESULTS", "Descriptive Name"="Read MultiEval EVM vs Chip Current Trace Results", "Data Type"=6, "Command"="READ:WPAN:MEAS{instance}:MEV:TRAC:EVMC:CURR?", "Access"=0, "Range Table"="", "Read Callback"="", "Write Callback"="", "Supported Models"="", "Instrument Options"="", "Flags"=8, "Help"="Starts a single-shot measurement and returns the current offset EVM vs chip traces. One value per two chips within the PSDU is returned.\n\nReturn values:\n<Reliability>   - Reliability indicator\ndecimal\n\n<EVM>   - Offset error vector magnitude\nfloat\n\nAvailable Repeated Capabilities:\ninstance: i0, i1, i2, i3, i4, i5, i6, i7, i8, i9, i10, i11, i12, i13, i14, i15, i16, i17, i18, i19, i20, i21, i22, i23, i24, i25, i26, i27, i28, i29, i30, i31, i32\r\n\nRemote-control command(s):\nREAD:WPAN:MEAS<i>:MEValuation:TRACe:EVMChip[:OFFSet]:CURRent?"}, {"Level"=4, "Class Only"=FALSE, "Identifier"="RSCMPLRWM_ATTR_HIDDEN_READ_MULTIEVAL_EVM_VS_CHIP_AVERAGE_TRACE_RESULTS", "Descriptive Name"="Read MultiEval EVM vs Chip Average Trace Results", "Data Type"=6, "Command"="READ:WPAN:MEAS{instance}:MEV:TRAC:EVMC:AVER?", "Access"=0, "Range Table"="", "Read Callback"="", "Write Callback"="", "Supported Models"="", "Instrument Options"="", "Flags"=8, "Help"="Starts a single-shot measurement and returns the average offset EVM vs chip traces. One value per two chips within the PSDU is returned.\n\nReturn values:\n<Reliability>   - Reliability indicator\ndecimal\n\n<EVM>   - Offset error vector magnitude\nfloat\n\nAvailable Repeated Capabilities:\ninstance: i0, i1, i2, i3, i4, i5, i6, i7, i8, i9, i10, i11, i12, i13, i14, i15, i16, i17, i18, i19, i20, i21, i22, i23, i24, i25, i26, i27, i28, i29, i30, i31, i32\r\n\nRemote-control command(s):\nREAD:WPAN:MEAS<i>:MEValuation:TRACe:EVMChip[:OFFSet]:AVERage?"}, {"Level"=4, "Class Only"=FALSE, "Identifier"="RSCMPLRWM_ATTR_HIDDEN_READ_MULTIEVAL_EVM_VS_CHIP_MAXIMUM_TRACE_RESULTS", "Descriptive Name"="Read MultiEval EVM vs Chip Maximum Trace Results", "Data Type"=6, "Command"="READ:WPAN:MEAS{instance}:MEV:TRAC:EVMC:MAX?", "Access"=0, "Range Table"="", "Read Callback"="", "Write Callback"="", "Supported Models"="", "Instrument Options"="", "Flags"=8, "Help"="Starts a single-shot measurement and returns the maximum offset EVM vs chip traces. One value per two chips within the PSDU is returned.\n\nReturn values:\n<Reliability>   - Reliability indicator\ndecimal\n\n<EVM>   - Offset error vector magnitude\nfloat\n\nAvailable Repeated Capabilities:\ninstance: i0, i1, i2, i3, i4, i5, i6, i7, i8, i9, i10, i11, i12, i13, i14, i15, i16, i17, i18, i19, i20, i21, i22, i23, i24, i25, i26, i27, i28, i29, i30, i31, i32\r\n\nRemote-control command(s):\nREAD:WPAN:MEAS<i>:MEValuation:TRACe:EVMChip[:OFFSet]:MAXimum?"}, {"Level"=4, "Class Only"=FALSE, "Identifier"="RSCMPLRWM_ATTR_HIDDEN_FETCH_MULTIEVAL_EVM_VS_CHIP_CURRENT_ABSOLUTE_TRACE_RESULTS", "Descriptive Name"="Fetch MultiEval EVM vs Chip Current Absolute Trace Results", "Data Type"=6, "Command"="FETC:WPAN:MEAS{instance}:MEV:TRAC:EVMC:ABS:CURR?", "Access"=0, "Range Table"="", "Read Callback"="", "Write Callback"="", "Supported Models"="", "Instrument Options"="", "Flags"=8, "Help"="Returns the absolute current offset EVM vs chip traces. One value per two chips within the PSDU is returned.\n\nReturn values:\n<Reliability>   - Reliability indicator\ndecimal\n\n<EVM>   - Absolute error vector magnitude\nfloat\n\nAvailable Repeated Capabilities:\ninstance: i0, i1, i2, i3, i4, i5, i6, i7, i8, i9, i10, i11, i12, i13, i14, i15, i16, i17, i18, i19, i20, i21, i22, i23, i24, i25, i26, i27, i28, i29, i30, i31, i32\r\n\nRemote-control command(s):\nFETCh:WPAN:MEAS<i>:MEValuation:TRACe:EVMChip:ABSolute:CURRent?"}, {"Level"=4, "Class Only"=FALSE, "Identifier"="RSCMPLRWM_ATTR_HIDDEN_FETCH_MULTIEVAL_EVM_VS_CHIP_AVERAGE_ABSOLUTE_TRACE_RESULTS", "Descriptive Name"="Fetch MultiEval EVM vs Chip Average Absolute Trace Results", "Data Type"=6, "Command"="FETC:WPAN:MEAS{instance}:MEV:TRAC:EVMC:ABS:AVER?", "Access"=0, "Range Table"="", "Read Callback"="", "Write Callback"="", "Supported Models"="", "Instrument Options"="", "Flags"=8, "Help"="Returns the absolute average offset EVM vs chip traces. One value per two chips within the PSDU is returned.\n\nReturn values:\n<Reliability>   - Reliability indicator\ndecimal\n\n<EVM>   - Absolute error vector magnitude\nfloat\n\nAvailable Repeated Capabilities:\ninstance: i0, i1, i2, i3, i4, i5, i6, i7, i8, i9, i10, i11, i12, i13, i14, i15, i16, i17, i18, i19, i20, i21, i22, i23, i24, i25, i26, i27, i28, i29, i30, i31, i32\r\n\nRemote-control command(s):\nFETCh:WPAN:MEAS<i>:MEValuation:TRACe:EVMChip:ABSolute:AVERage?"}, {"Level"=4, "Class Only"=FALSE, "Identifier"="RSCMPLRWM_ATTR_HIDDEN_FETCH_MULTIEVAL_EVM_VS_CHIP_MAXIMUM_ABSOLUTE_TRACE_RESULTS", "Descriptive Name"="Fetch MultiEval EVM vs Chip Maximum Absolute Trace Results", "Data Type"=6, "Command"="FETC:WPAN:MEAS{instance}:MEV:TRAC:EVMC:ABS:MAX?", "Access"=0, "Range Table"="", "Read Callback"="", "Write Callback"="", "Supported Models"="", "Instrument Options"="", "Flags"=8, "Help"="Returns the absolute maximumt offset EVM vs chip traces. One value per two chips within the PSDU is returned.\n\nReturn values:\n<Reliability>   - Reliability indicator\ndecimal\n\n<EVM>   - Absolute error vector magnitude\nfloat\n\nAvailable Repeated Capabilities:\ninstance: i0, i1, i2, i3, i4, i5, i6, i7, i8, i9, i10, i11, i12, i13, i14, i15, i16, i17, i18, i19, i20, i21, i22, i23, i24, i25, i26, i27, i28, i29, i30, i31, i32\r\n\nRemote-control command(s):\nFETCh:WPAN:MEAS<i>:MEValuation:TRACe:EVMChip:ABSolute:MAXimum?"}, {"Level"=4, "Class Only"=FALSE, "Identifier"="RSCMPLRWM_ATTR_HIDDEN_READ_MULTIEVAL_EVM_VS_CHIP_CURRENT_ABSOLUTE_TRACE_RESULTS", "Descriptive Name"="Read MultiEval EVM vs Chip Current Absolute Trace Results", "Data Type"=6, "Command"="READ:WPAN:MEAS{instance}:MEV:TRAC:EVMC:ABS:CURR?", "Access"=0, "Range Table"="", "Read Callback"="", "Write Callback"="", "Supported Models"="", "Instrument Options"="", "Flags"=8, "Help"="Starts a single-shot measurement and returns the absolute current EVM vs chip traces. One value per two chips within the PSDU is returned.\n\nReturn values:\n<Reliability>   - Reliability indicator\ndecimal\n\n<EVM>   - Absolute error vector magnitude\nfloats\n\nAvailable Repeated Capabilities:\ninstance: i0, i1, i2, i3, i4, i5, i6, i7, i8, i9, i10, i11, i12, i13, i14, i15, i16, i17, i18, i19, i20, i21, i22, i23, i24, i25, i26, i27, i28, i29, i30, i31, i32\r\n\nRemote-control command(s):\nREAD:WPAN:MEAS<i>:MEValuation:TRACe:EVMChip:ABSolute:CURRent?"}, {"Level"=4, "Class Only"=FALSE, "Identifier"="RSCMPLRWM_ATTR_HIDDEN_READ_MULTIEVAL_EVM_VS_CHIP_AVERAGE_ABSOLUTE_TRACE_RESULTS", "Descriptive Name"="Read MultiEval EVM vs Chip Average  Absolute Trace Results", "Data Type"=6, "Command"="READ:WPAN:MEAS{instance}:MEV:TRAC:EVMC:ABS:AVER?", "Access"=0, "Range Table"="", "Read Callback"="", "Write Callback"="", "Supported Models"="", "Instrument Options"="", "Flags"=8, "Help"="Starts a single-shot measurement and returns the absolute average EVM vs chip traces. One value per two chips within the PSDU is returned.\n\nReturn values:\n<Reliability>   - Reliability indicator\ndecimal\n\n<EVM>   - Absolute error vector magnitude\nfloats\n\nAvailable Repeated Capabilities:\ninstance: i0, i1, i2, i3, i4, i5, i6, i7, i8, i9, i10, i11, i12, i13, i14, i15, i16, i17, i18, i19, i20, i21, i22, i23, i24, i25, i26, i27, i28, i29, i30, i31, i32\r\n\nRemote-control command(s):\nREAD:WPAN:MEAS<i>:MEValuation:TRACe:EVMChip:ABSolute:AVERage?"}, {"Level"=4, "Class Only"=FALSE, "Identifier"="RSCMPLRWM_ATTR_HIDDEN_READ_MULTIEVAL_EVM_VS_CHIP_MAXIMUM_ABSOLUTE_TRACE_RESULTS", "Descriptive Name"="Read MultiEval EVM vs Chip Maximum Absolute Trace Results", "Data Type"=6, "Command"="READ:WPAN:MEAS{instance}:MEV:TRAC:EVMC:ABS:MAX?", "Access"=0, "Range Table"="", "Read Callback"="", "Write Callback"="", "Supported Models"="", "Instrument Options"="", "Flags"=8, "Help"="Starts a single-shot measurement and returns the absolute maximum EVM vs chip traces. One value per two chips within the PSDU is returned.\n\nReturn values:\n<Reliability>   - Reliability indicators\ndecimal\n\n<EVM>   - Absolute error vector magnitude\nfloats\n\nAvailable Repeated Capabilities:\ninstance: i0, i1, i2, i3, i4, i5, i6, i7, i8, i9, i10, i11, i12, i13, i14, i15, i16, i17, i18, i19, i20, i21, i22, i23, i24, i25, i26, i27, i28, i29, i30, i31, i32\r\n\nRemote-control command(s):\nREAD:WPAN:MEAS<i>:MEValuation:TRACe:EVMChip:ABSolute:MAXimum?"}, {"Level"=3, "Class Only"=TRUE, "Identifier"="", "Descriptive Name"="IQ Constellation", "Data Type"=0, "Command"="", "Access"=0, "Range Table"="", "Read Callback"="", "Write Callback"="", "Supported Models"="", "Instrument Options"="", "Flags"=0, "Help"="This class contains commands that return the contents of the IQ constellation diagram."}, {"Level"=4, "Class Only"=FALSE, "Identifier"="RSCMPLRWM_ATTR_HIDDEN_FETCH_MULTIEVAL_IQ_ABSOLUTE_TRACE_RESULTS", "Descriptive Name"="Fetch MultiEval IQ Absolute Trace Results", "Data Type"=6, "Command"="FETC:WPAN:MEAS{instance}:MEV:TRAC:IQAB?", "Access"=0, "Range Table"="", "Read Callback"="", "Write Callback"="", "Supported Models"="", "Instrument Options"="", "Flags"=8, "Help"="Returns the absolute IQ constellation diagram (IQ points at each chip interval within the PSDU are returned).\n\nReturn values:\n<Reliability>   - Reliability indicator\ndecimal\n\n<I_1>  <Q_1>  ...  <I_10240>  <Q_10240>   - Pairs of normalized I and Q amplitudes\nfloat\nRange: -2.0 - 2.0\n\nAvailable Repeated Capabilities:\ninstance: i0, i1, i2, i3, i4, i5, i6, i7, i8, i9, i10, i11, i12, i13, i14, i15, i16, i17, i18, i19, i20, i21, i22, i23, i24, i25, i26, i27, i28, i29, i30, i31, i32\r\n\nRemote-control command(s):\nFETCh:WPAN:MEAS<i>:MEValuation:TRACe:IQABsolute?"}, {"Level"=4, "Class Only"=FALSE, "Identifier"="RSCMPLRWM_ATTR_HIDDEN_FETCH_MULTIEVAL_IQ_OFFSET_TRACE_RESULTS", "Descriptive Name"="Fetch MultiEval IQ Offset Trace Results", "Data Type"=6, "Command"="FETC:WPAN:MEAS{instance}:MEV:TRAC:IQOF?", "Access"=0, "Range Table"="", "Read Callback"="", "Write Callback"="", "Supported Models"="", "Instrument Options"="", "Flags"=8, "Help"="Returns the offset IQ constellation diagram (IQ points per two chip intervals within the PSDU are returned).\n\nReturn values:\n<Reliability>   - Reliability indicator\ndecimals\n\n<I_1>  <Q_1>  ...  <I_10240>  <Q_10240>   - Pairs of normalized I and Q amplitudes\nfloat\nRange: -2.0 - 2.0\n\nAvailable Repeated Capabilities:\ninstance: i0, i1, i2, i3, i4, i5, i6, i7, i8, i9, i10, i11, i12, i13, i14, i15, i16, i17, i18, i19, i20, i21, i22, i23, i24, i25, i26, i27, i28, i29, i30, i31, i32\r\n\nRemote-control command(s):\nFETCh:WPAN:MEAS<i>:MEValuation:TRACe:IQOFfset?"}, {"Level"=4, "Class Only"=FALSE, "Identifier"="RSCMPLRWM_ATTR_HIDDEN_READ_MULTIEVAL_IQ_ABSOLUTE_TRACE_RESULTS", "Descriptive Name"="Read MultiEval IQ Absolute Trace Results", "Data Type"=6, "Command"="READ:WPAN:MEAS{instance}:MEV:TRAC:IQAB?", "Access"=0, "Range Table"="", "Read Callback"="", "Write Callback"="", "Supported Models"="", "Instrument Options"="", "Flags"=8, "Help"="Starts a signel-shot measurement and returns the absolute IQ constellation diagram (IQ points at each chip interval within the PSDU are returned).\n\nReturn values:\n<Reliability>   - Reliability indicator\ndecimals\n\n<I_1>  <Q_1>  ...  <I_10240>  <Q_10240>   - Pairs of normalized I and Q amplitudes\nfloat\nRange: -2.0 - 2.0\n\nAvailable Repeated Capabilities:\ninstance: i0, i1, i2, i3, i4, i5, i6, i7, i8, i9, i10, i11, i12, i13, i14, i15, i16, i17, i18, i19, i20, i21, i22, i23, i24, i25, i26, i27, i28, i29, i30, i31, i32\r\n\nRemote-control command(s):\nREAD:WPAN:MEAS<i>:MEValuation:TRACe:IQABsolute?"}, {"Level"=4, "Class Only"=FALSE, "Identifier"="RSCMPLRWM_ATTR_HIDDEN_READ_MULTIEVAL_IQ_OFFSET_TRACE_RESULTS", "Descriptive Name"="Read MultiEval IQ Offset Trace Results", "Data Type"=6, "Command"="READ:WPAN:MEAS{instance}:MEV:TRAC:IQOF?", "Access"=0, "Range Table"="", "Read Callback"="", "Write Callback"="", "Supported Models"="", "Instrument Options"="", "Flags"=8, "Help"="Starts a signel-shot measurement and returns the offset IQ constellation diagram (IQ points per two chip intervals within the PSDU are returned).\n\nReturn values:\n<Reliability>   - Reliability indicator\ndecimals\n\n<I_1>  <Q_1>  ...  <I_10240>  <Q_10240>   - Pairs of normalized I and Q amplitudes\nfloat\nRange: -2.0 - 2.0\n\nAvailable Repeated Capabilities:\ninstance: i0, i1, i2, i3, i4, i5, i6, i7, i8, i9, i10, i11, i12, i13, i14, i15, i16, i17, i18, i19, i20, i21, i22, i23, i24, i25, i26, i27, i28, i29, i30, i31, i32\r\n\nRemote-control command(s):\nREAD:WPAN:MEAS<i>:MEValuation:TRACe:IQOFfset?"}, {"Level"=3, "Class Only"=TRUE, "Identifier"="", "Descriptive Name"="Power Spectral Density", "Data Type"=0, "Command"="", "Access"=0, "Range Table"="", "Read Callback"="", "Write Callback"="", "Supported Models"="", "Instrument Options"="", "Flags"=0, "Help"="This class contains commands that return the contents of the power spectral density diagram."}, {"Level"=4, "Class Only"=FALSE, "Identifier"="RSCMPLRWM_ATTR_HIDDEN_FETCH_MULTIEVAL_PSD_CURRENT_TRACE_RESULTS", "Descriptive Name"="Fetch MultiEval PSD Current Trace Results", "Data Type"=6, "Command"="FETC:WPAN:MEAS{instance}:MEV:TRAC:PSD:CURR?", "Access"=0, "Range Table"="", "Read Callback"="", "Write Callback"="", "Supported Models"="", "Instrument Options"="", "Flags"=8, "Help"="Returns the current power spectral density traces measured using a 100 kHz resolution bandwidth filter. The results are relative to the maximum average spectral power measured within the 1.0 MHz of the carrier frequency. The first and last samples correspond to -12.5 MHz and +12.5 MHz relative to the carrier frequency. The frequency step between two consecutive samples is 31.25 kHz.\n\nReturn values:\n<Reliability>   -  Reliability indicator\ndecimal\n\n<PowSpecDensity>   -  Spectral power\nfloat\nRange: -99.99 -  99.99\n\nAvailable Repeated Capabilities:\ninstance: i0, i1, i2, i3, i4, i5, i6, i7, i8, i9, i10, i11, i12, i13, i14, i15, i16, i17, i18, i19, i20, i21, i22, i23, i24, i25, i26, i27, i28, i29, i30, i31, i32\r\n\nRemote-control command(s):\nFETCh:WPAN:MEAS<i>:MEValuation:TRACe:PSDensity:CURRent[:RELative]?"}, {"Level"=4, "Class Only"=FALSE, "Identifier"="RSCMPLRWM_ATTR_HIDDEN_FETCH_MULTIEVAL_PSD_AVERAGE_TRACE_RESULTS", "Descriptive Name"="Fetch MultiEval PSD Average Trace Results", "Data Type"=6, "Command"="FETC:WPAN:MEAS{instance}:MEV:TRAC:PSD:AVER?", "Access"=0, "Range Table"="", "Read Callback"="", "Write Callback"="", "Supported Models"="", "Instrument Options"="", "Flags"=8, "Help"="Returns the averaget power spectral density traces measured using a 100 kHz resolution bandwidth filter. The results are relative to the maximum average spectral power measured within the 1.0 MHz of the carrier frequency. The first and last samples correspond to -12.5 MHz and +12.5 MHz relative to the carrier frequency. The frequency step between two consecutive samples is 31.25 kHz.\n\nReturn values:\n<Reliability>   -  Reliability indicator\ndecimal\n\n<PowSpecDensity>   -  Spectral power\nfloat\nRange: -99.99 -  99.99\n\nAvailable Repeated Capabilities:\ninstance: i0, i1, i2, i3, i4, i5, i6, i7, i8, i9, i10, i11, i12, i13, i14, i15, i16, i17, i18, i19, i20, i21, i22, i23, i24, i25, i26, i27, i28, i29, i30, i31, i32\r\n\nRemote-control command(s):\nFETCh:WPAN:MEAS<i>:MEValuation:TRACe:PSDensity:AVERage[:RELative]?"}, {"Level"=4, "Class Only"=FALSE, "Identifier"="RSCMPLRWM_ATTR_HIDDEN_FETCH_MULTIEVAL_PSD_MAXIMUM_TRACE_RESULTS", "Descriptive Name"="Fetch MultiEval PSD Maximum Trace Results", "Data Type"=6, "Command"="FETC:WPAN:MEAS{instance}:MEV:TRAC:PSD:MAX?", "Access"=0, "Range Table"="", "Read Callback"="", "Write Callback"="", "Supported Models"="", "Instrument Options"="", "Flags"=8, "Help"="Returns the maximum power spectral density traces measured using a 100 kHz resolution bandwidth filter. The results are relative to the maximum average spectral power measured within the 1.0 MHz of the carrier frequency. The first and last samples correspond to -12.5 MHz and +12.5 MHz relative to the carrier frequency. The frequency step between two consecutive samples is 31.25 kHz.\n\nReturn values:s\n<Reliability>   -  Reliability indicator\ndecimal\n\n<PowSpecDensity>   -  Spectral power\nfloat\nRange: -99.99 -  99.99\n\nAvailable Repeated Capabilities:\ninstance: i0, i1, i2, i3, i4, i5, i6, i7, i8, i9, i10, i11, i12, i13, i14, i15, i16, i17, i18, i19, i20, i21, i22, i23, i24, i25, i26, i27, i28, i29, i30, i31, i32\r\n\nRemote-control command(s):\nFETCh:WPAN:MEAS<i>:MEValuation:TRACe:PSDensity:MAXimum[:RELative]?"}, {"Level"=4, "Class Only"=FALSE, "Identifier"="RSCMPLRWM_ATTR_HIDDEN_READ_MULTIEVAL_PSD_CURRENT_TRACE_RESULTS", "Descriptive Name"="Read MultiEval PSD Current Trace Results", "Data Type"=6, "Command"="READ:WPAN:MEAS{instance}:MEV:TRAC:PSD:CURR?", "Access"=0, "Range Table"="", "Read Callback"="", "Write Callback"="", "Supported Models"="", "Instrument Options"="", "Flags"=8, "Help"="Starts a single-shot measurement and returns the current power spectral density traces measured using a 100 kHz resolution bandwidth filter. The results are relative to the maximum average spectral power measured within the 1.0 MHz of the carrier frequency. The first and last samples correspond to -12.5 MHz and +12.5 MHz relative to the carrier frequency. The frequency step between two consecutive samples is 31.25 kHz.\n\nReturn values:\n<Reliability>   -  Reliability indicator\ndecimal\n\n<PowSpecDensity>   -  Spectral power\nfloat\nRange: -99.99 -  99.99\n\nAvailable Repeated Capabilities:\ninstance: i0, i1, i2, i3, i4, i5, i6, i7, i8, i9, i10, i11, i12, i13, i14, i15, i16, i17, i18, i19, i20, i21, i22, i23, i24, i25, i26, i27, i28, i29, i30, i31, i32\r\n\nRemote-control command(s):\nREAD:WPAN:MEAS<i>:MEValuation:TRACe:PSDensity:CURRent[:RELative]?"}, {"Level"=4, "Class Only"=FALSE, "Identifier"="RSCMPLRWM_ATTR_HIDDEN_READ_MULTIEVAL_PSD_AVERAGE_TRACE_RESULTS", "Descriptive Name"="Read MultiEval PSD Average Trace Results", "Data Type"=6, "Command"="READ:WPAN:MEAS{instance}:MEV:TRAC:PSD:AVER?", "Access"=0, "Range Table"="", "Read Callback"="", "Write Callback"="", "Supported Models"="", "Instrument Options"="", "Flags"=8, "Help"="Starts a single-shot measurement and returns the average power spectral density traces measured using a 100 kHz resolution bandwidth filter. The results are relative to the maximum average spectral power measured within the 1.0 MHz of the carrier frequency. The first and last samples correspond to -12.5 MHz and +12.5 MHz relative to the carrier frequency. The frequency step between two consecutive samples is 31.25 kHz.\n\nReturn values:\n<Reliability>   -  Reliability indicator\ndecimal\n\n<PowSpecDensity>   -  Spectral power\nfloat\nRange: -99.99 -  99.99\n\nAvailable Repeated Capabilities:\ninstance: i0, i1, i2, i3, i4, i5, i6, i7, i8, i9, i10, i11, i12, i13, i14, i15, i16, i17, i18, i19, i20, i21, i22, i23, i24, i25, i26, i27, i28, i29, i30, i31, i32\r\n\nRemote-control command(s):\nREAD:WPAN:MEAS<i>:MEValuation:TRACe:PSDensity:AVERage[:RELative]?"}, {"Level"=4, "Class Only"=FALSE, "Identifier"="RSCMPLRWM_ATTR_HIDDEN_READ_MULTIEVAL_PSD_MAXIMUM_TRACE_RESULTS", "Descriptive Name"="Read MultiEval PSD Maximum Trace Results", "Data Type"=6, "Command"="READ:WPAN:MEAS{instance}:MEV:TRAC:PSD:MAX?", "Access"=0, "Range Table"="", "Read Callback"="", "Write Callback"="", "Supported Models"="", "Instrument Options"="", "Flags"=8, "Help"="Starts a single-shot measurement and returns the maximum power spectral density traces measured using a 100 kHz resolution bandwidth filter. The results are relative to the maximum average spectral power measured within the 1.0 MHz of the carrier frequency. The first and last samples correspond to -12.5 MHz and +12.5 MHz relative to the carrier frequency. The frequency step between two consecutive samples is 31.25 kHz.\n\nReturn values:\n<Reliability>   -  Reliability indicator\ndecimal\n\n<PowSpecDensity>   -  Spectral power\nfloat\nRange: -99.99 -  99.99\n\nAvailable Repeated Capabilities:\ninstance: i0, i1, i2, i3, i4, i5, i6, i7, i8, i9, i10, i11, i12, i13, i14, i15, i16, i17, i18, i19, i20, i21, i22, i23, i24, i25, i26, i27, i28, i29, i30, i31, i32\r\n\nRemote-control command(s):\nREAD:WPAN:MEAS<i>:MEValuation:TRACe:PSDensity:MAXimum[:RELative]?"}, {"Level"=1, "Class Only"=TRUE, "Identifier"="", "Descriptive Name"="Utility", "Data Type"=0, "Command"="", "Access"=0, "Range Table"="", "Read Callback"="", "Write Callback"="", "Supported Models"="", "Instrument Options"="", "Flags"=0, "Help"="Utility settings"}, {"Level"=2, "Class Only"=FALSE, "Identifier"="RSCMPLRWM_ATTR_SYSTEM_VERSION", "Descriptive Name"="System Version", "Data Type"=2, "Command"="SYST:VERSion?", "Access"=0, "Range Table"="", "Read Callback"="", "Write Callback"="", "Supported Models"="", "Instrument Options"="", "Flags"=0, "Help"="Gets system version.\n\nAvailable Repeated Capabilities:\nNone\n\nRemote-control command(s):\nSYSTem:VERSion?"}, {"Level"=2, "Class Only"=FALSE, "Identifier"="RSCMPLRWM_ATTR_SYSTEM_ERROR", "Descriptive Name"="System Error", "Data Type"=2, "Command"="SYST:ERRor?", "Access"=0, "Range Table"="", "Read Callback"="", "Write Callback"="", "Supported Models"="", "Instrument Options"="", "Flags"=0, "Help"="This attribute queries the earliest entry in the error queue, and deletes it after the readout.\n\nAvailable Repeated Capabilities:\nNone\n\nRemote-control command(s):\nSYSTem:ERRor?"}, {"Level"=2, "Class Only"=FALSE, "Identifier"="RSCMPLRWM_ATTR_SYSTEM_ALL_ERRORS", "Descriptive Name"="System All Errors", "Data Type"=2, "Command"="SYST:ERR:ALL?", "Access"=0, "Range Table"="", "Read Callback"="", "Write Callback"="", "Supported Models"="", "Instrument Options"="", "Flags"=0, "Help"="Reads all errors from instrument.\n\nAvailable Repeated Capabilities:\nNone\n\nRemote-control command(s):\nSYSTem:ERRor:ALL?"}, {"Level"=2, "Class Only"=FALSE, "Identifier"="RSCMPLRWM_ATTR_SYSTEM_PRESET", "Descriptive Name"="System Preset", "Data Type"=4, "Command"="SYST:PRES", "Access"=1, "Range Table"="", "Read Callback"="", "Write Callback"="", "Supported Models"="", "Instrument Options"="", "Flags"=0, "Help"="Resets instrument.\n\nAvailable Repeated Capabilities:\nNone\n\nRemote-control command(s):\nSYSTem:PRESet"}, {"Level"=2, "Class Only"=FALSE, "Identifier"="RSCMPLRWM_ATTR_PROCESS_ALL_PREVIOUS_COMMANDS", "Descriptive Name"="Process All Previous Commands", "Data Type"=4, "Command"="*WAI", "Access"=1, "Range Table"="", "Read Callback"="", "Write Callback"="", "Supported Models"="", "Instrument Options"="", "Flags"=0, "Help"="Stops further command processing until all commands sent before *WAI have been executed.\n\nAvailable Repeated Capabilities:\nNone\n\nRemote-control command(s):\n*WAI"}] {"Flags" format="%08b"; "Access" items=["Read Only", "Write Only", "Read/Write"]; "Data Type" items=["Integer 32", "Double", "String", "Boolean", "None", "Integer 64", "RawString"]}
  in  "Supported Models":string[](array[string])=["CMX", "CMP", "CMW"]
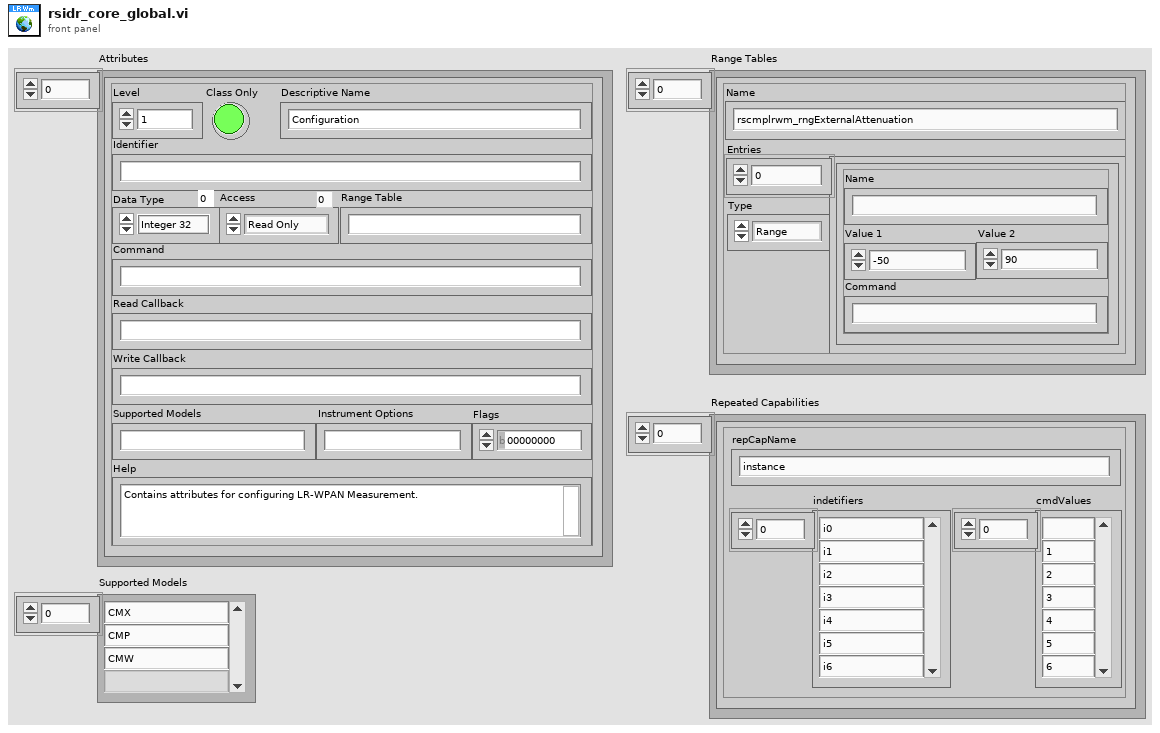
[diagram p1: front panel]
types:
  T1 = typedef "Rohde&Schwarz CMP LR WPAN Measurement.lvlib/rsidr_core.lvlib/type_Input_Format_RepCap.ctl" = cluster{"repCapName":string, "indetifiers":string[], "cmdValues":string[]}
  T2 = typedef "Rohde&Schwarz CMP LR WPAN Measurement.lvlib/rsidr_core.lvlib/type_Input_Format_RangeTable.ctl" = cluster{"Type":u16, "Name":string, "Entries":cluster{"Name":string, "Value 1":dbl, "Value 2":dbl, "Command":string}[]}
  T3 = typedef "Rohde&Schwarz CMP LR WPAN Measurement.lvlib/rsidr_core.lvlib/type_Input_Format_Attribute.ctl" = cluster{"Level":i32, "Class Only":bool, "Identifier":string, "Descriptive Name":string, "Data Type":u16, "Command":string, "Access":u16, "Range Table":string, "Read Callback":string, "Write Callback":string, "Supported Models":string, "Instrument Options":string, "Flags":i32, "Help":string}
diagram:
